vi "IonicsServiceTool.vi"() -> ()   [LabVIEW 2015]
uses:
  Type/_Source Type.ctl
  Type/_Syringe Pump Command.ctl
  Type/_Instrument Model.ctl
  Type/_RT Instrument State.ctl
  Type/_Run State.ctl
  Type/_Log Command.ctl
  Type/_RT Command.ctl
  Type/_RT Configuration 2.ctl
  Type/_PIC Channel.ctl
  Type/_RT Startup Options.ctl
  Type/_RT Instrument 2.ctl
  Type/_Data Operation.ctl
  Type/_Model Family.ctl
  Type/_SaveOption.ctl
  Type/_Board ID.ctl
  Type/_Run Module.ctl
  Type/_Voltage Type.ctl
  Print.ctl
  Type/_Pump Parameter.ctl
  Configuration/_Global Configuration.vi
  <vilib>/Utility/config.llb/Read Key (Path).vi
  <vilib>/Utility/config.llb/Write Key (Path).vi
  <vilib>/Utility/config.llb/Read Key (String).vi
  <vilib>/Utility/config.llb/Write Key (String).vi
  LCDriver/_Global LC Driver.vi
  <vilib>/Utility/config.llb/Read Key (I32).vi
  <vilib>/Utility/NIReport.llb/Append Image to Report (path wrap).vi
  <vilib>/Platform/browser.llb/Open URL in Default Browser (string).vi
  <vilib>/Utility/config.llb/Write Key (I32).vi
  <vilib>/Utility/NIReport.llb/NI_report.lvclass
  <vilib>/Utility/config.llb/NI_LVConfig.lvlib
panel:
  in  "Force Update Oscillators":bool
  out "Version":string
  out "Date/Time":string
  out "SN":string
  in  "Force Update Poles":bool
  out "MS State":T1
  in  "Print":bool
  in  "Options":bool
  in  "Unit":bool
  out "Firmware OK":bool
  out "Intlk/Per OK":bool
  out "Quad/Tune OK":bool=TRUE
  out "SVG OK":bool
  out "Voltage OK":bool
  out "Turbo OK":bool
  in  "Tab Control":T2(tab)
  out "*.ipf Path:":path=path "C:/GIT/EH-Simplicity/firmware-server/Sniffer.900/Ionica Server.ipf"
  in  "Header Info":bool
  out "IP Address":string="172.16.0.2"
  out "Corona":u16
  out "Source 2":u16
  out "Source 1":u16
  out "HSID":u16
  out "Model Name":T3=enum."Simulation (Single Source)"
  out "Serial Number":string="Ion Sniffer 03"
  in  "Refresh":bool
  out "Messages":string
  out "Description":string
  in  "Load Firmware":bool
  out "Current Information:":string[][](table)=[["FW Package Version", "0"], ["RT Firmware Version", "0"], ["FPGA Firmware Version", "0"], ["", ""], ["Instrument Serial #", "-1"], ["Instrument Model", "-1"]]
  out "Number of Power Failures:":u32
  out "Number of Pressure Overload Errors:":u32
  out "Total Number of Errors:":u32
  out "Errors:":string[][](table)=[["0", ""], ["", ""], ["", ""], ["", ""], ["", ""], ["", ""], ["", ""], ["", ""]]
  out "PumpStatus":u16(ring)
  out "Turning":bool
  out "Normal \nOperation":bool
  out "Accel":bool
  out "Decel":bool
  out "Frequency (Hz):":u16(slide) scale=0.0..1000.0
  out "Controller Temperature:":u16(slide) scale=0.0..90.0
  out "Moter Temperature:":u32(slide) scale=0.0..120.0
  out "Bearing Temperature:":u32(slide) scale=0.0..75.0
  out "Pressures:":string[][](table)=[["Foreline Pressure (torr)", "-0.11"], ["Analyzer Pressure (torr)", "1.00E+0"]]
  out "Run Time:":string[][](table)=[["Pump (hours)", ""], ["Days", ""], ["Number of Starts", ""], ["", ""], ["", ""], ["", ""], ["", ""], ["", ""]]
  out "Power:":string[][](table)=[["Voltage (V)", ""], ["Power (W)", ""], ["Current (A)", ""], ["Mean Current (A)", ""], ["Max Current (A)", ""], ["", ""], ["", ""], ["", ""]]
  out "Configuration:":string[][](table)=[["Pump Model", ""], ["Pump Serial Number", ""], ["Controller Model", ""], ["Controller Serial Number", ""], ["Electronics Model", ""], ["Electronic Serial Number", ""], ["Software Version", ""], ["Pump Parameter Set", ""]]
  in  "LBPower":bool
  in  "LBRunTime":bool
  in  "LBError":bool
  in  "LBConfiguration":bool
  in  "LBFreqTemp":bool
  in  "LBUpdateAll":bool
  in  "LBPump":bool
  in  "Update Power":bool
  in  "Update Temp":bool
  in  "Update Pumping":bool
  in  "Update Info":bool
  out "Error History":string[][](table)
  out "Temperatures:":string[][](table)=[["Electronic Drive Temperature", "Pass"], ["Pump Temperature", "Pass"], ["Power Stage Temperature (°C)", "0"], ["Electronics Temperature (°C)", "0"], ["Upper Pump Temperature (°C)", "0"], ["Bearing Temperature (°C)", "0"], ["Motor Temperature (°C)", "0"]]
  out "Power / Current:":string[][](table)=[["Drive Power (W)", "0"], ["Drive Current (A)", "0"]]
  out "Pumping:":string[][](table)=[["Rotational Frequency (Hz)", "0"], ["Rotational Speed (rpm)", "0"]]
  out "Pump Info:":string[][](table)=[["Hardware Version", "0"], ["Firmware Version", "0"], ["Operating Hours (Pump)", "0"], ["Operating Hours (Electronic Drive)", "0"]]
  in  "Turbo Update":bool
  out "Vacuum Readings by Region":string[][](table)=[["Foreline Pressure (torr)", "-0.11"], ["Analyzer Pressure (torr)", "1.00E+0"]]
  in  "Update Error":bool
  out "Main System Current (A)":dbl
  out "Lens Board 2 PS":i32(listbox)=-1
  in  "Set 0 Values":bool
  in  "Load Default Method":bool
  in  "Load Tune File":bool
  in  "Min Voltages":bool
  in  "Max Voltages":bool
  in  "Test Voltages":bool
  in  "Switch Polarity":bool
  out "Main System PS":i32(listbox)=-1
  out "Quad DC PS":i32(listbox)=-1
  out "Lens Board 1 PS":i32(listbox)=-1
  in  "Detector":string[][](table)=[["HED", "", "0.0", "3.014"], ["Horn", "", "0.0", "0.019"], ["DV", "", "0.0", "0.023"], ["Disc", "", "0.0", "2.014"], ["5", "L2 (11)", "0.0", "0.019"], ["6", "PF (12)", "-16.0", "0.019"], ["7", "CCL1 (13)", "0.0", "0.019"], ["8", "CCL2 (14)", "-100.0", "0.019"], ["9", "CC (23)", "-50.0", "0.014"], ["10", "CCAF (10)", "50.0", "0.019"], ["11", "CCL3 (15)", "-52.5", "0.014"], ["12", "CCL4 (16)", "-72.5", "0.014"], ["13", "ID (17)", "-100.0", "0.014"], ["14", "Horn (200)", "5500.0", "-82.090"], ["15", "DV (34)", "1000.0", "-82.773"], ["16", "M1RF (3)", "400.0", "2.161"], ["17", "Disc (32)", "10", "10"]]
  in  "Lens 1":string[][](table)=[["Element", "L1", "M1", "EV", "Spare", "M2", "CC", "Spare", "Spare"], ["Input", "0", "0", "0", "0", "0", "0", "0", "0"], ["Readback", "0", "0", "0", "0", "0", "0", "0", "0"]]
  in  "Lens 2":string[][](table)=[["Element", "CCAF", "L2", "PF", "CCL1", "CCL2", "CCL3", "CCL4", "ID"], ["Input", "", "", "", "", "", "", "", ""], ["Readback", "", "", "", "", "", "", "", ""]]
  out "Source Map":T4={"Ring 2"=0, "Ring 3"=0, "OK 2"=TRUE, "OK 3"=TRUE, "OK 4"=TRUE, "OK 5"=TRUE, "OK 6"=TRUE, "OK 7"=TRUE, "OK 8"=TRUE, "OK 9"=TRUE, "OK 10"=TRUE, "OK 11"=TRUE}
  out "Pressure Readings":string[][](table)=[["Foreline Pressure (torr)", "-0.11"], ["Analyzer Pressure (torr)", "1.00E+0"], ["Plenum Delta P (torr)", "-0.09"], ["Drying Gas Pressure (psi)", "-12.56"], ["Source Gas Pressure (psi)", "-12.56"]]
  in  "Corona/Curtain High Voltage":string[][](table)=[["Corona High Voltage", "0.0", "65535.000", "0"], ["Curtain Cap Voltage", "0.0", "910936.500", "0"]]
  in  "Source Probes":string[][](table)=[["Pillar 1", "None", "0.0", "2791790.869", "0"], ["Pillar 2", "None", "0.0", "2794412.334", "0"]]
  in  "Heaters":string[][](table)=[["1", "HSID", "200.0", "65535.000"], ["2", "P1T", "0.0", "93715.050"], ["3", "P2T", "0.0", "93715.050"]]
  in  "Typical Gas Settings":bool
  in  "Max Gas Settings":bool
  in  "Min Gas Settings":bool
  in  "Gas Flows":string[][](table)=[["1", "DG", "150.0", "316.460"], ["2", "NG1", "200.0", "312.782"], ["3", "HG1", "280.0", "354.817"], ["4", "NG2", "200.0", "0.000"], ["5", "HG2", "280.0", "0.000"], ["6", "CCP", "490", "-477.539"]]
  in  "GotoUPS":bool
  in  "IP Address":string
  in  "Input Value":sgl
  in  "Pump Command":T5=enum."status"
  out "Return Data":string
  in  "SendSyringeCommand":bool
  out "SourceOK":bool
  out "HG2OK":bool
  out "HG1OK":bool
  out "ExhaustOK":bool
  out "DryingGasOK":bool
  out "VacRdy":bool
  out "DoorOK":bool=TRUE
  out "Interlocks":string[][](table)=[["Card Cage Door", ""], ["Vacuum Ready", ""], ["Heating Gas 1", ""], ["Heating Gas 2", ""], ["Drying Gas", ""], ["Exhaust Gas", ""], ["Source Interlock", ""]]
  out "Source 2 Type:":T6=127 items=["None", "ESI", "APCI", "APPI", "MicroSpray"]
  out "Source 1 Type:":T6=127 items=["None", "ESI", "APCI", "APPI", "MicroSpray"]
  in  "FrequencyTuneSetup":bool
  out "Q2 RF Heat Sink Temperatures":string[][](table)=[["Q2 HS1", "-0.481"], ["Q2 HS2", "-0.481"], ["Q2 DC Pole A (18)", "-0.481"], ["Q2 DC Pole B (19)", "-0.481"]]
  out "Q1 RF Heat Sink Temperatures":string[][](table)=[["Q1 HS1", "-0.481"], ["Q1 HS2", "-0.481"], ["Q2 DC Pole A (18)", "-0.481"], ["Q2 DC Pole B (19)", "-0.481"]]
  out "M1 RF Heat Sink Temperatures":string[][](table)=[["M1 HS1", "-0.481"], ["M1 HS2", "-0.481"], ["Q2 DC Pole A (18)", "-0.481"], ["Q2 DC Pole B (19)", "-0.481"]]
  out "New Frequence":dbl=1.1064999969676137 format="%.4f"
  out "Old Frequency":dbl=1.1064999969676137 format="%.4f"
  in  "Adjust Cal Tables":bool
  out "M1RF Readback":dbl
  in  "M1RF":dbl=400.0 format="%#.3f"
  in  "Update PM":bool
  in  "Q2 Park Mass":dbl=400.0 format="%#.3f"
  in  "Q1 Park Mass":dbl=400.0 format="%#.3f"
  out "Q2 Total":dbl=157.94015025000002
  out "Q1 Total":dbl=157.94015025000002
  out "Q2 (VDC)":dbl=157.94015025000002
  out "Q1 (VDC)":dbl=157.94015025000002
  in  "Q2 DC Inputs":string[][](table)=[["600.00"], ["0.00"], ["0.00"]]
  in  "Q1 DC Inputs":string[][](table)=[["600.00"], ["0.00"], ["0.00"]]
  out "DC Pole Read Back":string[][](table)=[["Q1 DC Pole A", "-0.481"], ["Q1 DC Pole B", "-0.481"], ["Q2 DC Pole A", "-0.481"], ["Q2 DC Pole B", "-0.481"]]
  in  "Oscillator Settings":string[][](table)=[["M1RF", "66529043", "10", "10", "0.4", "1.5490", "2.256", "1.5490"], ["Q1RF", "47523813", "10", "10", "0.6", "1.1065", "-0.645", "1.1065"], ["Q2RF", "47523813", "10", "10", "0.6", "1.1065", "7.339", "1.1065"]]
  in  "Pos/Neg":enum32{"Positive", "Negative"}(radio)
  in  "Pole Swap Options Negative":T7
  in  "Pole Swap Options Positive":T7
  in  "Table Choice":T8(radio)
  out "Table 4":T9 caption="Q2 -ve Mass Calibration Table"
  out "Table 2":T9 caption="Q2 +ve Mass Calibration Table"
  out "Table 3":T9 caption="Q1 -ve Mass Calibration Table"
  out "Table 1":T9 caption="Q1 +ve Mass Calibration Table"
  in  "Edit Config":bool
  in  "Edit ADC":bool
  in  "View Config":bool
  in  "Export ADC":bool
  out "ADC List":i32(listbox)=130
  in  "Run":bool
  in  "Cancel":bool
  out "Progress Bar":u8(slide)=1 scale=0.0..100.0
  out "LoadedTable":bool
  in  "Tune File":path=path "C:/GIT/EH-Simplicity/firmware-server/Sniffer.900/InternalTools/DEFAULT_SETTINGS.d2m"
  in  "SG Input":dbl[](array[numeric])=[40.0, 0.0, 0.0, 0.0, 0.0, 0.0, 0.0, 200.0, 0.0, 0.0, 0.0, 0.0, 0.0, 0.0]
  in  "VoltageInput":dbl[](array[numeric])=[0.0, 0.0, 0.0, 0.0, 0.0, -16.0, 0.0, -100.0, -50.0, 50.0, -52.5, -72.5, -100.0, 5500.0, 1000.0, 400.0, 10.0, 0.0, 0.0]
  out "Quit":bool=TRUE
  out "Running":bool
  out "Ion Path":T10={"OK 1"=TRUE, "OK 2"=TRUE, "OK 3"=TRUE, "OK 4"=TRUE, "OK 5"=TRUE, "OK 6"=TRUE, "OK 7"=TRUE, "OK 8"=TRUE, "OK 9"=TRUE, "OK 10"=TRUE, "OK 15"=TRUE, "OK 20"=TRUE, "OK 16"=TRUE, "OK 11"=TRUE, "OK 17"=TRUE, "OK 18"=TRUE, "OK 19"=TRUE, "OK 12"=TRUE, "OK 13"=TRUE, "Selected 1"="Selected", "Selected 2"="Selected", "Selected 3"="Selected", "Selected 4"="Selected", "Selected 5"="Selected", "Selected 6"="Selected", "Selected 7"="Selected", "Selected 8"="Selected", "Selected 9"="Selected", "Selected 10"="Selected", "Selected 15"="Selected", "Selected 20"="Selected", "Selected 16"="Selected", "Selected 11"="Selected", "Selected 17"="Selected", "Selected 18"="Selected", "Selected 19"="Selected", "Selected 12"="Selected", "Selected 13"="Selected", "Ring 2"=0, "Ring 3"=0, "OK 14"=TRUE, "Selected 14"="Selected"}
  out "IonPathMap":enum32{"0", "200", "100"}(tab)
  # "PIC Firmware Version"
  # "It will take about 70s\nto complete Update All."
  # "Syringe Pump Control"
  # "UPS"
  # "V"
  # "Polarity"
  # "Pole Orientation"
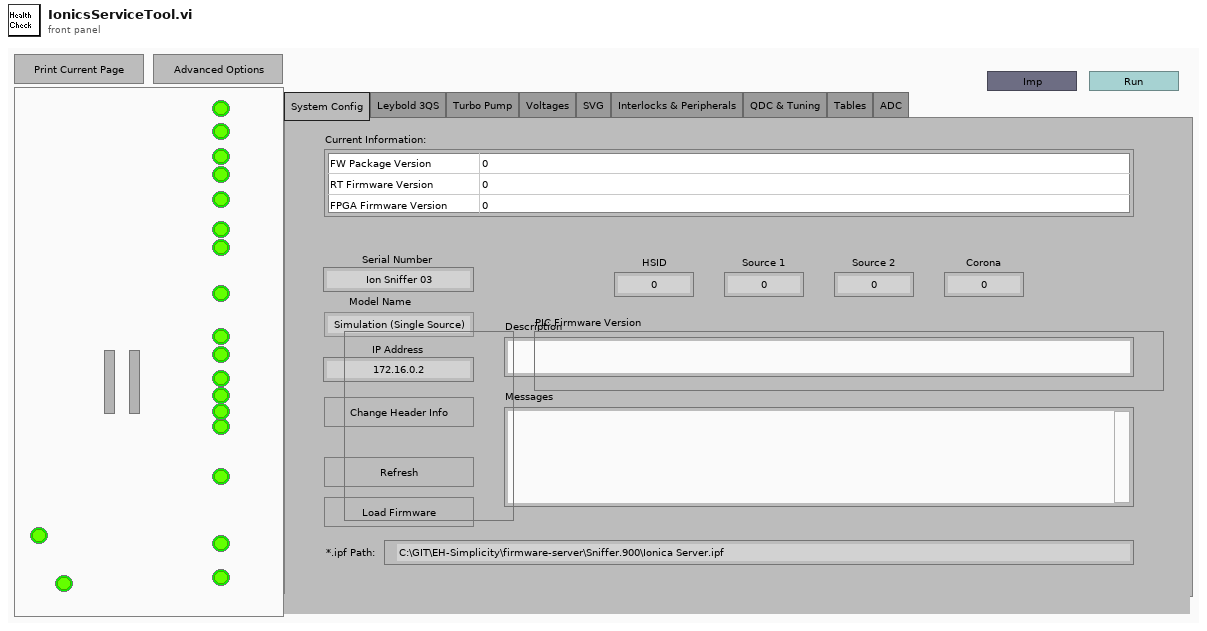
[diagram p1: front panel]
types:
  T1 = typedef "_RT Instrument State.ctl" = enum16{"Initializing", "Mass Spectrometer is Off", "Starting Up", "Turning Power Off", "Going to Standby", "Roughing Pump Ready", "Turning Turbo Off", "Turbo Startup", "Turbopump Ready", "Checking Vacuum", "Going to Ready", "Ready", "Running", "Source Standby", "Lost Communication", "Shutting Down", "Fault", "24V Standby", "Go to 24V Standby", "Turbopump Ready-Waiting"}
  T2 = enum32{"System Config", "Leybold 3QS", "Turbo Pump", "Voltages", "SVG", "Interlocks & Peripherals", "QDC & Tuning", "Tables", "ADC"}
  T3 = typedef "_Instrument Model.ctl" = enum16{"QSight 110", "QSight 120", "QSight 210", "QSight 220", "IONICS 3Q 110", "IONICS 3Q 120", "IONICS 3Q 210", "IONICS 3Q 220", "IONICS 3Q 310", "IONICS 3Q 320", "Simulation (Single Source)", "Simulation (Dual Source)"}
  T4 = cluster{"Ring 2":u16, "Ring 3":u16, "OK 2":bool, "OK 3":bool, "OK 4":bool, "OK 5":bool, "OK 6":bool, "OK 7":bool, "OK 8":bool, "OK 9":bool, "OK 10":bool, "OK 11":bool}
  T5 = typedef "_Syringe Pump Command.ctl" = enum16{"start", "stop", "pause", "restart", "help", "set units", "set diameter", "set rate", "set time", "set volume", "set delay", "save setting", "read limit parameter", "view parameter", "status"}
  T6 = typedef "_Source Type.ctl" = i8
  T7 = cluster{"Q1 A":bool, "Q1 B":bool, "Q2 A":bool, "Q2 B":bool}
  T8 = enum32{"Calibration", "Low Resolution", "Unit Resolution", "High Resolution"}
  T9 = cluster{"Graph":cluster{"all rows":dbl[], "all rows":dbl[]}, "Table":string[][]}
  T10 = cluster{"OK 1":bool, "OK 2":bool, "OK 3":bool, "OK 4":bool, "OK 5":bool, "OK 6":bool, "OK 7":bool, "OK 8":bool, "OK 9":bool, "OK 10":bool, "OK 15":bool, "OK 20":bool, "OK 16":bool, "OK 11":bool, "OK 17":bool, "OK 18":bool, "OK 19":bool, "OK 12":bool, "OK 13":bool, "Selected 1":string, "Selected 2":string, "Selected 3":string, "Selected 4":string, "Selected 5":string, "Selected 6":string, "Selected 7":string, "Selected 8":string, "Selected 9":string, "Selected 10":string, "Selected 15":string, "Selected 20":string, "Selected 16":string, "Selected 11":string, "Selected 17":string, "Selected 18":string, "Selected 19":string, "Selected 12":string, "Selected 13":string, "Ring 2":u16, "Ring 3":u16, "OK 14":bool, "Selected 14":string}
  T11 = enum32{"invalid app kind", "Development System", "Run Time System", "Student Edition", "Embedded LabVIEW", "Evaluation", "Custom"}
  T12 = enum8{"Enabled", "Disabled", "Disabled and Grayed Out"}
  T13 = typedef "_Run State.ctl" = enum16{"Init", "Update", "Start", "End", "Error"}
  T14 = typedef "_Log Command.ctl" = enum16{"No Command", "Open", "Read", "Write", "Close", "Check Size"}
  T15 = typedef "_RT Command.ctl" = enum16{"xml Start Run", "xml Start Actual Run", "xml Stop Run", "xml Runtime Update", "xml Get Status", "xml Get Table", "xml Set Table", "xml Get Configuration", "xml System Status", "xml Set LC Input Logic", "xml Get Data", "xml Get Info", "Start", "StartActualRun", "Stop", "Runtime Update", "Get Data", "Get Info", "Get Status", "Get Param", "Get Config", "Get Table", "Read ADC", "Set Oscillator", "Update Config", "Update Table", "Set All Pol", "Set Pol and DC", "Set Max Mass", "Toggle RP", "Toggle EL", "Set PIC", "Initialize Turbo", "Send Turbo Comm", "Close Turbo", "P1", "P2", "P3", "Send Serial", "Set LC Out", "Get LC In", "Read VAC", "Test Table", "Toggle Power", "Get Startup", "Set Startup", "Get ADC Table", "Set ADC Table", "Get Brief Status", "Get Detail Status", "Auxiliary Update", "Set CC Logics", "Set CC Input Logics", "Ignore Error", "invalid"}
  T16 = enum16{"Use Dialog", "Temporary File", "My Tables"}
  T17 = typedef "_PIC Channel.ctl" = enum16{"Corona +HV", "Corona -HV", "HSID Temp", "Time Const 1", "Curtain Cap +HV", "Curtain Cap -HV", "Time Const 2", "Source 1 +HV", "Source 1 -HV", "Source 1 Temp", "Time Const 3", "Source 2 +HV", "Source 2 -HV", "Source 2 Temp", "Time Const 4"}
  T18 = typedef "_RT Instrument 2.ctl" = cluster{"Table":T19[], "Instrument":string[]}
  T19 = typedef "_RT Configuration 2.ctl" = cluster{"Name":string, "Ch#":u8, "Min":dbl, "Max":dbl, "Def+":dbl, "Def-":dbl, "Offset":dbl, "Slope":dbl, "Type":u8, "Description":string, "SettleT":dbl}
  T20 = cluster{"top":dbl, "left":dbl, "right":dbl, "bottom":dbl}
  T21 = typedef "Print.ctl" = cluster{"Picture Name":string, "VI Reference":refnum<vi>}
  T22 = enum16{"Standard Report", "HTML", "Word", "Excel"}
  T23 = typedef "_Data Operation.ctl" = enum8{"Initialize", "Get Data", "Set Data", "Close"}
  T24 = typedef "_SaveOption.ctl" = enum16{"Use Dialog", "Temporary File", "My Tables", "Full Path"}
  T25 = typedef "_Pump Parameter.ctl" = enum16{"Turn Pump Motor On", "Turn Pump Motor Off", "Read Pump Oil Deficiency", "Read Rotation Switch Point Attained", "Read Ele. Drive Over Temperature", "Read Pump Over Temperature", "Read Set Rotation Speed Attained", "Read Turbopump Accelerates", "Read Actual Rotation Speed in Hz", "Read Motor Current in A", "Read Operating Hours in h", "Read Motor Voltage in V", "Read Motor Power in W", "Set Rotation Speed Switchpoint in %", "Clear Error", "Read Error Code", "Read Bearing Temperature", "Read Hardware Version", "Read Firmware Version", "Read Operating Hours (Drive)", "Read Rotational Speed (rpm)", "Read Power Stage Temperature", "Read Electronics Temperature", "Read Upper Pump Temperature", "Read Motor Temperature", "Read Error Code History, 1", "Read Error Code History, 2", "Read Error Code History, 3", "Read Error Code History, 4", "Read Error Code History, 5", "Read Error Code History, 6", "Read Error Code History, 7", "Read Error Code History, 8", "Read Error Code History, 9", "Read Error Code History, 10"}
  T26 = enum32{"existing file", "new file", "new or existing file", "existing dir", "new dir", "new or existing dir", "existing file (use LLBs)", "new file (use LLBs)", "new or existing file (use LLBs)", "new or existing file or directory (use LLBs)"}
  T27 = enum32{"Leybold 3QS", "Pfeiffer Pump", "Voltages", "SVG", "Interlocks & Peripherals", "FW Manager", "QDC & Tuning", "Tables", "ADC"}
  T28 = cluster{"Source Map":refnum<vi>, "Ion Path":refnum<vi>, "Lens 1":refnum<vi>, "Lens 2":refnum<vi>, "Detector":refnum<vi>, "Main System PS":refnum<vi>, "Lens Board 1 PS":refnum<vi>, "Quad DC PS":refnum<vi>, "Gas Flows":refnum<vi>, "Heaters":refnum<vi>, "Source Probes":refnum<vi>, "Corona/Curtain High Voltage":refnum<vi>, "Pressure Readings":refnum<vi>, "DC Pole Read Back":refnum<vi>, "Lens Board 2 PS":refnum<vi>, "M1 RF Heat Sink Temperatures":refnum<vi>, "Q1 RF Heat Sink Temperatures":refnum<vi>, "Q2 RF Heat Sink Temperatures":refnum<vi>}
  T29 = typedef "NI_LVConfig.lvlib/Config Data RefNum.ctl" = refnum<k1>
  T30 = typedef "_LC Type.ctl" = enum16{"No LC", "Spark"}
  T31 = typedef "_RT Startup Options.ctl" = cluster{"Door":bool, "Curtain":bool, "Pressure":bool, "Turbo":bool, "SysPoll":bool, "GasFlag":bool, "SourceExhaust":bool}
  T32 = cluster{"Configuration 2":T18, "FrequencyTune":bool, "CalAjusted":bool, "Update":bool, "Running":bool, "ADC Table":T19[]}
  T33 = typedef "_Model Family.ctl" = u16
  T34 = typedef "_Board ID.ctl" = u16
  T35 = typedef "_Run Module.ctl" = u16
  T36 = cluster{"trimmed string":string, string, "selected path":path, "Source":enum32{"RT Target", "Folder"}}
  T37 = typedef "_Voltage Type.ctl" = u16
  T38 = cluster{"Frequency":u16, "Decel":bool, "Accel":bool, "Normal \nOperation":bool, "Turning":bool, "BearingTemp":u32, "MotorTemp":u32, "ControllerTemp":u16, "PumpStatus":u16, "NumErrors":u32, "NumOverload":u32, "NumFailure":u32}
  T39 = typedef "imagedata.ctl" = cluster{"image type":i32, "image depth":i32, "image":u8[], "mask":u8[], "colors":u32[], "Rectangle":cluster{"left":i16, "top":i16, "right":i16, "bottom":i16}}
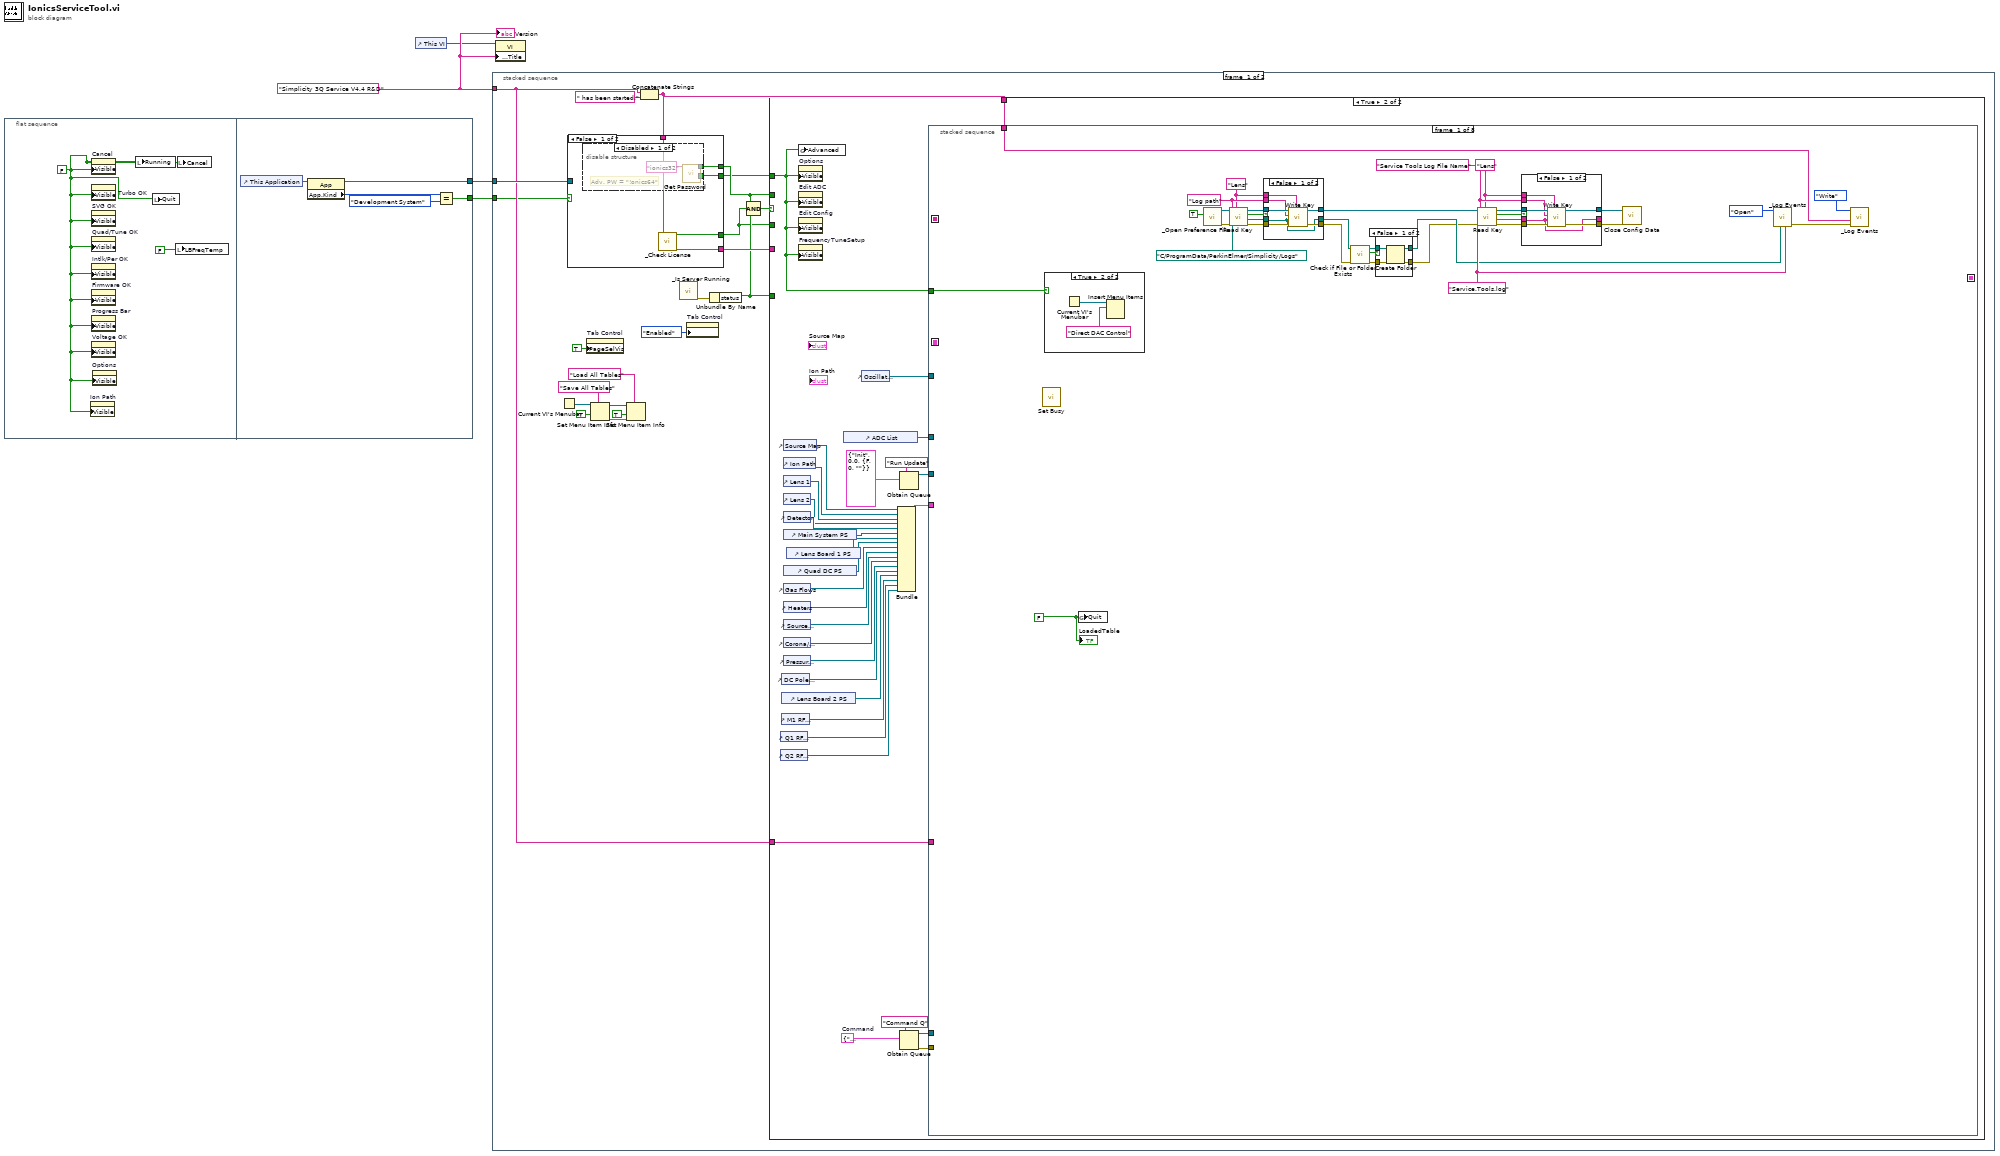
[diagram p0: block diagram]
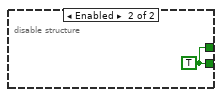
[diagram p2: hidden frame]
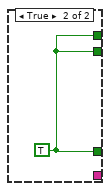
[diagram p3: hidden frame]
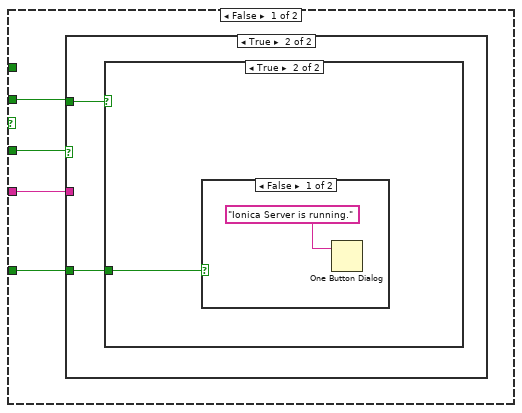
[diagram p4: hidden frame]
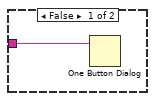
[diagram p5: hidden frame]
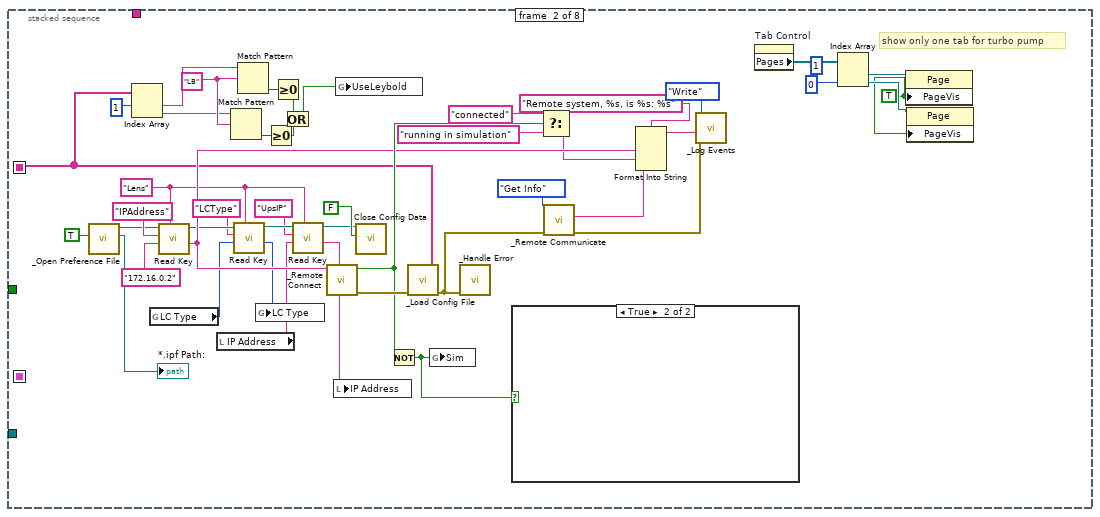
[diagram p12: hidden frame]
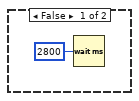
[diagram p13: hidden frame]
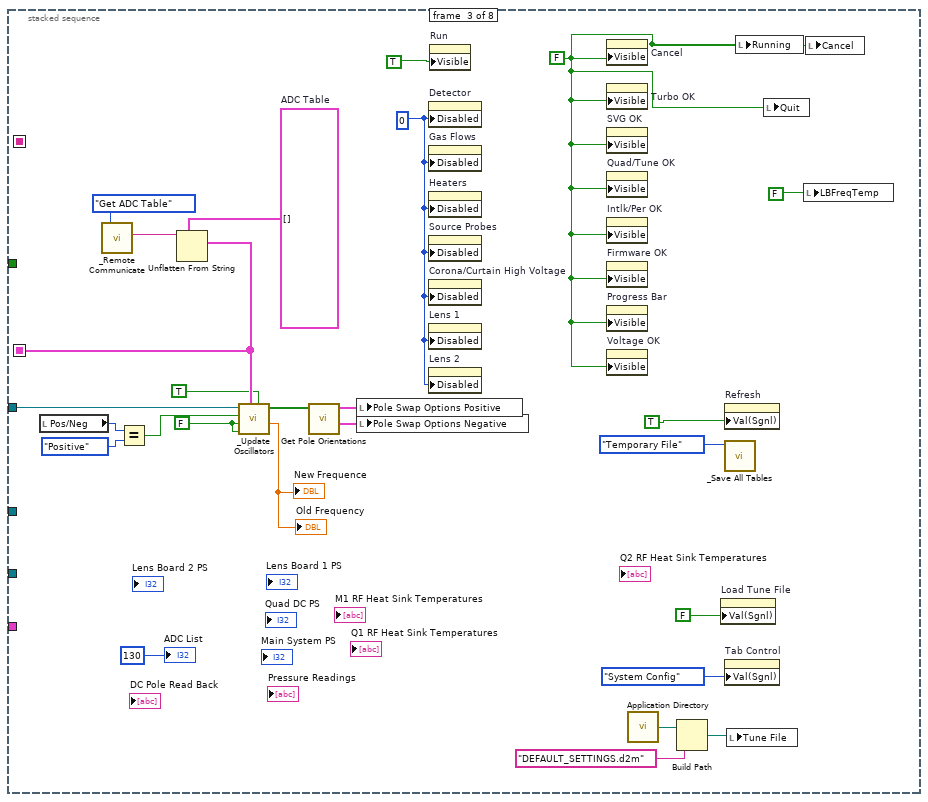
[diagram p14: hidden frame]
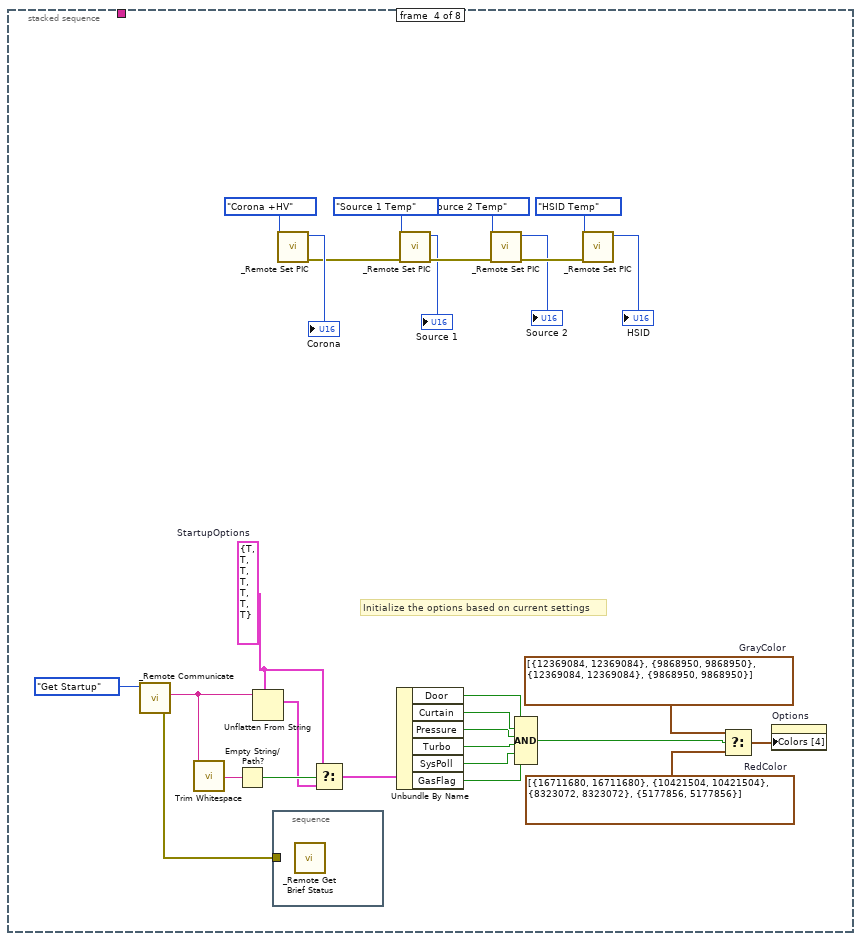
[diagram p15: hidden frame]
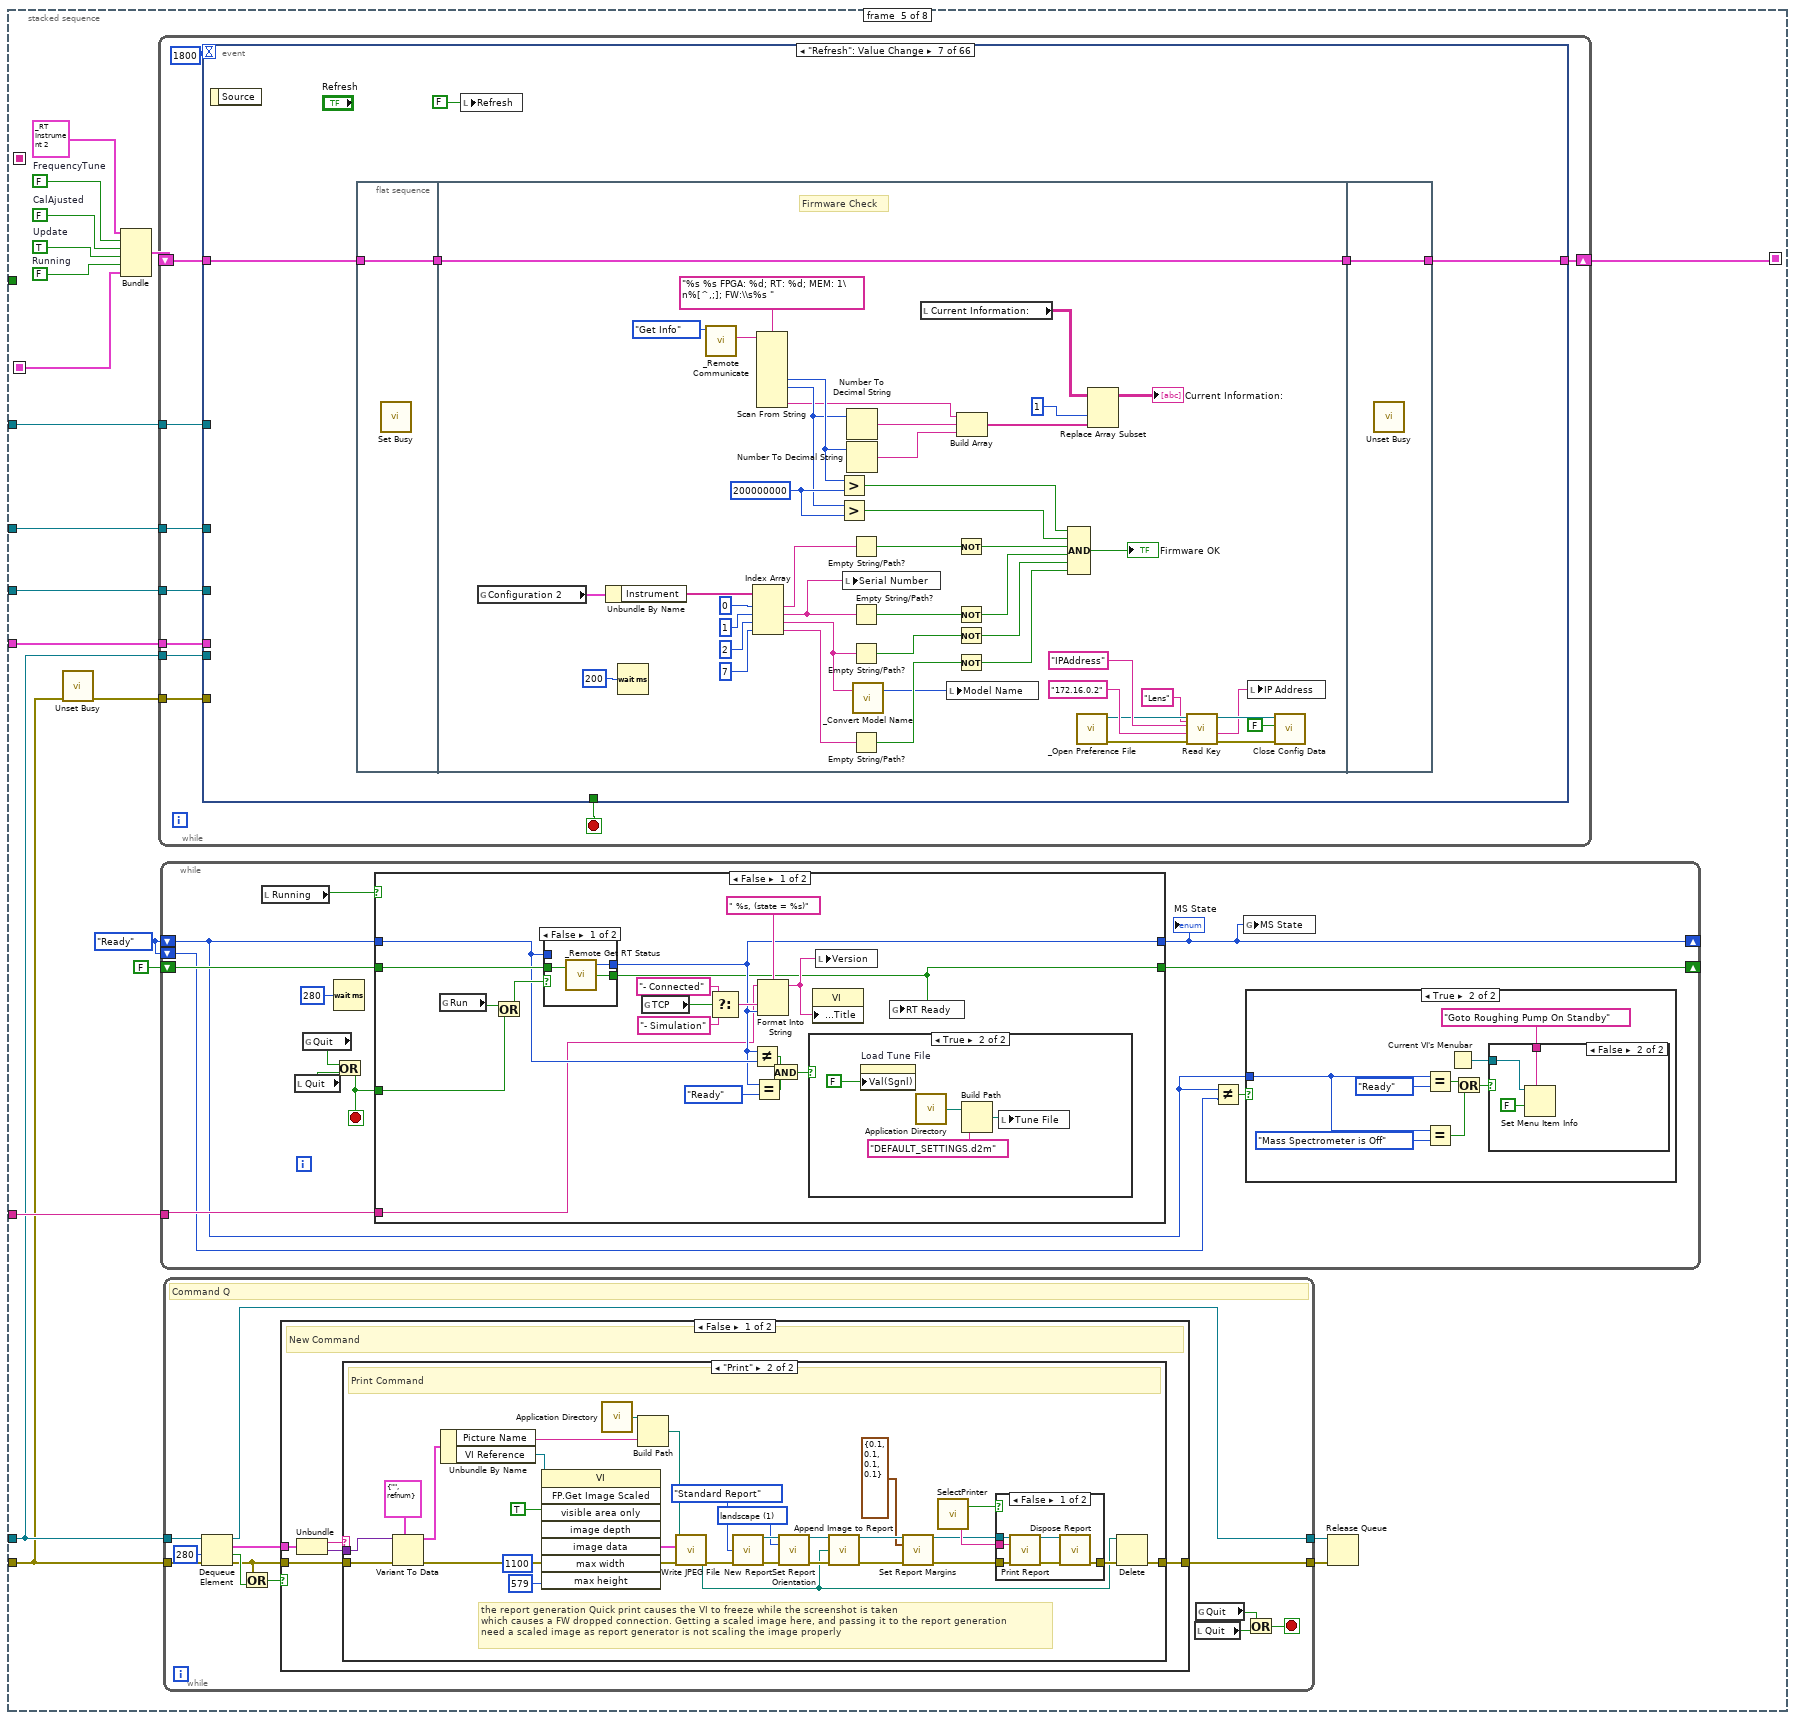
[diagram p16: hidden frame]
diagram:
  w2 = "Simplicity 3Q Service V4.4 R&D" ("string")
  n1 = flat-sequence {
    tunnel: [w9] -> w4
    tunnel: [w8] -> w3
    frame #0 {
      w5 = FALSE ("Unit")
      n2 = property on="Ion Path" class="Clust (strict)"("Visible"=w5) -> ()  [unwired: 2 in, 2 out]
      n3 = property on="Cancel" class="Bool (strict)"("Visible"=w5) -> ()  [unwired: 2 in, 2 out]
      n4 = property on="Turbo OK" class="Bool (strict)"("Visible"=w5) -> ()  [unwired: 2 in, 2 out]
      n5 = property on="SVG OK" class="Bool (strict)"("Visible"=w5) -> ()  [unwired: 2 in, 2 out]
      n6 = property on="Quad/Tune OK" class="Bool (strict)"("Visible"=w5) -> ()  [unwired: 2 in, 2 out]
      n7 = property on="Intlk/Per OK" class="Bool (strict)"("Visible"=w5) -> ()  [unwired: 2 in, 2 out]
      n8 = property on="Firmware OK" class="Bool (strict)"("Visible"=w5) -> ()  [unwired: 2 in, 2 out]
      n9 = property on="Progress Bar" class="Slide (strict)"("Visible"=w5) -> ()  [unwired: 2 in, 2 out]
      n10 = property on="Voltage OK" class="Bool (strict)"("Visible"=w5) -> ()  [unwired: 2 in, 2 out]
      n11 = property on="Options" class="Bool"("Visible"=w5) -> ()  [unwired: 2 in, 2 out]
      n12 = local write "Running"(w5) -> ()
      n13 = local write "Quit"(w5) -> ()
      n14 = local write "LBFreqTemp"(FALSE ("LBFreqTemp")) -> ()
      n15 = local write "Cancel"(w5) -> ()
    }
    frame #1 {
      n16 = control-ref of="This Application"() -> (w7:refnum<vi>)
      n17 = property class="App"(reference=w7) -> (reference out=w8:refnum<vi>, "App.Kind"=w10:T11)  [unwired: 1 in, 1 out]
      n18 = Equal?(x=w10, y=T11."Development System") -> (x = y?=w9:bool)
    }
  }
  n19 = control-ref of="This VI"() -> (w1:refnum<vi>)
  n20 = stacked-sequence {
    tunnel: w4 -> [w12 w1712]
    tunnel: w3 -> [w25 _]
    tunnel: w2 -> [w22 _]
    frame #0 {
      n21 = Current VI's Menubar() -> (w19:refnum<k9>)
      n22 = property on="Tab Control" class="TabCtl (strict)"("PageSelVis"=TRUE ("Page Selector Visible")) -> ()  [unwired: 2 in, 2 out]
      n23 = Set Menu Item Info(7:"Save All Tables" ("item tag"), 9:TRUE ("enabled"), 11:w19) -> (0:w15:errorcluster, 3:w16:refnum<k9>)  [unwired: 4 in]
      n24 = Set Menu Item Info(7:"Load All Tables" ("item tag"), 8:w15, 9:TRUE ("enabled"), 11:w16) -> ()  [unwired: 3 in, 2 out]
      n25 = Concatenate Strings(w22, " has been started." ("string")) -> (w24:string)
      n26 = case shown="False" w12 {
        tunnel: w24 -> [w37 _]
        tunnel: [w36 _] -> w31
        tunnel: [w35 w42] -> w30
        tunnel: [w34 w42] -> w29
        tunnel: [w33 w42] -> w26
        tunnel: w25 -> [_ _]
        frame False {
          n27 = disable-structure shown="Disabled" {
            disable-tunnel: [w39 w41] -> w35
            disable-tunnel: [w38 w41] -> w34
            frame Disabled {
              # "Adv. PW = \"!onics64\""
              n28 = call "Get Password.vi"("IonSniffer777"="ionics32") -> ("Advanced"=w38:bool, "Valid"=w39:bool)  [unwired: 5 out]
            }
            frame Enabled {
              w41 = TRUE ("Advanced")
            }
          }
          n29 = call "_Check License.vi"("ApplicationName"=w37) -> ("Reason"=w36:string, "Valid"=w33:bool)  [unwired: 5 out]
        }
        frame True {
          w42 = TRUE ("Valid")
        }
      }
      n30 = call "_Is Server Running.vi"() -> ("error out"=w28:errorcluster)  [unwired: 6 in, 1 out]
      n31 = property on="Tab Control" class="TabCtl (strict)"("DisabledEnum"=T12."Enabled" ("Disabled")) -> ()  [unwired: 2 in, 2 out]
      n32 = Unbundle By Name(w28) -> ("status"=w27:bool)
      n33 = Compound Arithmetic op=AND(w30, w26, w27) -> (w32:bool)
      n34 = case shown="True" w32 {
        tunnel: w24 -> [_ w66]
        tunnel: w26 -> [w46 _]
        tunnel: w31 -> [w45 _]
        tunnel: w30 -> [w44 _]
        tunnel: w29 -> [_ w57]
        tunnel: w27 -> [w43 _]
        tunnel: w22 -> [_ w56]
        frame False {
          n35 = case shown="True" w46 {
            tunnel: w45 -> [w47 _]
            tunnel: w44 -> [_ w49]
            tunnel: w43 -> [_ w48]
            frame False {
              n36 = One Button Dialog(message=w47) -> ()  [unwired: 2 out]
            }
            frame True {
              n37 = case shown="True" w49 {
                tunnel: w48 -> [_ w50]
                frame False {
                }
                frame True {
                  n38 = case shown="False" w50 {
                    frame False {
                      n39 = One Button Dialog(message="Ionica Server is running.") -> ()  [unwired: 2 out]
                    }
                    frame True {
                    }
                  }
                }
              }
            }
          }
        }
        frame True {
          w54 = cluster{"Command":string, "Data":variant} {"Command"="", "Data"=variant}  # Command
          n40 = control-ref of="Q1 RF Heat Sink Temperatures"() -> (w59:refnum<vi>)
          n41 = control-ref of="Q2 RF Heat Sink Temperatures"() -> (w58:refnum<vi>)
          n42 = control-ref of="Lens Board 2 PS"() -> (w61:refnum<vi>)
          n43 = control-ref of="DC Pole Read Back"() -> (w67:refnum<vi>)
          n44 = control-ref of="M1 RF Heat Sink Temperatures"() -> (w60:refnum<vi>)
          n45 = control-ref of="Ion Path"() -> (w63:refnum<vi>)
          n46 = control-ref of="Lens 1"() -> (w64:refnum<vi>)
          n47 = control-ref of="Lens 2"() -> (w65:refnum<vi>)
          n48 = control-ref of="Detector"() -> (w79:refnum<vi>)
          n49 = control-ref of="Main System PS"() -> (w78:refnum<vi>)
          n50 = control-ref of="Quad DC PS"() -> (w77:refnum<vi>)
          n51 = control-ref of="Gas Flows"() -> (w73:refnum<vi>)
          n52 = control-ref of="Heaters"() -> (w72:refnum<vi>)
          n53 = control-ref of="Source Probes"() -> (w71:refnum<vi>)
          n54 = control-ref of="Corona/Curtain High Voltage"() -> (w70:refnum<vi>)
          n55 = control-ref of="Pressure Readings"() -> (w69:refnum<vi>)
          n56 = control-ref of="Source Map"() -> (w62:refnum<vi>)
          n57 = control-ref of="Lens Board 1 PS"() -> (w76:refnum<vi>)
          n58 = global write "_Global Configuration.vi" "Advanced"(w57) -> ()
          n59 = property on="Options" class="Bool"("Visible"=w57) -> ()  [unwired: 2 in, 2 out]
          n60 = property on="Edit ADC" class="Bool"("Visible"=w57) -> ()  [unwired: 2 in, 2 out]
          n61 = property on="Edit Config" class="Bool"("Visible"=w57) -> ()  [unwired: 2 in, 2 out]
          n62 = property on="FrequencyTuneSetup" class="Bool (strict)"("Visible"=w57) -> ()  [unwired: 2 in, 2 out]
          n63 = control-ref of="ADC List"() -> (w74:refnum<vi>)
          n64 = control-ref of="Oscillator Settings"() -> (w68:refnum<vi>)
          n65 = Bundle("Source Map"=w62, "Ion Path"=w63, "Lens 1"=w64, "Lens 2"=w65, "Detector"=w79, "Main System PS"=w78, "Lens Board 1 PS"=w76, "Quad DC PS"=w77, "Gas Flows"=w73, "Heaters"=w72, "Source Probes"=w71, "Corona/Curtain High Voltage"=w70, "Pressure Readings"=w69, "DC Pole Read Back"=w67, "Lens Board 2 PS"=w61, "M1 RF Heat Sink Temperatures"=w60, "Q1 RF Heat Sink Temperatures"=w59, "Q2 RF Heat Sink Temperatures"=w58) -> (w75:T28)  [unwired: 1 out]
          n66 = Obtain Queue(name (unnamed)="Run Update", element data type=cluster{T13, dbl, "error out":errorcluster} {enum."Init", 0.0, "error out"={"status"=FALSE, "code"=0, "source"=""}}) -> (queue out=w80:refnum<queue>)  [unwired: 3 in, 2 out]
          n67 = Obtain Queue(name (unnamed)="Command Q", element data type=w54) -> (queue out=w53:refnum<queue>, error out=w52:errorcluster)  [unwired: 3 in, 1 out]
          n68 = stacked-sequence {
            seq-local: [_ _ w209 _ _ _ _ _] -> [_ _ _ _ w257 _ _ _]
            seq-local: [_ w160 _ _ _ _ _ _] -> [_ _ _ _ _ w1652 _ _]
            seq-local: [_ _ _ _ w255 _ _ _] -> [_ _ _ _ _ w1596 _ _]
            tunnel: w80 -> [_ _ _ _ w265 w1658 _ _]
            tunnel: w75 -> [_ _ _ _ w261 _ _ _]
            tunnel: w74 -> [_ _ _ _ w260 _ _ _]
            tunnel: w68 -> [_ _ w214 _ w259 _ _ _]
            tunnel: w66 -> [w83 _ _ _ _ _ _ _]
            tunnel: w57 -> [w114 _ _ _ _ _ _ _]
            tunnel: w56 -> [_ _ _ _ w252 _ _ _]
            tunnel: w53 -> [_ _ _ _ w251 _ _ _]
            tunnel: w52 -> [_ _ _ _ w248 _ _ _]
            frame #0 {
              w113 = "Service.Tools.log" ("default value")
              w103 = "Service Tools Log File Name" ("key")
              w102 = "Lens" ("section")
              w97 = "Log path" ("key")
              w96 = "Lens" ("section")
              w115 = FALSE ("Quit")
              n69 = call <vilib>:"Set Busy.vi"() -> ()  [unwired: 4 in, 8 out]
              n70 = case shown="True" w114 {
                frame False {
                }
                frame True {
                  n71 = Current VI's Menubar() -> (w143:refnum<k9>)
                  n72 = Insert Menu Items(8:"Direct DAC Control", 9:w143) -> ()  [unwired: 4 in, 3 out]
                }
              }
              n73 = global write "_Global Configuration.vi" "Quit"(w115) -> ()
              n74 = call "_Open Preference File.vi"("Initialize"=TRUE) -> ("error"=w89:errorcluster, "refnum"=w90:T29)  [unwired: 2 in, 3 out]
              n75 = call-poly <vilib>:"Read Key.vi"("section"=w96, "error in (no error)"=w89, "default value"=path "C:/ProgramData/PerkinElmer/Simplicity/Logs", "key"=w97, "refnum"=w90) -> ("error out"=w91:errorcluster, "value"=w93:path, "found?"=w92:bool, "refnum out"=w94:T29)  [unwired: 3 in]
              n76 = case shown="False" w92 {
                tunnel: w91 -> [w138 w141]
                tunnel: w93 -> [w132 w139]
                tunnel: w94 -> [w136 w140]
                tunnel: [w137 w141] -> w110
                tunnel: [w135 w140] -> w95
                tunnel: [w132 w139] -> w111
                tunnel: w96 -> [w134 _]
                tunnel: w97 -> [w133 _]
                frame False {
                  n77 = call-poly <vilib>:"Write Key.vi"("section"=w134, "error in (no error)"=w138, "value"=w132, "key"=w133, "refnum"=w136) -> ("error out"=w137:errorcluster, "refnum out"=w135:T29)  [unwired: 4 in, 1 out]
                }
                frame True {
                }
              }
              n78 = call <vilib>:"Check if File or Folder Exists.vi"("error in (no error)"=w110, "path"=w111) -> ("error out"=w106:errorcluster, "file or folder exists?"=w108:bool, "dup path"=w107:path)  [unwired: 7 in]
              n79 = case shown="False" w108 {
                tunnel: w106 -> [w119 w120]
                tunnel: w107 -> [w118 w121]
                tunnel: [w117 w121] -> w112
                tunnel: [w116 w120] -> w109
                frame False {
                  n80 = Create Folder(path (use dialog)=w118, error in=w119) -> (created path=w117:path, error out=w116:errorcluster)  [unwired: 1 in, 1 out]
                }
                frame True {
                }
              }
              n81 = call-poly <vilib>:"Read Key.vi"("section"=w102, "error in (no error)"=w109, "default value"=w113, "key"=w103, "refnum"=w95) -> ("error out"=w101:errorcluster, "value"=w100:string, "found?"=w99:bool, "refnum out"=w98:T29)  [unwired: 3 in]
              n82 = case shown="False" w99 {
                tunnel: w101 -> [w128 w131]
                tunnel: w100 -> [w122 w129]
                tunnel: w98 -> [w126 w130]
                tunnel: [w127 w131] -> w105
                tunnel: [w125 w130] -> w104
                tunnel: [w122 w129] -> _
                tunnel: w102 -> [w124 _]
                tunnel: w103 -> [w123 _]
                frame False {
                  n83 = call-poly <vilib>:"Write Key.vi"("section"=w124, "error in (no error)"=w128, "value"=w122, "key"=w123, "refnum"=w126) -> ("error out"=w127:errorcluster, "refnum out"=w125:T29)  [unwired: 4 in, 1 out]
                }
                frame True {
                }
              }
              n84 = call <vilib>:"Close Config Data.vi"("error in (no error)"=w105, "refnum"=w104) -> ()  [unwired: 1 in, 9 out]
              n85 = call "_Log Events.vi"("File Name"=w113, "Log Path"=w112, "Log Command"=_Log_Command."Open" ("File Command")) -> ("error out"=w86:errorcluster)  [unwired: 5 in, 1 out]
              n86 = call "_Log Events.vi"("error in (no error)"=w86, "Event"=w83, "Log Command"=_Log_Command."Write" ("File Command")) -> ()  [unwired: 5 in, 2 out]
              "LoadedTable" <- w115
            }
            frame #1 {
              w144 = TRUE ("Page Visible")
              w156 = "LB" ("regular expression")
              w163 = "Lens" ("section")
              # "show only one tab for turbo pump"
              n87 = call "_Open Preference File.vi"("Initialize"=TRUE) -> ("ipf path"=→"*.ipf Path:":path, "refnum"=w173:T29)  [unwired: 2 in, 3 out]
              n88 = global read "_Global LC Driver.vi" "LC Type"() -> (w169:T30)
              n89 = call-poly <vilib>:"Read Key.vi"("section"=w163, "default value"="172.16.0.2", "key"="IPAddress" ("section"), "refnum"=w173) -> ("value"=w183:string, "refnum out"=w170:T29)  [unwired: 2 in, 4 out]
              n90 = local read "IP Address"() -> (w162:string)
              n91 = call-poly <vilib>:"Read Key.vi"("section"=w163, "default value"=w169, "key"="LCType" ("section"), "refnum"=w170) -> ("value"=w167:i32, "refnum out"=w166:T29)  [unwired: 1 in, 5 out]
              n92 = global write "_Global LC Driver.vi" "LC Type"(w167) -> ()
              n93 = call-poly <vilib>:"Read Key.vi"("section"=w163, "default value"=w162, "key"="UpsIP" ("section"), "refnum"=w166) -> ("value"=w161:string, "refnum out"=w165:T29)  [unwired: 2 in, 4 out]
              n94 = call "_Remote Connect.vi"("IP Address"=w183) -> ("error out"=w187:errorcluster, "TCP"=w186:bool)  [unwired: 1 in, 4 out]
              n95 = local write "IP Address"(w161) -> ()
              n96 = call <vilib>:"Close Config Data.vi"("write file if changed (T)"=FALSE ("write configuration file? (T)"), "refnum"=w165) -> ()  [unwired: 1 in, 9 out]
              n97 = Not(x=w186) -> (.not. x?=w172:bool)
              n98 = call "_Load Config File.vi"("error in (no error)"=w187) -> ("error out"=w189:errorcluster, "Instrument"=w160:string[])  [unwired: 5 out]
              n99 = Index Array(array=w160, index #1=1 ("index")) -> (element #1=w153:string, element #2=w152:string)  [unwired: 1 in]
              n100 = Match Pattern(string=w152, regular expression=w156) -> (offset past match=w157:i32)  [unwired: 4 out]
              n101 = Match Pattern(string=w153, regular expression=w156) -> (offset past match=w158:i32)  [unwired: 4 out]
              n102 = Greater Or Equal To 0?(x=w157) -> (x >= 0?=w154:bool)
              n103 = Greater Or Equal To 0?(x=w158) -> (x >= 0?=w155:bool)
              n104 = Or(x=w155, y=w154) -> (x .or. y?=w151:bool)
              n105 = global write "_Global Configuration.vi" "UseLeybold"(w151) -> ()
              n106 = global write "_Global Configuration.vi" "Sim"(w172) -> ()
              n107 = call "_Handle Error.vi"("error in (no error)"=w189) -> ()  [unwired: 2 in, 5 out]
              n108 = case shown="True" w172 {
                frame False {
                  n109 = Wait (ms)(milliseconds to wait=u32 2800) -> ()  [unwired: 1 out]
                }
                frame True {
                }
              }
              n110 = Select(t="connected", s=w186, f="running in simulation") -> (s? t:f=w178:string)
              n111 = call "_Remote Communicate.vi"("error in (no error)"=w189, "Command"=_RT_Command."Get Info") -> ("error out"=w188:errorcluster, "Info"=w185:string)  [unwired: 4 in, 2 out]
              n112 = Format Into String(format string="Remote system, %s, is %s: %s", w183, w178, w185) -> (resulting string=w179:string)  [unwired: 2 in, 1 out]
              n113 = call "_Log Events.vi"("error in (no error)"=w188, "Event"=w179, "Log Command"=_Log_Command."Write" ("File Command")) -> ()  [unwired: 5 in, 2 out]
              n114 = property on="Tab Control" class="TabCtl (strict)"() -> ("Pages"=w149:refnum<vi>[])  [unwired: 2 in, 2 out]
              n115 = Index Array(array=w149, index #1=1 ("index"), index #2=0 ("index")) -> (element #1=w148:refnum<vi>, element #2=w147:refnum<vi>)
              n116 = property class="Page"(reference=w148, "PageVis"=w144) -> ()  [unwired: 1 in, 2 out]
              n117 = property class="Page"(reference=w147, "PageVis"=w144) -> ()  [unwired: 1 in, 2 out]
            }
            frame #2 {
              w210 = T19[] []  # ADC Table
              w213 = FALSE ("Update (T)")
              w201 = u8 0 ("Disabled")
              w207 = FALSE ("Unit")
              n118 = local read "Pos/Neg"() -> (w193:enum32{"Positive", "Negative"})
              n119 = call "_Remote Communicate.vi"("Command"=_RT_Command."Get ADC Table") -> ("Info"=w211:string)  [unwired: 5 in, 3 out]
              n120 = Equal?(x=w193, y=enum32{"Positive", "Negative"}."Positive" ("Pos/Neg")) -> (x = y?=w191:bool)
              n121 = Unflatten From String(type=w210, binary string=w211) -> (value=w209:T19[])  [unwired: 1 in, 4 out]
              n122 = call "_Update Oscillators.vi"("UpdateInput (F)"=TRUE, "ADC Table"=w209, "Pole Swap (T)"=w213, "Update (T)"=w213, "Mode(pos)"=w191, "Oscillator Settings"=w214) -> ("Q1RF Frequency"=→"New Frequence" →"Old Frequency":dbl, "Pole"=w194:bool[])  [unwired: 2 in, 2 out]
              n123 = call "Get Pole Orientations.vi"("Pole"=w194) -> ("Pole Swap Options Negative"=w195:T7, "Pole Swap Options Positive"=w196:T7)  [unwired: 9 in]
              n124 = local write "Pole Swap Options Positive"(w196) -> ()
              n125 = local write "Pole Swap Options Negative"(w195) -> ()
              n126 = property on="Detector" class="Tbl (strict)"("Disabled"=w201) -> ()  [unwired: 2 in, 2 out]
              n127 = property on="Gas Flows" class="Tbl (strict)"("Disabled"=w201) -> ()  [unwired: 2 in, 2 out]
              n128 = property on="Heaters" class="Tbl (strict)"("Disabled"=w201) -> ()  [unwired: 2 in, 2 out]
              n129 = property on="Source Probes" class="Tbl (strict)"("Disabled"=w201) -> ()  [unwired: 2 in, 2 out]
              n130 = property on="Corona/Curtain High Voltage" class="Tbl (strict)"("Disabled"=w201) -> ()  [unwired: 2 in, 2 out]
              n131 = property on="Lens 1" class="Tbl (strict)"("Disabled"=w201) -> ()  [unwired: 2 in, 2 out]
              n132 = property on="Lens 2" class="Tbl (strict)"("Disabled"=w201) -> ()  [unwired: 2 in, 2 out]
              n133 = property on="Run" class="Bool"("Visible"=TRUE) -> ()  [unwired: 2 in, 2 out]
              n134 = property on="Cancel" class="Bool (strict)"("Visible"=w207) -> ()  [unwired: 2 in, 2 out]
              n135 = property on="Turbo OK" class="Bool (strict)"("Visible"=w207) -> ()  [unwired: 2 in, 2 out]
              n136 = property on="SVG OK" class="Bool (strict)"("Visible"=w207) -> ()  [unwired: 2 in, 2 out]
              n137 = property on="Quad/Tune OK" class="Bool (strict)"("Visible"=w207) -> ()  [unwired: 2 in, 2 out]
              n138 = property on="Intlk/Per OK" class="Bool (strict)"("Visible"=w207) -> ()  [unwired: 2 in, 2 out]
              n139 = property on="Firmware OK" class="Bool (strict)"("Visible"=w207) -> ()  [unwired: 2 in, 2 out]
              n140 = property on="Progress Bar" class="Slide (strict)"("Visible"=w207) -> ()  [unwired: 2 in, 2 out]
              n141 = property on="Voltage OK" class="Bool (strict)"("Visible"=w207) -> ()  [unwired: 2 in, 2 out]
              n142 = call <vilib>:"Application Directory.vi"() -> ("Application Directory"=w197:path)
              n143 = Build Path(base path=w197, name or relative path="DEFAULT_SETTINGS.d2m") -> (appended path=w205:path)
              n144 = property on="Load Tune File" class="Bool (strict)"("Val(Sgnl)"=FALSE ("Value (Signaling)")) -> ()  [unwired: 2 in, 2 out]
              n145 = property on="Refresh" class="Bool (strict)"("Val(Sgnl)"=TRUE ("Use temporary file (F)")) -> ()  [unwired: 2 in, 2 out]
              n146 = call "_Save All Tables.vi"("SaveOption (Temporary File)"=T16."Temporary File" ("Use temporary file (F)")) -> ()  [unwired: 2 in, 5 out]
              n147 = property on="Tab Control" class="TabCtl (strict)"("Val(Sgnl)"=T2."System Config" ("Value (Signaling)")) -> ()  [unwired: 2 in, 2 out]
              n148 = local write "Tune File"(w205) -> ()
              n149 = local write "Running"(w207) -> ()
              n150 = local write "Quit"(w207) -> ()
              n151 = local write "LBFreqTemp"(FALSE ("LBFreqTemp")) -> ()
              n152 = local write "Cancel"(w207) -> ()
              "ADC List" <- 130 ("ADC List")
            }
            frame #3 {
              w220 = cluster{u32, u32}[] [{16711680, 16711680}, {10421504, 10421504}, {8323072, 8323072}, {5177856, 5177856}]  # RedColor
              w221 = cluster{u32, u32}[] [{12369084, 12369084}, {9868950, 9868950}, {12369084, 12369084}, {9868950, 9868950}]  # GrayColor
              w230 = T31 {"Door"=TRUE, "Curtain"=TRUE, "Pressure"=TRUE, "Turbo"=TRUE, "SysPoll"=TRUE, "GasFlag"=TRUE, "SourceExhaust"=TRUE}  # StartupOptions
              # "Initialize the options based on current settings"
              n153 = call "_Remote Communicate.vi"("Command"=_RT_Command."Get Startup") -> ("error out"=w217:errorcluster, "Info"=w233:string)  [unwired: 5 in, 2 out]
              n154 = call <vilib>:"Trim Whitespace.vi"("string"=w233) -> ("trimmed string"=w232:string)  [unwired: 1 in]
              n155 = Empty String/Path?(string/path=w232) -> (empty?=w231:bool)
              n156 = Unflatten From String(type=w230, binary string=w233) -> (value=w229:T31)  [unwired: 1 in, 4 out]
              n157 = stacked-sequence {
                tunnel: w217 -> [_]
                frame #0 {
                  n158 = call "_Remote Get Brief Status.vi"() -> ()  [unwired: 2 in, 3 out]
                }
              }
              n159 = call "_Remote Set PIC.vi"("PIC Channel"=_PIC_Channel."Corona +HV") -> ("error out"=w240:errorcluster, "Received Header"=→"Corona":u16)  [unwired: 2 in, 3 out]
              n160 = Select(t=w230, s=w231, f=w229) -> (s? t:f=w228:T31)
              n161 = Unbundle By Name(w228) -> ("Door"=w227:bool, "Curtain"=w226:bool, "Pressure"=w225:bool, "Turbo"=w224:bool, "SysPoll"=w223:bool, "GasFlag"=w222:bool)
              n162 = call "_Remote Set PIC.vi"("error in (no error)"=w240, "PIC Channel"=_PIC_Channel."Source 1 Temp") -> ("error out"=w239:errorcluster, "Received Header"=→"Source 1":u16)  [unwired: 1 in, 3 out]
              n163 = call "_Remote Set PIC.vi"("error in (no error)"=w239, "PIC Channel"=_PIC_Channel."Source 2 Temp") -> ("error out"=w238:errorcluster, "Received Header"=→"Source 2":u16)  [unwired: 1 in, 3 out]
              n164 = Compound Arithmetic op=AND(w227, w226, w225, w224, w223, w222) -> (w218:bool)
              n165 = call "_Remote Set PIC.vi"("error in (no error)"=w238, "PIC Channel"=_PIC_Channel."HSID Temp") -> ("Received Header"=→"HSID":u16)  [unwired: 1 in, 4 out]
              n166 = Select(t=w221, s=w218, f=w220) -> (s? t:f=w219:cluster{u32, u32}[])
              n167 = property on="Options" class="Bool"("Colors [4]"=w219) -> ()  [unwired: 2 in, 2 out]
            }
            frame #4 {
              w254 = FALSE  # FrequencyTune
              w256 = FALSE  # CalAjusted
              w246 = _RT_Instrument_State."Ready" ("y")
              w263 = FALSE  # Running
              w264 = TRUE  # Update
              n168 = call <vilib>:"Unset Busy.vi"("error in (no error)"=w248) -> ("error out"=w247:errorcluster)  [unwired: 1 in, 9 out]
              n169 = Bundle("Configuration 2"=T18 {"Table"=[{"Name"="Q1 RF", "Ch#"=1, "Min"=0.0, "Max"=1500.0, "Def+"=400.0, "Def-"=400.0, "Offset"=0.0, "Slope"=218.45, "Type"=64, "Description"="Quadrupole 1 RF", "SettleT"=5.0}, {"Name"="Q1 DC", "Ch#"=4, "Min"=0.0, "Max"=1500.0, "Def+"=600.0, "Def-"=600.0, "Offset"=0.0, "Slope"=218.45, "Type"=64, "Description"="Quadrupole 1 DC", "SettleT"=5.0}, {"Name"="Q1 RR", "Ch#"=7, "Min"=0.0, "Max"=64000.0, "Def+"=32000.0, "Def-"=32000.0, "Offset"=32768.0, "Slope"=-1.0, "Type"=64, "Description"="Quadrupole 1 PW", "SettleT"=5.0}, {"Name"="Q2 RF", "Ch#"=2, "Min"=0.0, "Max"=1500.0, "Def+"=400.0, "Def-"=400.0, "Offset"=0.0, "Slope"=218.45, "Type"=64, "Description"="Quadrupole 2 RF", "SettleT"=5.0}, {"Name"="Q2 DC", "Ch#"=5, "Min"=0.0, "Max"=1500.0, "Def+"=600.0, "Def-"=600.0, "Offset"=0.0, "Slope"=218.45, "Type"=64, "Description"="Quadrupole 2 DC", "SettleT"=5.0}, {"Name"="Q2 RR", "Ch#"=9, "Min"=0.0, "Max"=64000.0, "Def+"=32000.0, "Def-"=32000.0, "Offset"=32768.0, "Slope"=-1.0, "Type"=64, "Description"="Quadrupole 2 PW", "SettleT"=5.0}, {"Name"="M1 RF", "Ch#"=3, "Min"=0.0, "Max"=500.0, "Def+"=400.0, "Def-"=400.0, "Offset"=0.0, "Slope"=14.7, "Type"=6, "Description"="Multipole 1 RF", "SettleT"=5.0}, {"Name"="EV", "Ch#"=20, "Min"=-400.0, "Max"=400.0, "Def+"=0.0, "Def-"=0.0, "Offset"=32768.0, "Slope"=-65.7, "Type"=7, "Description"="Entrance voltage", "SettleT"=5.0}, {"Name"="ED", "Ch#"=21, "Min"=-400.0, "Max"=400.0, "Def+"=0.0, "Def-"=0.0, "Offset"=32768.0, "Slope"=-131.0, "Type"=7, "Description"="Not Used 1", "SettleT"=5.0}, {"Name"="M1", "Ch#"=19, "Min"=-400.0, "Max"=400.0, "Def+"=0.0, "Def-"=0.0, "Offset"=32768.0, "Slope"=-65.6, "Type"=7, "Description"="Multipole 1", "SettleT"=5.0}, {"Name"="L1", "Ch#"=18, "Min"=-400.0, "Max"=400.0, "Def+"=0.0, "Def-"=0.0, "Offset"=32760.0, "Slope"=-65.9, "Type"=7, "Description"="Multipole Len 1", "SettleT"=5.0}, {"Name"="M2", "Ch#"=22, "Min"=-400.0, "Max"=400.0, "Def+"=0.0, "Def-"=0.0, "Offset"=32768.0, "Slope"=-66.0, "Type"=7, "Description"="Multipole 2", "SettleT"=5.0}, {"Name"="L2", "Ch#"=11, "Min"=-400.0, "Max"=400.0, "Def+"=0.0, "Def-"=0.0, "Offset"=32768.0, "Slope"=-65.9, "Type"=7, "Description"="Multipole Len 2", "SettleT"=5.0}, {"Name"="PF", "Ch#"=12, "Min"=-400.0, "Max"=400.0, "Def+"=-16.0, "Def-"=16.0, "Offset"=32768.0, "Slope"=-65.8, "Type"=7, "Description"="Prefilter 1", "SettleT"=5.0}, {"Name"="Q1", "Ch#"=6, "Min"=-150.0, "Max"=150.0, "Def+"=-1.0, "Def-"=1.0, "Offset"=32755.0, "Slope"=-131.3, "Type"=11, "Description"="Quadrupole 1", "SettleT"=5.0}, {"Name"="CC L1", "Ch#"=13, "Min"=-400.0, "Max"=400.0, "Def+"=0.0, "Def-"=0.0, "Offset"=32768.0, "Slope"=-65.8, "Type"=7, "Description"="Collision Cell Lens 1", "SettleT"=5.0}, {"Name"="CC L2", "Ch#"=14, "Min"=-400.0, "Max"=400.0, "Def+"=-100.0, "Def-"=100.0, "Offset"=32768.0, "Slope"=-65.8, "Type"=7, "Description"="Collision Cell Lens 2", "SettleT"=5.0}, {"Name"="CC", "Ch#"=23, "Min"=-400.0, "Max"=400.0, "Def+"=-50.0, "Def-"=50.0, "Offset"=32768.0, "Slope"=-65.8, "Type"=7, "Description"="Collision Energy", "SettleT"=5.0}, {"Name"="CC AF", "Ch#"=10, "Min"=-400.0, "Max"=400.0, "Def+"=50.0, "Def-"=-50.0, "Offset"=32768.0, "Slope"=-65.8, "Type"=7, "Description"="Axial Field", "SettleT"=5.0}, {"Name"="CC L3", "Ch#"=15, "Min"=-400.0, "Max"=400.0, "Def+"=-52.5, "Def-"=52.5, "Offset"=32768.0, "Slope"=-65.7, "Type"=7, "Description"="Collision Cell Lens 3", "SettleT"=5.0}, {"Name"="CC L4", "Ch#"=16, "Min"=-400.0, "Max"=400.0, "Def+"=-72.5, "Def-"=72.5, "Offset"=32768.0, "Slope"=-65.7, "Type"=7, "Description"="Collision Cell Lens 4", "SettleT"=5.0}, {"Name"="Q2", "Ch#"=8, "Min"=-150.0, "Max"=150.0, "Def+"=-54.0, "Def-"=54.0, "Offset"=32756.0, "Slope"=-131.3, "Type"=11, "Description"="Quadrupole 2", "SettleT"=5.0}, {"Name"="ID", "Ch#"=17, "Min"=-400.0, "Max"=400.0, "Def+"=-100.0, "Def-"=100.0, "Offset"=32768.0, "Slope"=-65.8, "Type"=18, "Description"="Detector Deflector", "SettleT"=5.0}, {"Name"="DISC", "Ch#"=32, "Min"=10.0, "Max"=2000.0, "Def+"=20.0, "Def-"=20.0, "Offset"=-10.0, "Slope"=1.23, "Type"=18, "Description"="Discriminator", "SettleT"=5.0}, {"Name"="DV", "Ch#"=34, "Min"=0.0, "Max"=3500.0, "Def+"=1000.0, "Def-"=1000.0, "Offset"=0.0, "Slope"=0.615, "Type"=18, "Description"="Detector Voltage", "SettleT"=5.0}, {"Name"="DET horn", "Ch#"=200, "Min"=0.0, "Max"=5500.0, "Def+"=5500.0, "Def-"=5500.0, "Offset"=0.0, "Slope"=0.615, "Type"=16, "Description"="Detector Horn", "SettleT"=200.0}, {"Name"="LS400A", "Ch#"=36, "Min"=0.0, "Max"=420.0, "Def+"=420.0, "Def-"=420.0, "Offset"=0.0, "Slope"=8.4, "Type"=64, "Description"="Len Power Supply A +400", "SettleT"=5.0}, {"Name"="LS-400A", "Ch#"=37, "Min"=-420.0, "Max"=-55.0, "Def+"=-420.0, "Def-"=-420.0, "Offset"=-433.0, "Slope"=-8.4, "Type"=64, "Description"="Len Power Supply A -400", "SettleT"=5.0}, {"Name"="LS400B", "Ch#"=38, "Min"=0.0, "Max"=420.0, "Def+"=420.0, "Def-"=420.0, "Offset"=0.0, "Slope"=8.4, "Type"=64, "Description"="Len Power Supply B +400", "SettleT"=5.0}, {"Name"="LS-400B", "Ch#"=39, "Min"=-420.0, "Max"=-55.0, "Def+"=-420.0, "Def-"=-420.0, "Offset"=-433.0, "Slope"=-8.4, "Type"=64, "Description"="Len Power Supply B  -400", "SettleT"=5.0}, {"Name"="QPS800", "Ch#"=40, "Min"=0.0, "Max"=600.0, "Def+"=600.0, "Def-"=600.0, "Offset"=0.0, "Slope"=4.25, "Type"=64, "Description"="Quad Power Supply +800", "SettleT"=5.0}, {"Name"="QPS-800", "Ch#"=41, "Min"=-600.0, "Max"=-110.0, "Def+"=-600.0, "Def-"=-600.0, "Offset"=-433.0, "Slope"=-4.2, "Type"=64, "Description"="Quad Power Supply -800", "SettleT"=5.0}, {"Name"="DG", "Ch#"=26, "Min"=30.0, "Max"=300.0, "Def+"=40.0, "Def-"=40.0, "Offset"=0.0, "Slope"=32.765, "Type"=32, "Description"="Drying Gas", "SettleT"=1000.0}, {"Name"="NG1", "Ch#"=27, "Min"=0.0, "Max"=500.0, "Def+"=0.0, "Def-"=0.0, "Offset"=0.0, "Slope"=32.765, "Type"=32, "Description"="Nebulizer Gas 1", "SettleT"=1000.0}, {"Name"="HG1", "Ch#"=29, "Min"=0.0, "Max"=350.0, "Def+"=0.0, "Def-"=0.0, "Offset"=0.0, "Slope"=32.765, "Type"=32, "Description"="Heating Gas 1", "SettleT"=1000.0}, {"Name"="NG2", "Ch#"=28, "Min"=0.0, "Max"=500.0, "Def+"=0.0, "Def-"=0.0, "Offset"=0.0, "Slope"=32.765, "Type"=32, "Description"="Nebulizer Gas 2", "SettleT"=1000.0}, {"Name"="HG2", "Ch#"=30, "Min"=0.0, "Max"=350.0, "Def+"=0.0, "Def-"=0.0, "Offset"=0.0, "Slope"=32.765, "Type"=32, "Description"="Heating Gas 2", "SettleT"=1000.0}, {"Name"="CC P", "Ch#"=43, "Min"=0.0, "Max"=500.0, "Def+"=0.0, "Def-"=0.0, "Offset"=0.0, "Slope"=32.765, "Type"=6, "Description"="Collision Pressure", "SettleT"=3000.0}, {"Name"="SX", "Ch#"=42, "Min"=0.0, "Max"=500.0, "Def+"=0.0, "Def-"=0.0, "Offset"=0.0, "Slope"=32.765, "Type"=32, "Description"="Source Exhaust", "SettleT"=1000.0}, {"Name"="ISV2", "Ch#"=204, "Min"=-6000.0, "Max"=6000.0, "Def+"=0.0, "Def-"=0.0, "Offset"=0.0, "Slope"=0.04, "Type"=34, "Description"="Ion Spray HV2", "SettleT"=200.0}, {"Name"="ISV1", "Ch#"=203, "Min"=-6000.0, "Max"=6000.0, "Def+"=0.0, "Def-"=0.0, "Offset"=0.0, "Slope"=0.04, "Type"=34, "Description"="Ion Spray HV1", "SettleT"=200.0}, {"Name"="CD", "Ch#"=202, "Min"=-255.0, "Max"=255.0, "Def+"=0.0, "Def-"=0.0, "Offset"=0.0, "Slope"=1.0, "Type"=34, "Description"="Corona Discharge", "SettleT"=2000.0}, {"Name"="CAP", "Ch#"=201, "Min"=-1100.0, "Max"=1100.0, "Def+"=0.0, "Def-"=0.0, "Offset"=0.0, "Slope"=0.22, "Type"=32, "Description"="Curtain Cap", "SettleT"=200.0}, {"Name"="HSID T", "Ch#"=81, "Min"=0.0, "Max"=300.0, "Def+"=200.0, "Def-"=200.0, "Offset"=0.0, "Slope"=1.0, "Type"=32, "Description"="HSID Temperature", "SettleT"=3000.0}, {"Name"="P1 T", "Ch#"=86, "Min"=0.0, "Max"=500.0, "Def+"=0.0, "Def-"=0.0, "Offset"=0.0, "Slope"=0.7, "Type"=32, "Description"="Probe 1 Temp", "SettleT"=3000.0}, {"Name"="P2 T", "Ch#"=84, "Min"=0.0, "Max"=500.0, "Def+"=0.0, "Def-"=0.0, "Offset"=0.0, "Slope"=0.7, "Type"=32, "Description"="Probe 2 Temp", "SettleT"=3000.0}], "Instrument"=["C:\\USERS\\PUBLIC\\Ion Sniffer\\GOLD\\Config\\Config-Default-Molana-110209.c3n", "Ion Sniffer 03", "Ionics 3Q Simulation", "0", "0", "0", "0", "172.16.0.2", "T", "0", "2864776525 47523813", "2864776525 47523813", "2864776499 66529043", "0", "0"]}, "FrequencyTune"=w254, "CalAjusted"=w256, "Update"=w264, "Running"=w263, "ADC Table"=w257) -> (w262:T32)  [unwired: 1 out]
              n170 = while {
                shift-right: [w457] -> w255
                shift-left: w262 -> [w459]
                tunnel: w265 -> [w456]
                tunnel: w261 -> [w455]
                tunnel: w260 -> [w454]
                tunnel: w259 -> [w453]
                tunnel: w251 -> [w452]
                tunnel: w247 -> [w451]
                stop <- w460 stop-if-true
                n171 = event shown="[6] \"Refresh\": Value Change" {
                  selector: _ -> [_ _ _ _ _ _ _ _ _ _ _ _ _ _ _ _ _ _ _ _ _ _ _ _ _ _ _ _ _ _ _ _ _ _ _ _ _ _ _ _ _ _ _ _ _ _ _ _ _ _ _ _ _ _ _ _ _ _ _ _ _ _ _ _ _ _]
                  dyn-events: _ -> [_ _ _ _ _ _ _ _ _ _ _ _ _ _ _ _ _ _ _ _ _ _ _ _ _ _ _ _ _ _ _ _ _ _ _ _ _ _ _ _ _ _ _ _ _ _ _ _ _ _ _ _ _ _ _ _ _ _ _ _ _ _ _ _ _ _]
                  timeout: 1800 -> [_ _ _ _ _ _ _ _ _ _ _ _ _ _ _ _ _ _ _ _ _ _ _ _ _ _ _ _ _ _ _ _ _ _ _ _ _ _ _ _ _ _ _ _ _ _ _ _ _ _ _ _ _ _ _ _ _ _ _ _ _ _ _ _ _ _]
                  tunnel: [w464 _ w557 _ _ _ _ _ _ _ _ _ _ _ _ _ _ _ _ _ _ _ _ _ _ _ _ _ _ _ _ _ _ _ _ _ _ _ _ _ _ _ _ _ _ _ _ _ _ _ _ _ _ _ _ _ _ _ _ _ _ _ _ _ _ _] -> w460
                  tunnel: w459 -> [w465 w482 w554 w705 w716 w726 w800 w854 w864 w867 w914 w942 w946 w963 w980 w997 w1015 w1027 w1039 w1050 w1068 w1097 w1113 w1120 w1127 w1134 w1146 w1153 w1155 w1180 w1185 w1191 w1197 w1203 w1211 w1217 w1223 w1229 w1242 w1244 w1285 w1294 w1301 w1303 w1314 w1331 w1336 w1341 w1346 w1351 w1356 w1378 w1391 w1397 w1402 w1407 w1419 w1423 w1424 w1426 w1428 w1438 w1504 w1554 w1556 w1582]
                  tunnel: [w465 w484 w553 w709 w713 w725 w803 w853 w864 w867 w914 w942 w946 w963 w980 w997 w1015 w1027 w1039 w1050 w1068 w1097 w1113 w1120 w1127 w1134 w1146 w1153 w1155 w1180 w1185 w1191 w1197 w1203 w1211 w1217 w1223 w1229 w1242 w1243 w1284 w1294 w1301 w1303 w1314 w1331 w1336 w1341 w1346 w1351 w1356 w1378 w1391 w1397 w1402 w1407 w1419 w1423 w1424 w1426 w1428 w1437 w1503 w1554 w1555 w1582] -> w457
                  tunnel: w456 -> [_ w483 _ w711 _ _ _ _ _ _ _ _ _ _ _ _ _ _ _ _ _ _ _ _ _ _ _ _ _ _ _ _ _ _ _ _ _ _ _ _ _ _ _ _ _ _ _ _ _ _ _ _ _ _ _ _ _ _ _ _ _ _ _ _ _ _]
                  tunnel: w455 -> [_ w479 _ _ _ _ _ _ _ _ _ _ _ _ _ _ _ _ _ _ _ _ _ _ _ _ _ _ _ _ _ _ _ _ _ _ _ _ _ _ _ _ _ _ _ _ _ _ _ _ _ _ _ _ _ _ _ _ _ _ _ _ _ _ _ _]
                  tunnel: w454 -> [_ w478 _ _ _ _ _ _ _ _ _ _ _ _ _ _ _ _ _ _ _ _ _ _ _ _ _ _ _ _ _ _ _ _ _ _ _ _ _ _ _ _ _ _ _ _ _ _ _ _ _ _ _ _ _ _ _ _ _ _ _ _ _ _ _ _]
                  tunnel: w453 -> [_ w477 w552 _ _ _ _ _ _ _ _ _ _ _ _ _ _ _ _ _ _ _ _ _ _ _ _ _ _ w1184 _ _ _ _ _ _ _ _ _ w1246 _ w1290 w1297 _ _ _ _ _ _ _ _ _ _ _ _ _ _ _ _ _ _ _ _ _ _ _]
                  tunnel: w452 -> [_ _ w551 _ _ _ _ _ _ _ _ _ _ _ _ _ _ _ _ _ _ _ _ _ _ _ _ _ _ _ _ _ _ _ _ _ _ _ w1240 _ _ _ _ _ _ _ _ _ _ _ _ _ _ _ _ _ _ _ _ _ _ _ _ _ _ _]
                  tunnel: w451 -> [_ _ _ _ _ _ _ _ _ _ _ _ _ _ _ _ _ _ _ _ _ _ _ _ _ _ _ _ _ _ _ _ _ _ _ _ _ _ w1241 _ _ _ _ _ _ _ _ _ _ _ _ _ _ _ _ _ _ _ _ _ _ _ _ _ _ _]
                  event Panel Close? {
                    w461 = FALSE ("Update")
                    w464 = TRUE ("Discard?")
                    n172 = event-data() -> ()  [unwired: 2 out]
                    n173 = call "_Remote Communicate.vi"("Command"=_RT_Command."Stop") -> ("error out"=w462:errorcluster)  [unwired: 5 in, 3 out]
                    n174 = call "_Remote Park Lens.vi"("error in"=w462, "All Ch (F)"=TRUE) -> ()  [unwired: 6 out]
                    n175 = global write "_Global Configuration.vi" "Quit"(w464) -> ()
                    n176 = global write "_Global Configuration.vi" "Run"(w461) -> ()
                    n177 = local write "Running"(w461) -> ()
                    n178 = event-data("Discard?"=w464) -> ()  [unwired: 1 in, 1 out]
                    "Quit" <- w464
                  }
                  event Timeout {
                    n179 = event-data() -> ()  [unwired: 2 out]
                    n180 = Unbundle By Name(w482) -> ("Update"=w481:bool, "Running"=w480:bool, "ADC Table"=w476:T19[])
                    n181 = case shown="False" w481 {
                      tunnel: w482 -> [w490 w548]
                      tunnel: [w489 w546] -> w484
                      tunnel: w480 -> [w492 _]
                      tunnel: w483 -> [w491 _]
                      tunnel: w476 -> [w488 _]
                      tunnel: w479 -> [w487 _]
                      tunnel: w478 -> [w486 _]
                      tunnel: w477 -> [w485 _]
                      frame False {
                        n182 = case shown="False" w492 {
                          tunnel: w491 -> [_ w534]
                          tunnel: w490 -> [w528 w529]
                          tunnel: [w528 w529] -> w489
                          tunnel: w488 -> [w495 _]
                          tunnel: w487 -> [w526 _]
                          tunnel: w486 -> [w523 _]
                          tunnel: w485 -> [w519 _]
                          frame False {
                            w501 = T6 4 items=["None", "ESI", "APCI", "APPI", "MicroSpray"] ("y")
                            w508 = FALSE ("Pole Swap (T)")
                            n183 = call "_Remote Communicate.vi"("Command"=_RT_Command."Read ADC") -> ("Data Array"=w496:i32[])  [unwired: 5 in, 3 out]
                            n184 = call "_Update Oscillators.vi"("UpdateInput (F)"=w508, "ADC Array"=w496, "ADC Table"=w495, "Pole Swap (T)"=w508, "Update (T)"=w508, "Oscillator Settings"=w519) -> ()  [unwired: 2 in, 4 out]
                            n185 = call "_Check ADCs.vi"("ADC Table"=w495, "ADC Values"=w496, "ADC List Ref"=w523) -> ("Interlocks"=w518:bool[])  [unwired: 4 out]
                            n186 = call "_Remote Calculate ADC.vi"("ADC Table"=w495, "ADC Channel (64)"=u8 56, "ADC Values"=w496) -> ("User Value"=→"M1RF Readback":dbl)  [unwired: 1 in, 3 out]
                            n187 = local read "VoltageInput"() -> (w524:dbl[])
                            n188 = call "_Remote Calculate ADC.vi"("ADC Table"=w495, "ADC Channel (64)"=u8 8, "ADC Values"=w496) -> ("User Value"=→"Main System Current (A)":dbl)  [unwired: 1 in, 3 out]
                            n189 = local read "SG Input"() -> (w517:dbl[])
                            n190 = call "_Check Voltages.vi"("Unit"="Unit", "SGInput"=w517, "ADC Table"=w495, "ADC Values"=w496, "VoltageInput"=w524, "Reference"=w526) -> ("Source 2 Type:"=w503:T6, "Source 1 Type:"=w502:T6, "SVG OK"=→"SVG OK":bool, "Voltage OK"=→"Voltage OK":bool, "Pressure"=→"Vacuum Readings by Region" →"Pressures:":string[][], "DC OK"=→"Quad/Tune OK":bool)
                            "Source 1 Type:" <- w502
                            "Source 2 Type:" <- w503
                            n191 = global read "_Global Configuration.vi" "Single Source"() -> (w516:bool)
                            n192 = Equal?(x=w503, y=w501) -> (x = y?=w504:bool)
                            n193 = Equal?(x=w502, y=w501) -> (x = y?=w500:bool)
                            n194 = Index Array(array=w518) -> (element #1=w510:bool, element #2=w511:bool, element #3=w499:bool, element #4=w505:bool, element #5=w513:bool, element #6=w514:bool, element #7=w515:bool)  [unwired: 7 in]
                            "DoorOK" <- w510
                            "VacRdy" <- w511
                            "DryingGasOK" <- w513
                            "ExhaustOK" <- w514
                            "SourceOK" <- w515
                            n195 = Compound Arithmetic op=OR(w505, w504, w516) -> (w512:bool)
                            "HG2OK" <- w512
                            n196 = Or(x=w500, y=w499) -> (x .or. y?=→"HG1OK":bool)
                            n197 = Compound Arithmetic op=AND(w510, w511, w499, w512, w513, w514, w515) -> (→"Intlk/Per OK":bool)
                          }
                          frame True {
                            n198 = Dequeue Element(queue=w534, timeout in ms (-1)=1) -> (element=w532:cluster{T13, dbl, "error out":errorcluster}, timed out?=w531:bool)  [unwired: 1 in, 2 out]
                            n199 = call "_Current Data Global.vi"("Operation"=_Data_Operation."Get Data") -> ()  [unwired: 3 in, 4 out]
                            n200 = case shown="False" w531 {
                              tunnel: w532 -> [w538 _]
                              frame False {
                                n201 = Unbundle(w538) -> (w537:T13, w535:dbl, "error out"=w536:errorcluster)
                                n202 = case shown="\"End\"" w537 {
                                tunnel: w536 -> [_ w539 w540]
                                tunnel: w535 -> [_ _ _]
                                frame "Init", Default {
                                }
                                frame "End" {
                                n203 = call "_Handle Error.vi"("error in (no error)"=w539) -> ()  [unwired: 2 in, 5 out]
                                }
                                frame "Error" {
                                n204 = call "_Handle Error.vi"("error in (no error)"=w540) -> ()  [unwired: 2 in, 5 out]
                                }
                                }
                              }
                              frame True {
                              }
                            }
                          }
                        }
                      }
                      frame True {
                        w545 = T33 1 items=["8080 Series", "100 Series", "200 Series", "300 Series", "Other Series"] ("Model Family (100)")
                        n205 = call "_Check Model Family.vi"("Model Family (100)"=w545) -> ("Yes"=w544:bool)
                        n206 = Select(t=enum32{"0", "200", "100"}."100" ("IonPathMap"), s=w544, f=enum32{"0", "200", "100"}."200" ("IonPathMap")) -> (s? t:f=w543:enum32{"0", "200", "100"})
                        n207 = stacked-sequence {
                          tunnel: w543 -> [w549 _]
                          frame #0 {
                            "IonPathMap" <- w549
                          }
                          frame #1 {
                            n208 = property on="Ion Path" class="Clust (strict)"("Visible"=TRUE) -> ()  [unwired: 2 in, 2 out]
                          }
                        }
                        n209 = Bundle By Name(cluster=w548, "Update"=FALSE) -> (w546:T32)
                      }
                    }
                    n210 = local read "Serial Number"() -> (w467:string)
                    n211 = Format Into String(format string="Serial Number: %s", w467) -> (resulting string=→"SN":string)  [unwired: 2 in, 1 out]
                    n212 = Get Date/Time In Seconds() -> (seconds since 1Jan1904=w475:timestamp)
                    n213 = Get Date/Time String(seconds (now)=w475, want seconds? (F)=TRUE) -> (date string=w472:string, time string=w471:string)  [unwired: 1 in]
                    n214 = Format Into String(format string="%s %s", w472, w471) -> (resulting string=→"Date/Time":string)  [unwired: 2 in, 1 out]
                  }
                  event Menu Selection (User) {
                    n215 = event-data() -> ("ItemTag"=w558:string)  [unwired: 1 out]
                    n216 = Unbundle By Name(w554) -> ("Running"=w559:bool, "ADC Table"=w556:T19[])
                    n217 = case shown="False" w559 {
                      tunnel: w558 -> [w565 _]
                      tunnel: [w564 _] -> w557
                      tunnel: w556 -> [w563 w699]
                      tunnel: [w562 w699] -> w555
                      tunnel: w552 -> [w561 _]
                      tunnel: w551 -> [w560 _]
                      frame False {
                        n218 = case shown="\"Load All Tables\"" w565 {
                          tunnel: [_ _ _ w589 _ _ _ _ _ _ _ _ _ _ _ _ _ _ _ _ w683 _] -> w564
                          tunnel: w563 -> [w567 w568 w581 w587 w591 w595 w600 w605 w610 w615 w620 w625 w629 w650 w652 w656 w660 w664 w665 w668 w685 w698]
                          tunnel: [w567 w568 w582 w587 w591 w594 w599 w604 w609 w614 w619 w624 w633 w650 w652 w656 w660 w664 w665 w668 w685 w698] -> w562
                          tunnel: w561 -> [_ _ w576 _ _ _ _ _ _ _ _ _ _ _ _ _ _ _ _ _ _ _]
                          tunnel: w560 -> [_ _ _ _ _ _ _ _ _ _ _ _ w628 _ _ _ _ _ _ _ _ _]
                          frame "Save All Tables" {
                            n219 = call "_Save All Tables.vi"("SaveOption (Temporary File)"=_SaveOption."Use Dialog") -> ()  [unwired: 2 in, 5 out]
                          }
                          frame Default {
                          }
                          frame "Load All Tables" {
                            w580 = FALSE ("Update (T)")
                            n220 = local read "Pos/Neg"() -> (w571:enum32{"Positive", "Negative"})
                            n221 = Equal?(x=w571, y=enum32{"Positive", "Negative"}."Positive" ("Pos/Neg")) -> (x = y?=w569:bool)
                            n222 = local write "LoadedTable"(TRUE ("LoadedTable")) -> ()
                            n223 = call "_Load All Tables.vi"() -> ("ADC Table"=w578:T19[], "Loaded ADC"=w583:bool)  [unwired: 1 in, 5 out]
                            n224 = call "_Update Oscillators.vi"("UpdateInput (F)"=TRUE, "ADC Table"=w578, "Pole Swap (T)"=w580, "Update (T)"=w580, "Mode(pos)"=w569, "Oscillator Settings"=w576) -> ("Q1RF Frequency"=w575:dbl, "Pole"=w572:bool[])  [unwired: 2 in, 2 out]
                            n225 = local write "New Frequence"(w575) -> ()
                            n226 = local write "Old Frequency"(w575) -> ()
                            n227 = call "Get Pole Orientations.vi"("Pole"=w572) -> ("Pole Swap Options Negative"=w573:T7, "Pole Swap Options Positive"=w574:T7)  [unwired: 9 in]
                            n228 = local write "Pole Swap Options Positive"(w574) -> ()
                            n229 = local write "Pole Swap Options Negative"(w573) -> ()
                            n230 = property on="Refresh" class="Bool (strict)"("Val(Sgnl)"=TRUE ("Use temporary file (F)")) -> ()  [unwired: 2 in, 2 out]
                            n231 = Select(t=w578, s=w583, f=w581) -> (s? t:f=w582:T19[])
                          }
                          frame "Quit" {
                            w589 = TRUE
                            n232 = call "_Remote Communicate.vi"("Command"=_RT_Command."Stop") -> ("error out"=w585:errorcluster)  [unwired: 5 in, 3 out]
                            n233 = call "_Remote Park Lens.vi"("error in"=w585, "All Ch (F)"=TRUE) -> ()  [unwired: 6 out]
                            n234 = global write "_Global Configuration.vi" "Run"(FALSE ("Run")) -> ()
                            n235 = global write "_Global Configuration.vi" "Quit"(w589) -> ()
                            n236 = local write "Quit"(w589) -> ()
                          }
                          frame "ADC Plot" {
                            n237 = call "_Launch Dynamic VI.vi"("VI Name"=path "ADC Plot.vi" ("name or relative path")) -> ()  [unwired: 4 out]
                          }
                          frame "Quad DC without PS Test Points" {
                            w593 = T34 0 items=["Quad DC Board", "Lens 1 (Slot 8) Module", "Lens 2 (Slot 6) Module", "Detector Board", "Quad DC Board with Test Points", "Lens 1 Module with Test Points", "Len 2 Module with Test Points", "", "", "", "", ""] ("Board")
                            n238 = call "Board Calibrator.vi"("Board"=w593) -> ("ADC Table"=w596:T19[], "Suceeded"=w597:bool)  [unwired: 5 out]
                            n239 = Select(t=w596, s=w597, f=w595) -> (s? t:f=w594:T19[])
                          }
                          frame "Quad DC with PS Test Points" {
                            w598 = T34 4 items=["Quad DC Board", "Lens 1 (Slot 8) Module", "Lens 2 (Slot 6) Module", "Detector Board", "Quad DC Board with Test Points", "Lens 1 Module with Test Points", "Len 2 Module with Test Points", "", "", "", "", ""] ("Board")
                            n240 = call "Board Calibrator.vi"("Board"=w598) -> ("ADC Table"=w601:T19[], "Suceeded"=w602:bool)  [unwired: 5 out]
                            n241 = Select(t=w601, s=w602, f=w600) -> (s? t:f=w599:T19[])
                          }
                          frame "Lens 1 without PS Test Points" {
                            w603 = T34 1 items=["Quad DC Board", "Lens 1 (Slot 8) Module", "Lens 2 (Slot 6) Module", "Detector Board", "Quad DC Board with Test Points", "Lens 1 Module with Test Points", "Len 2 Module with Test Points", "", "", "", "", ""] ("Board")
                            n242 = call "Board Calibrator.vi"("Board"=w603) -> ("ADC Table"=w606:T19[], "Suceeded"=w607:bool)  [unwired: 5 out]
                            n243 = Select(t=w606, s=w607, f=w605) -> (s? t:f=w604:T19[])
                          }
                          frame "Lens 1 with PS Test Points" {
                            w608 = T34 5 items=["Quad DC Board", "Lens 1 (Slot 8) Module", "Lens 2 (Slot 6) Module", "Detector Board", "Quad DC Board with Test Points", "Lens 1 Module with Test Points", "Len 2 Module with Test Points", "", "", "", "", ""] ("Board")
                            n244 = call "Board Calibrator.vi"("Board"=w608) -> ("ADC Table"=w611:T19[], "Suceeded"=w612:bool)  [unwired: 5 out]
                            n245 = Select(t=w611, s=w612, f=w610) -> (s? t:f=w609:T19[])
                          }
                          frame "Lens 2 without PS Test Points" {
                            w613 = T34 2 items=["Quad DC Board", "Lens 1 (Slot 8) Module", "Lens 2 (Slot 6) Module", "Detector Board", "Quad DC Board with Test Points", "Lens 1 Module with Test Points", "Len 2 Module with Test Points", "", "", "", "", ""] ("Board")
                            n246 = call "Board Calibrator.vi"("Board"=w613) -> ("ADC Table"=w616:T19[], "Suceeded"=w617:bool)  [unwired: 5 out]
                            n247 = Select(t=w616, s=w617, f=w615) -> (s? t:f=w614:T19[])
                          }
                          frame "Lens 2 with PS Test Points" {
                            w618 = T34 6 items=["Quad DC Board", "Lens 1 (Slot 8) Module", "Lens 2 (Slot 6) Module", "Detector Board", "Quad DC Board with Test Points", "Lens 1 Module with Test Points", "Len 2 Module with Test Points", "", "", "", "", ""] ("Board")
                            n248 = call "Board Calibrator.vi"("Board"=w618) -> ("ADC Table"=w621:T19[], "Suceeded"=w622:bool)  [unwired: 5 out]
                            n249 = Select(t=w621, s=w622, f=w620) -> (s? t:f=w619:T19[])
                          }
                          frame "Detector Board" {
                            w623 = T34 3 items=["Quad DC Board", "Lens 1 (Slot 8) Module", "Lens 2 (Slot 6) Module", "Detector Board", "Quad DC Board with Test Points", "Lens 1 Module with Test Points", "Len 2 Module with Test Points", "", "", "", "", ""] ("Board")
                            n250 = call "Board Calibrator.vi"("Board"=w623) -> ("ADC Table"=w626:T19[], "Suceeded"=w627:bool)  [unwired: 5 out]
                            n251 = Select(t=w626, s=w627, f=w625) -> (s? t:f=w624:T19[])
                          }
                          frame "Ion Spray Voltages" {
                            n252 = call "ISV Calibration.vi"("queue out"=w628) -> ("Channel Values"=w631:dbl[], "Suceeded"=w630:bool, "ADC Table"=w632:T19[])  [unwired: 4 in]
                            n253 = case shown="True" w630 {
                              tunnel: w629 -> [w634 _]
                              tunnel: [w634 w649] -> w633
                              tunnel: w632 -> [_ w649]
                              tunnel: w631 -> [_ w645]
                              frame False {
                              }
                              frame True {
                                w648 = 1 ("index (row)")
                                n254 = Index Array(array=w645) -> (element #1=w644:dbl, element #2=w638:dbl)  [unwired: 2 in]
                                n255 = local read "Corona/Curtain High Voltage"() -> (w643:string[][])
                                n256 = Format Into String(format string="%0.1f", w644) -> (resulting string=w646:string)  [unwired: 2 in, 1 out]
                                n257 = Format Into String(format string="%0.1f", w638) -> (resulting string=w637:string)  [unwired: 2 in, 1 out]
                                n258 = local read "Source Probes"() -> (w640:string[][])
                                n259 = Replace Array Subset(array=w643, new element=w646, index (row)=w648, index (col)=w648) -> (w642:string[][])
                                n260 = Replace Array Subset(array=w640, new element=w637, index (row)=0, index (col)=2 ("disabled index (col)")) -> (w636:string[][])
                                n261 = property on="Corona/Curtain High Voltage" class="Tbl (strict)"("Val(Sgnl)"=w642) -> ()  [unwired: 2 in, 2 out]
                                n262 = property on="Source Probes" class="Tbl (strict)"("Val(Sgnl)"=w636) -> ()  [unwired: 2 in, 2 out]
                              }
                            }
                          }
                          frame "Show Brief Status" {
                            n263 = call "_Launch Dynamic VI.vi"("VI Name"=path "Show Brief Status.vi" ("name or relative path")) -> ()  [unwired: 4 out]
                          }
                          frame "Start System" {
                            n264 = call "_Remote Communicate.vi"("DC Param"=u16 0, "Command"=_RT_Command."Toggle Power") -> ("error out"=w653:errorcluster)  [unwired: 4 in, 3 out]
                            n265 = call <vilib>:"Simple Error Handler.vi"("error in (no error)"=w653) -> ()  [unwired: 1 in, 8 out]
                          }
                          frame "Goto Roughing Pump On Standby" {
                            n266 = call "_Remote Communicate.vi"("DC Param"=u16 1, "Command"=_RT_Command."Toggle Power") -> ("error out"=w657:errorcluster)  [unwired: 4 in, 3 out]
                            n267 = call <vilib>:"Simple Error Handler.vi"("error in (no error)"=w657) -> ()  [unwired: 1 in, 8 out]
                          }
                          frame "Shut Down System" {
                            n268 = call "_Remote Communicate.vi"("DC Param"=u16 2, "Command"=_RT_Command."Toggle Power") -> ("error out"=w661:errorcluster)  [unwired: 4 in, 3 out]
                            n269 = call <vilib>:"Simple Error Handler.vi"("error in (no error)"=w661) -> ()  [unwired: 1 in, 8 out]
                          }
                          frame "Update Methods" {
                            n270 = call "Update Methods.vi"() -> ()  [unwired: 12 in]
                          }
                          frame "Diagnostics Run" {
                            n271 = call "Auto Diagnotics Run.vi"() -> ()  [unwired: 8 in]
                          }
                          frame "Firmware Reboot" {
                            n272 = local read "MS State"() -> (w667:T1)
                            n273 = case shown="Default" w667 {
                              tunnel: [w678 TRUE ("T button?")] -> w666
                              frame Default {
                                n274 = Two Button Dialog(message="MS will have to be shutdown before performing a firmware reboot.", 2:"Continue" ("T button name (\"OK\")")) -> (T button?=w678:bool)  [unwired: 1 out]
                              }
                              frame "Mass Spectrometer is Off" {
                              }
                            }
                            n275 = case shown="True" w666 {
                              frame False {
                              }
                              frame True {
                                n276 = call "_Open Preference File.vi"() -> ("error"=w670:errorcluster, "refnum"=w671:T29)  [unwired: 3 in, 3 out]
                                n277 = call-poly <vilib>:"Read Key.vi"("section"="Lens", "error in (no error)"=w670, "default value"="172.16.0.2", "key"="IPAddress", "refnum"=w671) -> ("error out"=w672:errorcluster, "value"=w669:string, "refnum out"=w673:T29)  [unwired: 1 in, 3 out]
                                n278 = call "_Remote Reboot.vi"("IP Address"=w669) -> ()  [unwired: 1 in, 1 out]
                                n279 = call <vilib>:"Close Config Data.vi"("error in (no error)"=w672, "write file if changed (T)"=FALSE ("write configuration file? (F)"), "refnum"=w673) -> ()  [unwired: 9 out]
                              }
                            }
                          }
                          frame "Switch User" {
                            n280 = disable-structure shown="Disabled" {
                              disable-tunnel: [w687 w689] -> w684
                              disable-tunnel: [w686 w689] -> w682
                              frame Disabled {
                                n281 = call "Get Password.vi"("IonSniffer777"="ionics32") -> ("Advanced"=w686:bool, "Valid"=w687:bool)  [unwired: 5 out]
                              }
                              frame Enabled {
                                w689 = TRUE ("Advanced")
                              }
                            }
                            n282 = global write "_Global Configuration.vi" "Advanced"(w682) -> ()
                            n283 = property on="Options" class="Bool"("Visible"=w682) -> ()  [unwired: 2 in, 2 out]
                            n284 = property on="Edit ADC" class="Bool"("Visible"=w682) -> ()  [unwired: 2 in, 2 out]
                            n285 = property on="Edit Config" class="Bool"("Visible"=w682) -> ()  [unwired: 2 in, 2 out]
                            n286 = property on="FrequencyTuneSetup" class="Bool (strict)"("Visible"=w682) -> ()  [unwired: 2 in, 2 out]
                            n287 = case shown="True" w682 {
                              frame False {
                                n288 = Current VI's Menubar() -> (w691:refnum<k9>)
                                n289 = Delete Menu Items(7:"Direct DAC Control", 9:w691) -> ()  [unwired: 2 in, 2 out]
                              }
                              frame True {
                                w695 = "Direct DAC Control"
                                n290 = Current VI's Menubar() -> (w694:refnum<k9>)
                                n291 = Get Menu Item Info(7:w695, 11:w694) -> (1:w692:bool, 3:w693:refnum<k9>)  [unwired: 1 in, 5 out]
                                n292 = case shown="False" w692 {
                                tunnel: w695 -> [w697 _]
                                tunnel: w693 -> [w696 _]
                                frame False {
                                n293 = Insert Menu Items(8:w697, 9:w696) -> ()  [unwired: 4 in, 3 out]
                                }
                                frame True {
                                }
                                }
                              }
                            }
                            n294 = Not(x=w684) -> (.not. x?=w683:bool)
                            n295 = global write "_Global Configuration.vi" "Quit"(w683) -> ()
                          }
                          frame "Direct DAC Control" {
                            n296 = call "Direct DAC Control.vi"() -> ()  [unwired: 8 in]
                          }
                        }
                      }
                      frame True {
                      }
                    }
                    n297 = Bundle By Name(cluster=w554, "ADC Table"=w555) -> (w553:T32)
                  }
                  event "Run": Value Change {
                    w700 = u8 1 ("Disabled")
                    w706 = T35 2 items=["Diagnostics", "Tune", "Acquisition"] ("RunModule")
                    w701 = FALSE
                    n298 = event-data() -> ()  [unwired: 2 out]
                    n299 = Flush Queue(queue=w711) -> ()  [unwired: 1 in, 3 out]
                    n300 = local write "Running"("Run") -> ()
                    n301 = global write "_Global Configuration.vi" "RunModule"(w706) -> ()
                    n302 = property on="Run" class="Bool"("Visible"=FALSE) -> ()  [unwired: 2 in, 2 out]
                    n303 = property on="Cancel" class="Bool (strict)"("Visible"=TRUE) -> ()  [unwired: 2 in, 2 out]
                    n304 = property on="Detector" class="Tbl (strict)"("Disabled"=w700) -> ()  [unwired: 2 in, 2 out]
                    n305 = property on="Gas Flows" class="Tbl (strict)"("Disabled"=w700) -> ()  [unwired: 2 in, 2 out]
                    n306 = property on="Heaters" class="Tbl (strict)"("Disabled"=w700) -> ()  [unwired: 2 in, 2 out]
                    n307 = property on="Source Probes" class="Tbl (strict)"("Disabled"=w700) -> ()  [unwired: 2 in, 2 out]
                    n308 = property on="Corona/Curtain High Voltage" class="Tbl (strict)"("Disabled"=w700) -> ()  [unwired: 2 in, 2 out]
                    n309 = property on="Lens 1" class="Tbl (strict)"("Disabled"=w700) -> ()  [unwired: 2 in, 2 out]
                    n310 = property on="Lens 2" class="Tbl (strict)"("Disabled"=w700) -> ()  [unwired: 2 in, 2 out]
                    n311 = property on="Turbo OK" class="Bool (strict)"("Visible"=w701) -> ()  [unwired: 2 in, 2 out]
                    n312 = property on="SVG OK" class="Bool (strict)"("Visible"=w701) -> ()  [unwired: 2 in, 2 out]
                    n313 = property on="Intlk/Per OK" class="Bool (strict)"("Visible"=w701) -> ()  [unwired: 2 in, 2 out]
                    n314 = property on="Firmware OK" class="Bool (strict)"("Visible"=w701) -> ()  [unwired: 2 in, 2 out]
                    n315 = property on="Quad/Tune OK" class="Bool (strict)"("Visible"=w701) -> ()  [unwired: 2 in, 2 out]
                    n316 = property on="Voltage OK" class="Bool (strict)"("Visible"=w701) -> ()  [unwired: 2 in, 2 out]
                    n317 = property on="Progress Bar" class="Slide (strict)"("Visible"=TRUE) -> ()  [unwired: 2 in, 2 out]
                    n318 = Bundle By Name(cluster=w705, "Running"=TRUE) -> (w709:T32)
                    "Progress Bar" <- u8 0 ("ProgressBar")
                  }
                  event "Cancel": Value Change {
                    n319 = event-data() -> ()  [unwired: 7 out]
                    n320 = local write "Cancel"(FALSE ("Cancel")) -> ()
                    n321 = stacked-sequence {
                      tunnel: w716 -> [_ w721 _]
                      tunnel: [_ w721 _] -> w714
                      frame #0 {
                        w717 = u8 0 ("Disabled")
                        w718 = TRUE
                        w719 = FALSE ("Update")
                        n322 = property on="Detector" class="Tbl (strict)"("Disabled"=w717) -> ()  [unwired: 2 in, 2 out]
                        n323 = property on="Gas Flows" class="Tbl (strict)"("Disabled"=w717) -> ()  [unwired: 2 in, 2 out]
                        n324 = property on="Heaters" class="Tbl (strict)"("Disabled"=w717) -> ()  [unwired: 2 in, 2 out]
                        n325 = property on="Source Probes" class="Tbl (strict)"("Disabled"=w717) -> ()  [unwired: 2 in, 2 out]
                        n326 = property on="Corona/Curtain High Voltage" class="Tbl (strict)"("Disabled"=w717) -> ()  [unwired: 2 in, 2 out]
                        n327 = property on="Lens 1" class="Tbl (strict)"("Disabled"=w717) -> ()  [unwired: 2 in, 2 out]
                        n328 = property on="Lens 2" class="Tbl (strict)"("Disabled"=w717) -> ()  [unwired: 2 in, 2 out]
                        n329 = call <vilib>:"Set Busy.vi"() -> ()  [unwired: 4 in, 8 out]
                        n330 = global write "_Global Configuration.vi" "Run"(w719) -> ()
                        n331 = property on="Turbo OK" class="Bool (strict)"("Visible"=w718) -> ()  [unwired: 2 in, 2 out]
                        n332 = property on="SVG OK" class="Bool (strict)"("Visible"=w718) -> ()  [unwired: 2 in, 2 out]
                        n333 = property on="Intlk/Per OK" class="Bool (strict)"("Visible"=w718) -> ()  [unwired: 2 in, 2 out]
                        n334 = property on="Firmware OK" class="Bool (strict)"("Visible"=w718) -> ()  [unwired: 2 in, 2 out]
                        n335 = property on="Quad/Tune OK" class="Bool (strict)"("Visible"=w718) -> ()  [unwired: 2 in, 2 out]
                        n336 = property on="Voltage OK" class="Bool (strict)"("Visible"=w718) -> ()  [unwired: 2 in, 2 out]
                        n337 = property on="Progress Bar" class="Slide (strict)"("Visible"=FALSE) -> ()  [unwired: 2 in, 2 out]
                        "Running" <- w719
                      }
                      frame #1 {
                      }
                      frame #2 {
                        n338 = call "_Remote Park Lens.vi"() -> ()  [unwired: 2 in, 6 out]
                        n339 = call <vilib>:"Unset Busy.vi"() -> ()  [unwired: 2 in, 10 out]
                        n340 = property on="Run" class="Bool"("Visible"=TRUE) -> ()  [unwired: 2 in, 2 out]
                        n341 = property on="Cancel" class="Bool (strict)"("Visible"=FALSE) -> ()  [unwired: 2 in, 2 out]
                      }
                    }
                    n342 = Bundle By Name(cluster=w714, "Running"=FALSE) -> (w713:T32)
                  }
                  event "Load Firmware": Value Change {
                    n343 = event-data() -> ()  [unwired: 2 out]
                    n344 = Unbundle By Name(w726) -> ("Running"=w727:bool)
                    n345 = case shown="False" w727 {
                      frame False {
                        n346 = stacked-sequence {
                          seq-local: [_ w774 _] -> [_ _ w783]
                          seq-local: [_ w771 _] -> [_ _ w784]
                          seq-local: [w729 _ _] -> [_ w772 _]
                          seq-local: [w728 _ _] -> [_ _ w782]
                          frame #0 {
                            w742 = ""
                            w732 = "RT Controller Image Info" ("section")
                            # "Update Firmware from Files"
                            n347 = Current VI's Path() -> (path=w770:path)
                            n348 = Strip Path(path=w770) -> (stripped path=w769:path)  [unwired: 1 out]
                            n349 = Strip Path(path=w769) -> (stripped path=w768:path)  [unwired: 1 out]
                            n350 = call "File Dialog"("start path"=w768, "prompt"="Please choose a firmware image folder") -> ("selected path"=w728:path)  [unwired: 5 in, 8 out]
                            n351 = Build Path(base path=w728, name or relative path="RTCtrlr.ini") -> (appended path=w733:path)
                            n352 = call <vilib>:"Open Config Data.vi"("create file if necessary (T)"=FALSE ("create file if necessary? (T)"), "configuration file path"=w733) -> ("error out"=w765:errorcluster, "refnum"=w766:T29)  [unwired: 7 in, 1 out]
                            n353 = call-poly <vilib>:"Read Key.vi"("section"=w732, "error in (no error)"=w765, "default value"=w742, "key"="Model", "refnum"=w766) -> ("error out"=w762:errorcluster, "value"=w740:string, "refnum out"=w763:T29)  [unwired: 1 in, 3 out]
                            n354 = call-poly <vilib>:"Read Key.vi"("section"=w732, "error in (no error)"=w762, "default value"=w742, "key"="Image_Type", "refnum"=w763) -> ("error out"=w759:errorcluster, "value"=w739:string, "refnum out"=w760:T29)  [unwired: 1 in, 3 out]
                            n355 = call-poly <vilib>:"Read Key.vi"("section"=w732, "error in (no error)"=w759, "default value"=w742, "key"="MAC_Address", "refnum"=w760) -> ("error out"=w754:errorcluster, "value"=w736:string, "refnum out"=w755:T29)  [unwired: 1 in, 3 out]
                            n356 = call-poly <vilib>:"Read Key.vi"("section"=w732, "error in (no error)"=w754, "default value"=w742, "key"="Time", "refnum"=w755) -> ("error out"=w745:errorcluster, "value"=w738:string, "refnum out"=w746:T29)  [unwired: 1 in, 3 out]
                            n357 = call-poly <vilib>:"Read Key.vi"("section"=w732, "error in (no error)"=w745, "default value"=w742, "key"="IP_Address", "refnum"=w746) -> ("error out"=w743:errorcluster, "value"=w737:string, "refnum out"=w744:T29)  [unwired: 1 in, 3 out]
                            n358 = call-poly <vilib>:"Read Key.vi"("section"=w732, "error in (no error)"=w743, "default value"=w742, "key"="Host_Name", "refnum"=w744) -> ("error out"=w752:errorcluster, "value"=w735:string, "refnum out"=w753:T29)  [unwired: 1 in, 3 out]
                            n359 = call <vilib>:"Close Config Data.vi"("error in (no error)"=w752, "refnum"=w753) -> ("error out"=w756:errorcluster)  [unwired: 1 in, 8 out]
                            n360 = Format Into String(format string="Model: %s    Image: %s    Created: %s\nIP: %s     MAC: %s     Name: %s", error in=w756, w740, w739, w738, w737, w736, w735) -> (resulting string=w748:string, error out=w749:errorcluster)  [unwired: 1 in]
                            n361 = Unbundle By Name(w749) -> ("status"=w729:bool)
                            n362 = Select(t="Failed to load the backup files.\nPlease find a folder containing the firmware back-up files.", s=w729, f=w748) -> (s? t:f=→"Description":string)
                          }
                          frame #1 {
                            n363 = case shown="False" w772 {
                              selector: w772 -> [_ w781]
                              tunnel: [w778 w780] -> w771
                              frame False {
                                n364 = Two Button Dialog(message="The vacuum pumps will be shut off during firmware update.  Please press OK to continue.") -> (T button?=w778:bool)  [unwired: 2 out]
                              }
                              frame True {
                                n365 = Not(x=w781) -> (.not. x?=w780:bool)
                              }
                            }
                            n366 = global read "_Global Configuration.vi" "Configuration 2"() -> (w777:T18)
                            n367 = Unbundle By Name(w777) -> ("Instrument"=w776:string[])
                            n368 = Index Array(array=w776, index=7) -> (element=w775:string)
                            n369 = call <vilib>:"Trim Whitespace.vi"("string"=w775) -> ("trimmed string"=w774:string)  [unwired: 1 in]
                          }
                          frame #2 {
                            n370 = case shown="True" w784 {
                              tunnel: w783 -> [_ w786]
                              tunnel: w782 -> [_ w785]
                              frame False {
                              }
                              frame True {
                                # "Start firmware update"
                                n371 = stacked-sequence {
                                tunnel: w786 -> [_ w788 _]
                                tunnel: w785 -> [_ w790 _]
                                frame #0 {
                                n372 = call <vilib>:"Set Busy.vi"() -> ()  [unwired: 4 in, 8 out]
                                }
                                frame #1 {
                                w797 = ""
                                n373 = Bundle("trimmed string"=w788, w797, "selected path"=w790, "Source"=enum32{"RT Target", "Folder"}."Folder") -> (w793:T36)  [unwired: 1 out]
                                n374 = Bundle("trimmed string"=w788, w797, "selected path"=w790, "Source"=enum32{"RT Target", "Folder"}."RT Target") -> (w792:T36)  [unwired: 1 out]
                                n375 = call "_Remote RT Copy.vi"("Copy software only"=FALSE, "Image Destination"=w792, "Image Source"=w793) -> ("Error Out"=w789:errorcluster, "Messages"=→"Messages":string)  [unwired: 1 in, 4 out]
                                n376 = case shown="No Error" w789 {
                                selector: w789 -> [_ w799]
                                tunnel: [w798 w799] -> w787
                                frame No Error {
                                n377 = call "_Load Config File.vi"() -> ("error out"=w798:errorcluster)  [unwired: 1 in, 6 out]
                                }
                                frame Error {
                                }
                                }
                                n378 = call "_Handle Error.vi"("error in (no error)"=w787) -> ()  [unwired: 2 in, 5 out]
                                }
                                frame #2 {
                                n379 = call <vilib>:"Unset Busy.vi"() -> ()  [unwired: 2 in, 10 out]
                                }
                                }
                              }
                            }
                          }
                        }
                      }
                      frame True {
                      }
                    }
                    n380 = Bundle By Name(cluster=w726, "Update"=TRUE) -> (w725:T32)
                  }
                  event "Refresh": Value Change {
                    n381 = event-data() -> ()  [unwired: 2 out]
                    n382 = flat-sequence {
                      tunnel: [w805] -> w801
                      tunnel: w800 -> [w805]
                      tunnel: [w812] -> w802
                      tunnel: w801 -> [w812]
                      tunnel: [w852] -> w803
                      tunnel: w802 -> [w852]
                      frame #0 {
                        n383 = call <vilib>:"Set Busy.vi"() -> ()  [unwired: 4 in, 8 out]
                      }
                      frame #1 {
                        w849 = u32 200000000 ("y")
                        # "Firmware Check"
                        n384 = global read "_Global Configuration.vi" "Configuration 2"() -> (w848:T18)
                        n385 = Unbundle By Name(w848) -> ("Instrument"=w847:string[])
                        n386 = Wait (ms)(milliseconds to wait=u32 200) -> ()  [unwired: 1 out]
                        n387 = call "_Remote Communicate.vi"("Command"=_RT_Command."Get Info") -> ("Info"=w850:string)  [unwired: 5 in, 3 out]
                        n388 = Index Array(array=w847, index #1=0 ("index"), index #2=1 ("index"), index #3=2 ("index"), index #4=7 ("index")) -> (element #1=w836:string, element #2=w826:string, element #3=w822:string, element #4=w825:string)
                        n389 = Scan From String(format string="%s %s FPGA: %d; RT: %d; MEM: 1\n%[^,;]; FW:\\s%s ", input string=w850) -> (output 3=w808:i32, output 4=w807:i32, output 6=w806:string)  [unwired: 2 in, 12 out]
                        n390 = Greater?(x=w808, y=w849) -> (0:w832:bool)
                        n391 = Greater?(x=w807, y=w849) -> (0:w840:bool)
                        n392 = local write "Serial Number"(w826) -> ()
                        n393 = Number To Decimal String(number=w807) -> (decimal integer string=w810:string)  [unwired: 1 out]
                        n394 = Number To Decimal String(number=w808) -> (decimal integer string=w811:string)  [unwired: 1 out]
                        n395 = Empty String/Path?(string/path=w836) -> (empty?=w842:bool)
                        n396 = Empty String/Path?(string/path=w826) -> (empty?=w843:bool)
                        n397 = Empty String/Path?(string/path=w822) -> (empty?=w841:bool)
                        n398 = Empty String/Path?(string/path=w825) -> (empty?=w831:bool)
                        n399 = call "_Convert Model Name.vi"("Model"=w822) -> ("Model Name"=w823:T3)  [unwired: 1 in, 1 out]
                        n400 = local read "Current Information:"() -> (w835:string[][])
                        n401 = local write "Model Name"(w823) -> ()
                        n402 = Not(x=w842) -> (.not. x?=w839:bool)
                        n403 = Not(x=w843) -> (.not. x?=w838:bool)
                        n404 = Not(x=w841) -> (.not. x?=w837:bool)
                        n405 = Not(x=w831) -> (.not. x?=w830:bool)
                        n406 = Build Array(w806, w810, w811) -> (w833:string[])
                        n407 = Compound Arithmetic op=AND(w832, w840, w839, w838, w837, w830) -> (→"Firmware OK":bool)
                        n408 = call "_Open Preference File.vi"() -> ("error"=w815:errorcluster, "refnum"=w819:T29)  [unwired: 3 in, 3 out]
                        n409 = Replace Array Subset(array=w835, new element=w833, index (col)=1 ("disabled index (col)")) -> (→"Current Information:":string[][])  [unwired: 1 in]
                        n410 = call-poly <vilib>:"Read Key.vi"("section"="Lens", "error in (no error)"=w815, "default value"="172.16.0.2", "key"="IPAddress" ("section"), "refnum"=w819) -> ("error out"=w814:errorcluster, "value"=w813:string, "refnum out"=w816:T29)  [unwired: 1 in, 3 out]
                        n411 = local write "IP Address"(w813) -> ()
                        n412 = call <vilib>:"Close Config Data.vi"("error in (no error)"=w814, "write file if changed (T)"=FALSE ("write configuration file? (T)"), "refnum"=w816) -> ()  [unwired: 9 out]
                      }
                      frame #2 {
                        n413 = call <vilib>:"Unset Busy.vi"() -> ()  [unwired: 2 in, 10 out]
                      }
                    }
                    n414 = local write "Refresh"(FALSE ("Refresh")) -> ()
                  }
                  event "Header Info": Value Change {
                    n415 = event-data() -> ()  [unwired: 7 out]
                    n416 = local read "Serial Number"() -> (w856:string)
                    n417 = local read "Model Name"() -> (w857:T3)
                    n418 = call "Get Header Info.vi"("Model Name"=w857, "Serial Number"=w856) -> ("Model Name out"=→"Model Name":T3, "IP Address"=→"IP Address":string, "Serial Number out"=→"Serial Number":string)  [unwired: 3 out]
                    n419 = Bundle By Name(cluster=w854, "Update"=TRUE) -> (w853:T32)
                  }
                  event "GotoUPS": Value Change {
                    n420 = event-data() -> ()  [unwired: 2 out]
                    n421 = call-poly <vilib>:"Open URL in Default Browser.vi"("URL"="IP Address") -> ("error out"=w861:errorcluster, "URL out"=w862:string)  [unwired: 5 in]
                    n422 = local write "IP Address"(w862) -> ()
                    n423 = case shown="Error" w861 {
                      frame No Error {
                      }
                      frame Error {
                        n424 = One Button Dialog(message="Invalid address format.  \nTo fully ensure accuracy, please take the following steps:\n1. Open the web page in your default browser.\n2. Copy the command line from the address bar.\n3. Paste the path in Ionica Service Tool, and press \"Go to UPS\".") -> ()  [unwired: 1 in, 1 out]
                      }
                    }
                  }
                  event "SendSyringeCommand": Value Change {
                    n425 = event-data() -> ()  [unwired: 2 out]
                    n426 = Unbundle By Name(w867) -> ("Running"=w866:bool)
                    n427 = case shown="False" w866 {
                      frame False {
                        n428 = case shown="\"status\", Default" "Pump Command" {
                          tunnel: [u8 2 u8 3 u8 12 u8 13 u8 14 u8 17 u8 4 u8 5 u8 18 u8 6 u8 19 u8 11 u8 16 u8 15 u8 7] -> w871
                          frame "start" {
                          }
                          frame "stop" {
                          }
                          frame "pause" {
                          }
                          frame "restart" {
                          }
                          frame "help" {
                          }
                          frame "set units" {
                          }
                          frame "set diameter" {
                          }
                          frame "set rate" {
                          }
                          frame "set time" {
                          }
                          frame "set volume" {
                          }
                          frame "set delay" {
                          }
                          frame "save setting" {
                          }
                          frame "read limit parameter" {
                          }
                          frame "view parameter" {
                          }
                          frame "status", Default {
                          }
                        }
                        n429 = Format Into String(format string="%d,%f", w871, "Input Value") -> (resulting string=w868:string)  [unwired: 2 in, 1 out]
                        n430 = call "_Remote Communicate.vi"("String"=w868, "Command"=_RT_Command."Auxiliary Update") -> ("Info"=→"Return Data":string)  [unwired: 4 in, 3 out]
                      }
                      frame True {
                      }
                    }
                  }
                  event "VoltageInput": Value Change {
                    w900 = "Input"
                    w904 = 8 ("length")
                    n431 = event-data() -> ("NewVal"=w913:dbl[])  [unwired: 1 out]
                    n432 = Number To Fractional String(number=w913, precision (6)=i16 1) -> (F-format string=w905:string[])  [unwired: 2 out]
                    n433 = Array Subset(array=w905, index=0, length=w904) -> (w903:string[])
                    n434 = Array Subset(array=w905, index=w904, length=w904) -> (w902:string[])
                    n435 = Array Subset(array=w905, index=16, length=3) -> (w901:string[])
                    n436 = Build Array (concatenate)(w900, w903) -> (w891:string[])
                    n437 = Build Array (concatenate)(w900, w902) -> (w897:string[])
                    n438 = Build Array (concatenate)("", w901) -> (w899:string[])
                    n439 = Replace Array Subset(array="Lens 1", new element=w891, index (row)=1 ("disabled index (col)")) -> (w893:string[][])  [unwired: 1 in]
                    n440 = Replace Array Subset(array="Lens 2", new element=w897, index (row)=1 ("disabled index (col)")) -> (w898:string[][])  [unwired: 1 in]
                    n441 = Replace Array Subset(array="Detector", new element=w899, index (col)=1 ("disabled index (col)")) -> (w909:string[][])  [unwired: 1 in]
                    n442 = local write "Lens 1"(w893) -> ()
                    n443 = local write "Lens 2"(w898) -> ()
                    n444 = local write "Detector"(w909) -> ()
                  }
                  event "SG Input": Value Change {
                    # "EHSM-1864 - SX row should be removed"
                    # "EHSM-351 - Set SX to 0 - delete the SX entry"
                    n445 = event-data() -> ("NewVal"=w940:dbl[])  [unwired: 1 out]
                    n446 = Number To Fractional String(number=w940, precision (6)=i16 1) -> (F-format string=w929:string[])  [unwired: 2 out]
                    n447 = Split 1D Array(array=w929, index=7) -> (first subarray=w918:string[], second subarray=w927:string[])
                    n448 = Delete From Array(array=w918, length=1, index=5) -> (array with subset deleted=w917:string[])  [unwired: 1 out]
                    n449 = Replace Array Subset(array="Gas Flows", new element=w917, index (col)=2 ("disabled index (col)")) -> (w919:string[][])  [unwired: 1 in]
                    n450 = local write "Gas Flows"(w919) -> ()
                    n451 = Split 1D Array(array=w927, index=3) -> (first subarray=w921:string[], second subarray=w925:string[])
                    n452 = Replace Array Subset(array="Heaters", new element=w921, index (col)=2 ("disabled index (col)")) -> (w935:string[][])  [unwired: 1 in]
                    n453 = local write "Heaters"(w935) -> ()
                    n454 = Split 1D Array(array=w925, index=2) -> (first subarray=w922:string[], second subarray=w923:string[])
                    n455 = Replace Array Subset(array="Source Probes", new element=w922, index (col)=2 ("disabled index (col)")) -> (w920:string[][])  [unwired: 1 in]
                    n456 = local write "Source Probes"(w920) -> ()
                    n457 = Replace Array Subset(array="Corona/Curtain High Voltage", new element=w923, index (col)=1 ("disabled index (col)")) -> (w932:string[][])  [unwired: 1 in]
                    n458 = local write "Corona/Curtain High Voltage"(w932) -> ()
                  }
                  event "Detector": Value Change {
                    n459 = event-data() -> ("OldVal"=w943:string[][], "NewVal"=w944:string[][])  [unwired: 1 out]
                    n460 = Unbundle By Name(w946) -> ("Running"=w945:bool)
                    n461 = case shown="False" w945 {
                      tunnel: w944 -> [w957 _]
                      tunnel: w943 -> [_ w959]
                      frame False {
                        w951 = 1 ("disabled index (col)")
                        n462 = Index Array(array=w957, index (col)=w951) -> (element=w954:string[])  [unwired: 1 in]
                        n463 = Array Subset(array=w954, index=w951, length=3) -> (w953:string[])
                        n464 = local read "VoltageInput"() -> (w950:dbl[])
                        n465 = Fract/Exp String To Number(string=w953) -> (number=w948:dbl[])  [unwired: 4 out]
                        n466 = Replace Array Subset(array=w950, new element=w948, index=16) -> (w947:dbl[])
                        n467 = local read "SG Input"() -> (w955:dbl[])
                        n468 = call "_Remote Set Voltages.vi"("Source/Gas"=w955, "UserValues"=w947) -> ("error out"=w956:errorcluster, "Voltages"=w958:dbl[])  [unwired: 2 in, 2 out]
                        n469 = property on="VoltageInput" class="Arr (strict)"("Val(Sgnl)"=w958) -> ()  [unwired: 2 in, 2 out]
                        n470 = call "_Handle Error.vi"("error in (no error)"=w956) -> ()  [unwired: 2 in, 5 out]
                      }
                      frame True {
                        n471 = local write "Detector"(w959) -> ()
                      }
                    }
                  }
                  event "Lens 1": Value Change {
                    n472 = event-data() -> ("OldVal"=w960:string[][], "NewVal"=w961:string[][])  [unwired: 1 out]
                    n473 = Unbundle By Name(w963) -> ("Running"=w962:bool)
                    n474 = case shown="False" w962 {
                      tunnel: w961 -> [w974 _]
                      tunnel: w960 -> [_ w976]
                      frame False {
                        w964 = 1 ("disabled index (col)")
                        n475 = Index Array(array=w974, index (row)=w964) -> (element=w971:string[])  [unwired: 1 in]
                        n476 = Array Subset(array=w971, index=w964, length=8) -> (w970:string[])
                        n477 = local read "VoltageInput"() -> (w968:dbl[])
                        n478 = Fract/Exp String To Number(string=w970) -> (number=w966:dbl[])  [unwired: 4 out]
                        n479 = Replace Array Subset(array=w968, new element=w966, index=0) -> (w965:dbl[])
                        n480 = local read "SG Input"() -> (w972:dbl[])
                        n481 = call "_Remote Set Voltages.vi"("Source/Gas"=w972, "UserValues"=w965) -> ("error out"=w973:errorcluster, "Voltages"=w975:dbl[])  [unwired: 2 in, 2 out]
                        n482 = property on="VoltageInput" class="Arr (strict)"("Val(Sgnl)"=w975) -> ()  [unwired: 2 in, 2 out]
                        n483 = call "_Handle Error.vi"("error in (no error)"=w973) -> ()  [unwired: 2 in, 5 out]
                      }
                      frame True {
                        n484 = local write "Lens 1"(w976) -> ()
                      }
                    }
                  }
                  event "Lens 2": Value Change {
                    n485 = event-data() -> ("OldVal"=w977:string[][], "NewVal"=w978:string[][])  [unwired: 1 out]
                    n486 = Unbundle By Name(w980) -> ("Running"=w979:bool)
                    n487 = case shown="False" w979 {
                      tunnel: w978 -> [w991 _]
                      tunnel: w977 -> [_ w993]
                      frame False {
                        w981 = 1 ("disabled index (col)")
                        n488 = Index Array(array=w991, index (row)=w981) -> (element=w988:string[])  [unwired: 1 in]
                        n489 = Array Subset(array=w988, index=w981, length=8) -> (w987:string[])
                        n490 = local read "VoltageInput"() -> (w985:dbl[])
                        n491 = Fract/Exp String To Number(string=w987) -> (number=w983:dbl[])  [unwired: 4 out]
                        n492 = Replace Array Subset(array=w985, new element=w983, index=8) -> (w982:dbl[])
                        n493 = local read "SG Input"() -> (w989:dbl[])
                        n494 = call "_Remote Set Voltages.vi"("Source/Gas"=w989, "UserValues"=w982) -> ("error out"=w990:errorcluster, "Voltages"=w992:dbl[])  [unwired: 2 in, 2 out]
                        n495 = property on="VoltageInput" class="Arr (strict)"("Val(Sgnl)"=w992) -> ()  [unwired: 2 in, 2 out]
                        n496 = call "_Handle Error.vi"("error in (no error)"=w990) -> ()  [unwired: 2 in, 5 out]
                      }
                      frame True {
                        n497 = local write "Lens 2"(w993) -> ()
                      }
                    }
                  }
                  event "Gas Flows": Value Change {
                    n498 = event-data() -> ("OldVal"=w994:string[][], "NewVal"=w995:string[][])  [unwired: 1 out]
                    n499 = Unbundle By Name(w997) -> ("Running"=w996:bool)
                    n500 = case shown="False" w996 {
                      tunnel: w995 -> [w1012 _]
                      tunnel: w994 -> [_ w1013]
                      frame False {
                        # "EHSM-351 - Set SX to 0 - add an entry for SX as 0"
                        n501 = Index Array(array=w1012, index (col)=2 ("disabled index (col)")) -> (element=w1010:string[])  [unwired: 1 in]
                        n502 = Fract/Exp String To Number(string=w1010) -> (number=w999:dbl[])  [unwired: 4 out]
                        n503 = Insert Into Array(array=w999, index=5, new element=0.0 ("new element/subarray")) -> (w998:dbl[])
                        n504 = Reshape Array(w998, 7 ("dimension size")) -> (w1001:dbl[])
                        n505 = local read "SG Input"() -> (w1006:dbl[])
                        n506 = local read "VoltageInput"() -> (w1007:dbl[])
                        n507 = Replace Array Subset(array=w1006, new element=w1001, index=0) -> (w1000:dbl[])
                        n508 = call "_Remote Set Voltages.vi"("Source/Gas"=w1000, "UserValues"=w1007) -> ("error out"=w1009:errorcluster, "Source/Gas Out"=w1008:dbl[])  [unwired: 2 in, 2 out]
                        n509 = property on="SG Input" class="Arr (strict)"("Val(Sgnl)"=w1008) -> ()  [unwired: 2 in, 2 out]
                        n510 = call "_Handle Error.vi"("error in (no error)"=w1009) -> ()  [unwired: 2 in, 5 out]
                      }
                      frame True {
                        n511 = local write "Gas Flows"(w1013) -> ()
                      }
                    }
                  }
                  event "Typical Gas Settings": Value Change {
                    n512 = event-data() -> ()  [unwired: 2 out]
                    n513 = Unbundle By Name(w1015) -> ("Running"=w1014:bool)
                    n514 = case shown="False" w1014 {
                      frame False {
                        n515 = global read "_Global Configuration.vi" "Single Source"() -> (w1019:bool)
                        n516 = local read "VoltageInput"() -> (w1023:dbl[])
                        n517 = local read "SG Input"() -> (w1022:dbl[])
                        n518 = Select(t=dbl[] [150.0, 200.0, 350.0, 0.0, 0.0, 0.0, 450.0] ("output array"), s=w1019, f=dbl[] [150.0, 200.0, 350.0, 200.0, 350.0, 0.0, 450.0] ("output array")) -> (s? t:f=w1017:dbl[])
                        n519 = Replace Array Subset(array=w1022, new element=w1017, index=0) -> (w1020:dbl[])
                        n520 = call "_Remote Set Voltages.vi"("Source/Gas"=w1020, "UserValues"=w1023) -> ("error out"=w1025:errorcluster, "Source/Gas Out"=w1024:dbl[])  [unwired: 2 in, 2 out]
                        n521 = property on="SG Input" class="Arr (strict)"("Val(Sgnl)"=w1024) -> ()  [unwired: 2 in, 2 out]
                        n522 = call "_Handle Error.vi"("error in (no error)"=w1025) -> ()  [unwired: 2 in, 5 out]
                      }
                      frame True {
                      }
                    }
                  }
                  event "Max Gas Settings": Value Change {
                    n523 = event-data() -> ()  [unwired: 2 out]
                    n524 = Unbundle By Name(w1027) -> ("Running"=w1026:bool)
                    n525 = case shown="False" w1026 {
                      frame False {
                        n526 = global read "_Global Configuration.vi" "Single Source"() -> (w1031:bool)
                        n527 = Select(t=dbl[] [300.0, 450.0, 350.0, 0.0, 0.0, 0.0, 500.0] ("output array"), s=w1031, f=dbl[] [300.0, 450.0, 350.0, 450.0, 350.0, 0.0, 500.0] ("output array")) -> (s? t:f=w1028:dbl[])
                        n528 = local read "VoltageInput"() -> (w1035:dbl[])
                        n529 = local read "SG Input"() -> (w1034:dbl[])
                        n530 = Replace Array Subset(array=w1034, new element=w1028, index=0) -> (w1032:dbl[])
                        n531 = call "_Remote Set Voltages.vi"("Source/Gas"=w1032, "UserValues"=w1035) -> ("error out"=w1037:errorcluster, "Source/Gas Out"=w1036:dbl[])  [unwired: 2 in, 2 out]
                        n532 = property on="SG Input" class="Arr (strict)"("Val(Sgnl)"=w1036) -> ()  [unwired: 2 in, 2 out]
                        n533 = call "_Handle Error.vi"("error in (no error)"=w1037) -> ()  [unwired: 2 in, 5 out]
                      }
                      frame True {
                      }
                    }
                  }
                  event "Min Gas Settings": Value Change {
                    n534 = event-data() -> ()  [unwired: 2 out]
                    n535 = Unbundle By Name(w1039) -> ("Running"=w1038:bool)
                    n536 = case shown="False" w1038 {
                      frame False {
                        n537 = local read "VoltageInput"() -> (w1044:dbl[])
                        n538 = local read "SG Input"() -> (w1043:dbl[])
                        n539 = Replace Array Subset(array=w1043, new element=dbl[] [30.0, 0.0, 0.0, 0.0, 0.0, 0.0, 0.0] ("output array"), index=0) -> (w1041:dbl[])
                        n540 = call "_Remote Set Voltages.vi"("Source/Gas"=w1041, "UserValues"=w1044) -> ("error out"=w1046:errorcluster, "Source/Gas Out"=w1045:dbl[])  [unwired: 2 in, 2 out]
                        n541 = property on="SG Input" class="Arr (strict)"("Val(Sgnl)"=w1045) -> ()  [unwired: 2 in, 2 out]
                        n542 = call "_Handle Error.vi"("error in (no error)"=w1046) -> ()  [unwired: 2 in, 5 out]
                      }
                      frame True {
                      }
                    }
                  }
                  event "Heaters": Value Change {
                    n543 = event-data() -> ("OldVal"=w1047:string[][], "NewVal"=w1048:string[][])  [unwired: 1 out]
                    n544 = Unbundle By Name(w1050) -> ("Running"=w1049:bool)
                    n545 = case shown="False" w1049 {
                      tunnel: w1048 -> [w1062 _]
                      tunnel: w1047 -> [_ w1064]
                      frame False {
                        n546 = Index Array(array=w1062, index (col)=2 ("disabled index (col)")) -> (element=w1060:string[])  [unwired: 1 in]
                        n547 = Fract/Exp String To Number(string=w1060) -> (number=w1055:dbl[])  [unwired: 4 out]
                        n548 = local read "VoltageInput"() -> (w1057:dbl[])
                        n549 = local read "SG Input"() -> (w1056:dbl[])
                        n550 = Reshape Array(w1055, 3 ("dimension size")) -> (w1053:dbl[])
                        n551 = Replace Array Subset(array=w1056, new element=w1053, index=7) -> (w1051:dbl[])
                        n552 = call "_Remote Set Voltages.vi"("Source/Gas"=w1051, "UserValues"=w1057) -> ("error out"=w1059:errorcluster, "Source/Gas Out"=w1058:dbl[], "Voltages"=w1063:dbl[])  [unwired: 2 in, 1 out]
                        n553 = property on="VoltageInput" class="Arr (strict)"("Val(Sgnl)"=w1063) -> ()  [unwired: 2 in, 2 out]
                        n554 = call "_Handle Error.vi"("error in (no error)"=w1059) -> ()  [unwired: 2 in, 5 out]
                        n555 = property on="SG Input" class="Arr (strict)"("Val(Sgnl)"=w1058) -> ()  [unwired: 2 in, 2 out]
                      }
                      frame True {
                        n556 = local write "Heaters"(w1064) -> ()
                      }
                    }
                  }
                  event "Source Probes": Value Change {
                    n557 = event-data() -> ("OldVal"=w1065:string[][], "NewVal"=w1066:string[][])  [unwired: 1 out]
                    n558 = Unbundle By Name(w1068) -> ("Running"=w1067:bool)
                    n559 = case shown="False" w1067 {
                      tunnel: w1066 -> [w1091 _]
                      tunnel: w1065 -> [_ w1093]
                      frame False {
                        w1073 = 0.0 ("t")
                        w1078 = T6 2 items=["None", "ESI", "APCI"] ("Source 1 Type:")
                        n560 = local read "Source 1 Type:"() -> (w1080:T6)
                        n561 = local read "Source 2 Type:"() -> (w1079:T6)
                        n562 = Index Array(array=w1091, index (col)=2 ("disabled index (col)")) -> (element=w1089:string[])  [unwired: 1 in]
                        n563 = Fract/Exp String To Number(string=w1089) -> (number=w1084:dbl[])  [unwired: 4 out]
                        n564 = Equal?(x=w1080, y=w1078) -> (x = y?=w1077:bool)
                        n565 = Equal?(x=w1078, y=w1079) -> (x = y?=w1075:bool)
                        n566 = local read "VoltageInput"() -> (w1086:dbl[])
                        n567 = local read "SG Input"() -> (w1085:dbl[])
                        n568 = Reshape Array(w1084, 2 ("dimension size")) -> (w1070:dbl[])
                        n569 = Index Array(array=w1070) -> (element #1=w1076:dbl, element #2=w1074:dbl)  [unwired: 2 in]
                        n570 = Select(t=w1073, s=w1075, f=w1074) -> (s? t:f=w1071:dbl)
                        n571 = Select(t=w1073, s=w1077, f=w1076) -> (s? t:f=w1072:dbl)
                        n572 = Build Array(w1072, w1071) -> (w1069:dbl[])
                        n573 = Replace Array Subset(array=w1085, new element=w1069, index=10) -> (w1081:dbl[])
                        n574 = call "_Remote Set Voltages.vi"("Source/Gas"=w1081, "UserValues"=w1086) -> ("error out"=w1088:errorcluster, "Source/Gas Out"=w1087:dbl[], "Voltages"=w1092:dbl[])  [unwired: 2 in, 1 out]
                        n575 = property on="VoltageInput" class="Arr (strict)"("Val(Sgnl)"=w1092) -> ()  [unwired: 2 in, 2 out]
                        n576 = call "_Handle Error.vi"("error in (no error)"=w1088) -> ()  [unwired: 2 in, 5 out]
                        n577 = property on="SG Input" class="Arr (strict)"("Val(Sgnl)"=w1087) -> ()  [unwired: 2 in, 2 out]
                      }
                      frame True {
                        n578 = local write "Source Probes"(w1093) -> ()
                      }
                    }
                  }
                  event "Corona/Curtain High Voltage": Value Change {
                    n579 = event-data() -> ("OldVal"=w1094:string[][], "NewVal"=w1095:string[][])  [unwired: 1 out]
                    n580 = Unbundle By Name(w1097) -> ("Running"=w1096:bool)
                    n581 = case shown="False" w1096 {
                      tunnel: w1095 -> [w1109 _]
                      tunnel: w1094 -> [_ w1111]
                      frame False {
                        n582 = Index Array(array=w1109, index (col)=1 ("disabled index (col)")) -> (element=w1107:string[])  [unwired: 1 in]
                        n583 = Fract/Exp String To Number(string=w1107) -> (number=w1102:dbl[])  [unwired: 4 out]
                        n584 = local read "VoltageInput"() -> (w1104:dbl[])
                        n585 = local read "SG Input"() -> (w1103:dbl[])
                        n586 = Reshape Array(w1102, 2 ("dimension size")) -> (w1100:dbl[])
                        n587 = Replace Array Subset(array=w1103, new element=w1100, index=12) -> (w1098:dbl[])
                        n588 = call "_Remote Set Voltages.vi"("Source/Gas"=w1098, "UserValues"=w1104) -> ("error out"=w1106:errorcluster, "Source/Gas Out"=w1105:dbl[], "Voltages"=w1110:dbl[])  [unwired: 2 in, 1 out]
                        n589 = property on="VoltageInput" class="Arr (strict)"("Val(Sgnl)"=w1110) -> ()  [unwired: 2 in, 2 out]
                        n590 = call "_Handle Error.vi"("error in (no error)"=w1106) -> ()  [unwired: 2 in, 5 out]
                        n591 = property on="SG Input" class="Arr (strict)"("Val(Sgnl)"=w1105) -> ()  [unwired: 2 in, 2 out]
                      }
                      frame True {
                        n592 = local write "Source Probes"(w1111) -> ()
                      }
                    }
                  }
                  event "Test Voltages": Value Change {
                    n593 = event-data() -> ()  [unwired: 2 out]
                    n594 = Unbundle By Name(w1113) -> ("Running"=w1112:bool)
                    n595 = case shown="False" w1112 {
                      frame False {
                        w1118 = T37 0 items=["Default", "Minimum", "Maximum", "Zero", "User"] ("VoltageType")
                        n596 = local read "SG Input"() -> (w1115:dbl[])
                        n597 = call "_Remote Set Voltages.vi"("Source/Gas"=w1115, "VoltageType"=w1118) -> ("error out"=w1117:errorcluster, "Source/Gas Out"=w1114:dbl[], "Voltages"=w1116:dbl[])  [unwired: 2 in, 1 out]
                        n598 = property on="VoltageInput" class="Arr (strict)"("Val(Sgnl)"=w1116) -> ()  [unwired: 2 in, 2 out]
                        n599 = property on="SG Input" class="Arr (strict)"("Val(Sgnl)"=w1114) -> ()  [unwired: 2 in, 2 out]
                        n600 = call "_Handle Error.vi"("error in (no error)"=w1117) -> ()  [unwired: 2 in, 5 out]
                      }
                      frame True {
                      }
                    }
                  }
                  event "Max Voltages": Value Change {
                    n601 = event-data() -> ()  [unwired: 2 out]
                    n602 = Unbundle By Name(w1120) -> ("Running"=w1119:bool)
                    n603 = case shown="False" w1119 {
                      frame False {
                        w1125 = T37 2 items=["Default", "Minimum", "Maximum", "Zero", "User"] ("VoltageType")
                        n604 = local read "SG Input"() -> (w1122:dbl[])
                        n605 = call "_Remote Set Voltages.vi"("Source/Gas"=w1122, "VoltageType"=w1125) -> ("error out"=w1124:errorcluster, "Source/Gas Out"=w1121:dbl[], "Voltages"=w1123:dbl[])  [unwired: 2 in, 1 out]
                        n606 = call "_Handle Error.vi"("error in (no error)"=w1124) -> ()  [unwired: 2 in, 5 out]
                        n607 = property on="SG Input" class="Arr (strict)"("Val(Sgnl)"=w1121) -> ()  [unwired: 2 in, 2 out]
                        n608 = property on="VoltageInput" class="Arr (strict)"("Val(Sgnl)"=w1123) -> ()  [unwired: 2 in, 2 out]
                      }
                      frame True {
                      }
                    }
                  }
                  event "Min Voltages": Value Change {
                    n609 = event-data() -> ()  [unwired: 2 out]
                    n610 = Unbundle By Name(w1127) -> ("Running"=w1126:bool)
                    n611 = case shown="False" w1126 {
                      frame False {
                        w1132 = T37 1 items=["Default", "Minimum", "Maximum", "Zero", "User"] ("VoltageType")
                        n612 = local read "SG Input"() -> (w1129:dbl[])
                        n613 = call "_Remote Set Voltages.vi"("Source/Gas"=w1129, "VoltageType"=w1132) -> ("error out"=w1131:errorcluster, "Source/Gas Out"=w1128:dbl[], "Voltages"=w1130:dbl[])  [unwired: 2 in, 1 out]
                        n614 = call "_Handle Error.vi"("error in (no error)"=w1131) -> ()  [unwired: 2 in, 5 out]
                        n615 = property on="SG Input" class="Arr (strict)"("Val(Sgnl)"=w1128) -> ()  [unwired: 2 in, 2 out]
                        n616 = property on="VoltageInput" class="Arr (strict)"("Val(Sgnl)"=w1130) -> ()  [unwired: 2 in, 2 out]
                      }
                      frame True {
                      }
                    }
                  }
                  event "Set 0 Values": Value Change {
                    n617 = event-data() -> ()  [unwired: 2 out]
                    n618 = Unbundle By Name(w1134) -> ("Running"=w1133:bool)
                    n619 = case shown="False" w1133 {
                      frame False {
                        w1139 = T37 3 items=["Default", "Minimum", "Maximum", "Zero", "User"] ("VoltageType")
                        n620 = local read "SG Input"() -> (w1136:dbl[])
                        n621 = call "_Remote Set Voltages.vi"("Source/Gas"=w1136, "VoltageType"=w1139) -> ("error out"=w1138:errorcluster, "Source/Gas Out"=w1135:dbl[], "Voltages"=w1137:dbl[])  [unwired: 2 in, 1 out]
                        n622 = call "_Handle Error.vi"("error in (no error)"=w1138) -> ()  [unwired: 2 in, 5 out]
                        n623 = property on="SG Input" class="Arr (strict)"("Val(Sgnl)"=w1135) -> ()  [unwired: 2 in, 2 out]
                        n624 = property on="VoltageInput" class="Arr (strict)"("Val(Sgnl)"=w1137) -> ()  [unwired: 2 in, 2 out]
                      }
                      frame True {
                      }
                    }
                  }
                  event "Load Tune File": Value Change {
                    n625 = event-data() -> ("NewVal"=w1144:bool)  [unwired: 1 out]
                    n626 = local write "Load Tune File"(FALSE ("Load Tune File")) -> ()
                    n627 = call "_Remote Set Method Voltages.vi"("use dialog? (F)"=w1144, "start path"="Tune File") -> ("error out"=w1143:errorcluster, "Source/Gas Out"=w1141:dbl[], "Voltages"=w1142:dbl[])  [unwired: 3 out]
                    n628 = case shown="No Error" w1143 {
                      tunnel: w1142 -> [w1148 _]
                      tunnel: w1141 -> [w1147 _]
                      frame No Error {
                        n629 = property on="VoltageInput" class="Arr (strict)"("Val(Sgnl)"=w1148) -> ()  [unwired: 2 in, 2 out]
                        n630 = property on="SG Input" class="Arr (strict)"("Val(Sgnl)"=w1147) -> ()  [unwired: 2 in, 2 out]
                      }
                      frame Error {
                      }
                    }
                  }
                  event "Load Default Method": Value Change {
                    n631 = event-data() -> ()  [unwired: 2 out]
                    n632 = property on="Load Tune File" class="Bool (strict)"("Val(Sgnl)"=FALSE ("Value (Signaling)")) -> ()  [unwired: 2 in, 2 out]
                    n633 = call <vilib>:"Application Directory.vi"() -> ("Application Directory"=w1149:path)
                    n634 = Build Path(base path=w1149, name or relative path="DEFAULT_SETTINGS.d2m") -> (appended path=w1152:path)
                    n635 = local write "Tune File"(w1152) -> ()
                  }
                  event "Switch Polarity": Value Change {
                    n636 = event-data() -> ()  [unwired: 2 out]
                    n637 = Unbundle By Name(w1155) -> ("Running"=w1154:bool)
                    n638 = case shown="False" w1154 {
                      frame False {
                        n639 = Split 1D Array(array="VoltageInput", index=16) -> (first subarray=w1159:dbl[], second subarray=w1158:dbl[])
                        n640 = Negate(x=w1159) -> (-x=w1157:dbl[])
                        n641 = Build Array (concatenate)(w1157, w1158) -> (w1156:dbl[])
                        n642 = call "_Remote Set Voltages.vi"("Source/Gas"="SG Input", "UserValues"=w1156) -> ("error out"=w1165:errorcluster, "Source/Gas Out"=w1162:dbl[], "Voltages"=w1164:dbl[])  [unwired: 2 in, 1 out]
                        n643 = property on="SG Input" class="Arr (strict)"("Val(Sgnl)"=w1162) -> ()  [unwired: 2 in, 2 out]
                        n644 = call "_Handle Error.vi"("error in (no error)"=w1165) -> ()  [unwired: 2 in, 5 out]
                        n645 = property on="VoltageInput" class="Arr (strict)"("Val(Sgnl)"=w1164) -> ()  [unwired: 2 in, 2 out]
                      }
                      frame True {
                      }
                    }
                  }
                  event "Pos/Neg", "Force Update Poles": Value Change {
                    n646 = event-data() -> ()  [unwired: 2 out]
                    n647 = Unbundle By Name(w1180) -> ("ADC Table"=w1179:T19[])
                    n648 = Unbundle By Name("Pole Swap Options Positive") -> ("Q1 B"=w1169:bool, "Q2 B"=w1168:bool)
                    n649 = Unbundle By Name("Pole Swap Options Negative") -> ("Q1 A"=w1167:bool, "Q2 A"=w1166:bool)
                    n650 = local write "Force Update Poles"(FALSE ("Force Update Poles")) -> ()
                    n651 = Equal?(x="Pos/Neg", y=enum32{"Positive", "Negative"}."Positive" ("Pos/Neg")) -> (x = y?=w1172:bool)
                    n652 = Build Array(w1169, w1168, w1167, w1166) -> (w1181:bool[])
                    n653 = call "_Update Oscillators.vi"("Pole In"=w1181, "ADC Table"=w1179, "Pole Swap (T)"=TRUE, "Update (T)"=FALSE, "Mode(pos)"=w1172, "Oscillator Settings"=w1184) -> ("Pole"=w1177:bool[])  [unwired: 2 in, 3 out]
                    n654 = call "Get Pole Orientations.vi"("Pole"=w1177) -> ("Pole Swap Options Negative"=w1175:T7, "Pole Swap Options Positive"=w1176:T7)  [unwired: 9 in]
                    n655 = local write "Pole Swap Options Positive"(w1176) -> ()
                    n656 = local write "Pole Swap Options Negative"(w1175) -> ()
                  }
                  event "Pole Swap Options Positive.Q1 A": Value Change {
                    n657 = event-data() -> ("NewVal"=w1189:bool)  [unwired: 1 out]
                    n658 = local read "Pole Swap Options Positive"() -> (w1186:T7)
                    n659 = Not(x=w1189) -> (.not. x?=w1188:bool)
                    n660 = Bundle By Name(cluster=w1186, "Q1 A"=w1189, "Q1 B"=w1188) -> (w1187:T7)
                    n661 = local write "Pole Swap Options Positive"(w1187) -> ()
                    n662 = property on="Force Update Poles" class="Bool (strict)"("Val(Sgnl)"=TRUE ("Value (Signaling)")) -> ()  [unwired: 2 in, 2 out]
                  }
                  event "Pole Swap Options Positive.Q1 B": Value Change {
                    n663 = event-data() -> ("NewVal"=w1195:bool)  [unwired: 1 out]
                    n664 = local read "Pole Swap Options Positive"() -> (w1192:T7)
                    n665 = Not(x=w1195) -> (.not. x?=w1194:bool)
                    n666 = Bundle By Name(cluster=w1192, "Q1 B"=w1195, "Q1 A"=w1194) -> (w1193:T7)
                    n667 = local write "Pole Swap Options Positive"(w1193) -> ()
                    n668 = property on="Force Update Poles" class="Bool (strict)"("Val(Sgnl)"=TRUE ("Value (Signaling)")) -> ()  [unwired: 2 in, 2 out]
                  }
                  event "Pole Swap Options Positive.Q2 A": Value Change {
                    n669 = event-data() -> ("NewVal"=w1201:bool)  [unwired: 1 out]
                    n670 = local read "Pole Swap Options Positive"() -> (w1198:T7)
                    n671 = Not(x=w1201) -> (.not. x?=w1200:bool)
                    n672 = Bundle By Name(cluster=w1198, "Q2 A"=w1201, "Q2 B"=w1200) -> (w1199:T7)
                    n673 = local write "Pole Swap Options Positive"(w1199) -> ()
                    n674 = property on="Force Update Poles" class="Bool (strict)"("Val(Sgnl)"=TRUE ("Value (Signaling)")) -> ()  [unwired: 2 in, 2 out]
                  }
                  event "Pole Swap Options Positive.Q2 B": Value Change {
                    n675 = event-data() -> ("NewVal"=w1207:bool)  [unwired: 1 out]
                    n676 = local read "Pole Swap Options Positive"() -> (w1204:T7)
                    n677 = Not(x=w1207) -> (.not. x?=w1206:bool)
                    n678 = Bundle By Name(cluster=w1204, "Q2 B"=w1207, "Q2 A"=w1206) -> (w1205:T7)
                    n679 = local write "Pole Swap Options Positive"(w1205) -> ()
                    n680 = property on="Force Update Poles" class="Bool (strict)"("Val(Sgnl)"=TRUE ("Value (Signaling)")) -> ()  [unwired: 2 in, 2 out]
                  }
                  event "Pole Swap Options Negative.Q1 A": Value Change {
                    n681 = event-data() -> ("NewVal"=w1213:bool)  [unwired: 1 out]
                    n682 = local read "Pole Swap Options Negative"() -> (w1209:T7)
                    n683 = Not(x=w1213) -> (.not. x?=w1212:bool)
                    n684 = Bundle By Name(cluster=w1209, "Q1 A"=w1213, "Q1 B"=w1212) -> (w1210:T7)
                    n685 = local write "Pole Swap Options Negative"(w1210) -> ()
                    n686 = property on="Force Update Poles" class="Bool (strict)"("Val(Sgnl)"=TRUE ("Value (Signaling)")) -> ()  [unwired: 2 in, 2 out]
                  }
                  event "Pole Swap Options Negative.Q1 B": Value Change {
                    n687 = event-data() -> ("NewVal"=w1219:bool)  [unwired: 1 out]
                    n688 = local read "Pole Swap Options Negative"() -> (w1215:T7)
                    n689 = Not(x=w1219) -> (.not. x?=w1218:bool)
                    n690 = Bundle By Name(cluster=w1215, "Q1 B"=w1219, "Q1 A"=w1218) -> (w1216:T7)
                    n691 = local write "Pole Swap Options Negative"(w1216) -> ()
                    n692 = property on="Force Update Poles" class="Bool (strict)"("Val(Sgnl)"=TRUE ("Value (Signaling)")) -> ()  [unwired: 2 in, 2 out]
                  }
                  event "Pole Swap Options Negative.Q2 A": Value Change {
                    n693 = event-data() -> ("NewVal"=w1225:bool)  [unwired: 1 out]
                    n694 = local read "Pole Swap Options Negative"() -> (w1221:T7)
                    n695 = Not(x=w1225) -> (.not. x?=w1224:bool)
                    n696 = Bundle By Name(cluster=w1221, "Q2 A"=w1225, "Q2 B"=w1224) -> (w1222:T7)
                    n697 = local write "Pole Swap Options Negative"(w1222) -> ()
                    n698 = property on="Force Update Poles" class="Bool (strict)"("Val(Sgnl)"=TRUE ("Value (Signaling)")) -> ()  [unwired: 2 in, 2 out]
                  }
                  event "Pole Swap Options Negative.Q2 B": Value Change {
                    n699 = event-data() -> ("NewVal"=w1231:bool)  [unwired: 1 out]
                    n700 = local read "Pole Swap Options Negative"() -> (w1227:T7)
                    n701 = Not(x=w1231) -> (.not. x?=w1230:bool)
                    n702 = Bundle By Name(cluster=w1227, "Q2 B"=w1231, "Q2 A"=w1230) -> (w1228:T7)
                    n703 = local write "Pole Swap Options Negative"(w1228) -> ()
                    n704 = property on="Force Update Poles" class="Bool (strict)"("Val(Sgnl)"=TRUE ("Value (Signaling)")) -> ()  [unwired: 2 in, 2 out]
                  }
                  event "Print": Value Change {
                    n705 = event-data() -> ()  [unwired: 2 out]
                    n706 = control-ref of="This VI"() -> (w1234:refnum<vi>)
                    n707 = Bundle By Name(cluster=T21 {"Picture Name"="", "VI Reference"=refnum} ("Cluster"), "Picture Name"="ServiceTool.jpg" ("name or relative path"), "VI Reference"=w1234) -> (w1233:T21)
                    n708 = Bundle By Name(cluster=cluster{"Command":string, "Data":variant} {"Command"="", "Data"=variant} ("element"), "Command"="Print", "Data"=w1233) -> (w1237:cluster{"Command":string, "Data":variant})
                    n709 = Enqueue Element(queue=w1240, element=w1237, error in (no error)=w1241) -> ()  [unwired: 1 in, 3 out]
                  }
                  event "Oscillator Settings": Value Change {
                    n710 = event-data() -> ()  [unwired: 7 out]
                    n711 = Unbundle By Name(w1244) -> ("ADC Table"=w1245:T19[])
                    n712 = stacked-sequence {
                      tunnel: w1246 -> [_ w1263 _]
                      tunnel: w1245 -> [_ w1260 _]
                      tunnel: w1244 -> [_ _ w1264]
                      tunnel: [_ _ w1265] -> w1243
                      frame #0 {
                        w1252 = 7 ("disabled index (col)")
                        # "copy the Q1RF input to Q2RF"
                        n713 = Index Array(array="Oscillator Settings", index (row)=1, index (col)=w1252) -> (element=w1250:string)
                        n714 = Replace Array Subset(array="Oscillator Settings", new element=w1250, index (row)=2, index (col)=w1252) -> (w1247:string[][])
                        n715 = local write "Oscillator Settings"(w1247) -> ()
                      }
                      frame #1 {
                        w1261 = TRUE ("Update (T)")
                        n716 = local read "Pos/Neg"() -> (w1255:enum32{"Positive", "Negative"})
                        n717 = Equal?(x=w1255, y=enum32{"Positive", "Negative"}."Positive" ("Pos/Neg")) -> (x = y?=w1253:bool)
                        n718 = call "_Update Oscillators.vi"("UpdateInput (F)"=w1261, "ADC Table"=w1260, "Pole Swap (T)"=FALSE, "Update (T)"=w1261, "Mode(pos)"=w1253, "Oscillator Settings"=w1263) -> ("Q1RF Frequency"=w1259:dbl, "Pole"=w1256:bool[])  [unwired: 2 in, 2 out]
                        n719 = local write "New Frequence"(w1259) -> ()
                        n720 = call "Get Pole Orientations.vi"("Pole"=w1256) -> ("Pole Swap Options Negative"=w1257:T7, "Pole Swap Options Positive"=w1258:T7)  [unwired: 9 in]
                        n721 = local write "Pole Swap Options Positive"(w1258) -> ()
                        n722 = local write "Pole Swap Options Negative"(w1257) -> ()
                      }
                      frame #2 {
                        n723 = Unbundle By Name(w1264) -> ("FrequencyTune"=w1266:bool)
                        n724 = case shown="True" w1266 {
                          tunnel: [w1267 w1270] -> w1265
                          tunnel: w1264 -> [w1267 w1271]
                          frame False {
                          }
                          frame True {
                            n725 = global read "_Global Configuration.vi" "Configuration 2"() -> (w1269:T18)
                            n726 = Unbundle By Name(w1269) -> ("Instrument"=w1268:string[])
                            n727 = Bundle By Name(cluster=w1271, "Configuration 2.Instrument"=w1268) -> (w1270:T32)
                          }
                        }
                      }
                    }
                  }
                  event "Force Update Oscillators": Value Change {
                    w1283 = FALSE ("Update (T)")
                    n728 = event-data() -> ()  [unwired: 2 out]
                    n729 = local write "Force Update Oscillators"(FALSE ("Force Update Poles")) -> ()
                    n730 = local read "Pos/Neg"() -> (w1275:enum32{"Positive", "Negative"})
                    n731 = call "_Remote Communicate.vi"("Command"=_RT_Command."Get ADC Table") -> ("error out"=w1282:errorcluster, "Info"=w1281:string)  [unwired: 5 in, 2 out]
                    n732 = Equal?(x=w1275, y=enum32{"Positive", "Negative"}."Positive" ("Pos/Neg")) -> (x = y?=w1273:bool)
                    n733 = Unflatten From String(type=T19[] [], binary string=w1281, error in (no error)=w1282) -> (value=w1279:T19[])  [unwired: 2 in, 2 out]
                    n734 = call "_Update Oscillators.vi"("UpdateInput (F)"=TRUE ("Pole Swap (T)"), "ADC Table"=w1279, "Pole Swap (T)"=w1283, "Update (T)"=w1283, "Mode(pos)"=w1273) -> ("Pole"=w1276:bool[])  [unwired: 5 in, 1 out]
                    n735 = Bundle By Name(cluster=w1285, "ADC Table"=w1279) -> (w1284:T32)
                    n736 = call "Get Pole Orientations.vi"("Pole"=w1276) -> ("Pole Swap Options Negative"=w1277:T7, "Pole Swap Options Positive"=w1278:T7)  [unwired: 9 in]
                    n737 = local write "Pole Swap Options Positive"(w1278) -> ()
                    n738 = local write "Pole Swap Options Negative"(w1277) -> ()
                  }
                  event "Q1 DC Inputs": Value Change {
                    n739 = event-data() -> ()  [unwired: 2 out]
                    n740 = call "_Remote Update DC.vi"("DC Inputs"="Q1 DC Inputs", "Table Reference"=w1290, "Ch#"=u8[] [4, 7, 6]) -> ("DC Outputs"=w1292:string[][], "Total"=→"Q1 Total":dbl, "VDC"=→"Q1 (VDC)":dbl)  [unwired: 2 out]
                    n741 = local write "Q1 DC Inputs"(w1292) -> ()
                  }
                  event "Q2 DC Inputs": Value Change {
                    n742 = event-data() -> ()  [unwired: 2 out]
                    n743 = call "_Remote Update DC.vi"("DC Inputs"="Q2 DC Inputs", "Table Reference"=w1297, "Ch#"=u8[] [5, 9, 8]) -> ("DC Outputs"=w1300:string[][], "Total"=→"Q2 Total":dbl, "VDC"=→"Q2 (VDC)":dbl)  [unwired: 2 out]
                    n744 = local write "Q2 DC Inputs"(w1300) -> ()
                  }
                  event "Turbo Update": Value Change {
                    n745 = event-data() -> ()  [unwired: 2 out]
                    n746 = Unbundle By Name(w1303) -> ("Running"=w1302:bool)
                    n747 = case shown="False" w1302 {
                      frame False {
                        n748 = stacked-sequence {
                          frame #0 {
                            n749 = call <vilib>:"Set Busy.vi"() -> ()  [unwired: 4 in, 8 out]
                          }
                          frame #1 {
                            w1304 = string[][] [] ("Error History")
                            n750 = local write "Pump Info:"(w1304) -> ()
                            n751 = local write "Temperatures:"(w1304) -> ()
                            n752 = local write "Error History"(w1304) -> ()
                            n753 = local write "Pumping:"(w1304) -> ()
                            n754 = local write "Power / Current:"(w1304) -> ()
                          }
                          frame #2 {
                            w1306 = TRUE
                            n755 = call "_Remote Get Turbo Status.vi"("Update Info"=w1306, "Update Temp"=w1306, "Update Error"=w1306, "Update Pumping"=w1306, "Update Power"=w1306) -> ("Power / Current:"=→"Power / Current:":string[][], "Turbo OK"=→"Turbo OK":bool, "Pump Info:"=→"Pump Info:":string[][], "Temperatures:"=→"Temperatures:":string[][], "Error History"=→"Error History":string[][], "Pumping:"=→"Pumping:":string[][])
                          }
                          frame #3 {
                            n756 = call <vilib>:"Unset Busy.vi"() -> ()  [unwired: 2 in, 10 out]
                          }
                        }
                      }
                      frame True {
                      }
                    }
                  }
                  event "LBFreqTemp": Value Change {
                    n757 = event-data() -> ()  [unwired: 2 out]
                    n758 = Unbundle By Name(w1314) -> ("Running"=w1313:bool)
                    n759 = case shown="False" w1313 {
                      frame False {
                        n760 = stacked-sequence {
                          frame #0 {
                            n761 = call <vilib>:"Set Busy.vi"() -> ()  [unwired: 4 in, 8 out]
                          }
                          frame #1 {
                            n762 = call "_Remote Get Leybold Status.vi"("UpdateOthers"=TRUE) -> ("OtherInfo"=w1328:T38, "Turbo OK"=w1315:bool)  [unwired: 5 in, 4 out]
                            n763 = local write "Turbo OK"(w1315) -> ()
                            n764 = Unbundle By Name(w1328) -> ("Frequency"=→"Frequency (Hz):":u16, "Decel"=→"Decel":bool, "Accel"=→"Accel":bool, "Normal \nOperation"=→"Normal \nOperation":bool, "Turning"=→"Turning":bool, "BearingTemp"=→"Bearing Temperature:":u32, "MotorTemp"=→"Moter Temperature:":u32, "ControllerTemp"=→"Controller Temperature:":u16, "PumpStatus"=→"PumpStatus":u16, "NumErrors"=→"Total Number of Errors:":u32, "NumOverload"=→"Number of Pressure Overload Errors:":u32, "NumFailure"=→"Number of Power Failures:":u32)
                          }
                          frame #2 {
                            n765 = call <vilib>:"Unset Busy.vi"() -> ()  [unwired: 2 in, 10 out]
                          }
                        }
                      }
                      frame True {
                      }
                    }
                    n766 = local write "LBFreqTemp"(FALSE ("LBFreqTemp")) -> ()
                  }
                  event "Update Info": Value Change {
                    n767 = event-data() -> ()  [unwired: 2 out]
                    n768 = Unbundle By Name(w1331) -> ("Running"=w1330:bool)
                    n769 = case shown="False" w1330 {
                      frame False {
                        n770 = stacked-sequence {
                          frame #0 {
                            n771 = call <vilib>:"Set Busy.vi"() -> ()  [unwired: 4 in, 8 out]
                          }
                          frame #1 {
                            n772 = local write "Pump Info:"(string[][] [] ("Error History")) -> ()
                          }
                          frame #2 {
                            n773 = call "_Remote Get Turbo Status.vi"("Update Info"=TRUE) -> ("Pump Info:"=w1333:string[][])  [unwired: 4 in, 5 out]
                            n774 = local write "Pump Info:"(w1333) -> ()
                          }
                          frame #3 {
                            n775 = call <vilib>:"Unset Busy.vi"() -> ()  [unwired: 2 in, 10 out]
                          }
                        }
                      }
                      frame True {
                      }
                    }
                  }
                  event "LBConfiguration": Value Change {
                    n776 = event-data() -> ()  [unwired: 2 out]
                    n777 = Unbundle By Name(w1336) -> ("Running"=w1335:bool)
                    n778 = case shown="False" w1335 {
                      frame False {
                        n779 = stacked-sequence {
                          frame #0 {
                            n780 = call <vilib>:"Set Busy.vi"() -> ()  [unwired: 4 in, 8 out]
                          }
                          frame #1 {
                            n781 = local write "Configuration:"(string[][] [] ("Error History")) -> ()
                          }
                          frame #2 {
                            n782 = call "_Remote Get Leybold Status.vi"("UpdateConfig"=TRUE) -> ("Configuration:"=→"Configuration:":string[][])  [unwired: 5 in, 5 out]
                          }
                          frame #3 {
                            n783 = call <vilib>:"Unset Busy.vi"() -> ()  [unwired: 2 in, 10 out]
                          }
                        }
                      }
                      frame True {
                      }
                    }
                  }
                  event "LBPower": Value Change {
                    n784 = event-data() -> ()  [unwired: 2 out]
                    n785 = Unbundle By Name(w1341) -> ("Running"=w1340:bool)
                    n786 = case shown="False" w1340 {
                      frame False {
                        n787 = stacked-sequence {
                          frame #0 {
                            n788 = call <vilib>:"Set Busy.vi"() -> ()  [unwired: 4 in, 8 out]
                          }
                          frame #1 {
                            n789 = local write "Power:"(string[][] [] ("Error History")) -> ()
                          }
                          frame #2 {
                            n790 = call "_Remote Get Leybold Status.vi"("UpdatePower"=TRUE) -> ("Power:"=→"Power:":string[][])  [unwired: 5 in, 5 out]
                          }
                          frame #3 {
                            n791 = call <vilib>:"Unset Busy.vi"() -> ()  [unwired: 2 in, 10 out]
                          }
                        }
                      }
                      frame True {
                      }
                    }
                  }
                  event "LBRunTime": Value Change {
                    n792 = event-data() -> ()  [unwired: 2 out]
                    n793 = Unbundle By Name(w1346) -> ("Running"=w1345:bool)
                    n794 = case shown="False" w1345 {
                      frame False {
                        n795 = stacked-sequence {
                          frame #0 {
                            n796 = call <vilib>:"Set Busy.vi"() -> ()  [unwired: 4 in, 8 out]
                          }
                          frame #1 {
                            n797 = local write "Run Time:"(string[][] [] ("Error History")) -> ()
                          }
                          frame #2 {
                            n798 = call "_Remote Get Leybold Status.vi"("UpdateRunTime"=TRUE) -> ("Run Time:"=→"Run Time:":string[][])  [unwired: 5 in, 5 out]
                          }
                          frame #3 {
                            n799 = call <vilib>:"Unset Busy.vi"() -> ()  [unwired: 2 in, 10 out]
                          }
                        }
                      }
                      frame True {
                      }
                    }
                  }
                  event "LBError": Value Change {
                    n800 = event-data() -> ()  [unwired: 2 out]
                    n801 = Unbundle By Name(w1351) -> ("Running"=w1350:bool)
                    n802 = case shown="False" w1350 {
                      frame False {
                        n803 = stacked-sequence {
                          frame #0 {
                            n804 = call <vilib>:"Set Busy.vi"() -> ()  [unwired: 4 in, 8 out]
                          }
                          frame #1 {
                            n805 = local write "Errors:"(string[][] [] ("Error History")) -> ()
                          }
                          frame #2 {
                            n806 = call "_Remote Get Leybold Status.vi"("UpdateError"=TRUE) -> ("Errors:"=→"Errors:":string[][])  [unwired: 5 in, 5 out]
                          }
                          frame #3 {
                            n807 = call <vilib>:"Unset Busy.vi"() -> ()  [unwired: 2 in, 10 out]
                          }
                        }
                      }
                      frame True {
                      }
                    }
                  }
                  event "LBUpdateAll": Value Change {
                    n808 = event-data() -> ()  [unwired: 2 out]
                    n809 = Unbundle By Name(w1356) -> ("Running"=w1355:bool)
                    n810 = case shown="False" w1355 {
                      frame False {
                        n811 = stacked-sequence {
                          frame #0 {
                            n812 = call <vilib>:"Set Busy.vi"() -> ()  [unwired: 4 in, 8 out]
                          }
                          frame #1 {
                            w1357 = string[][] [] ("Error History")
                            n813 = local write "Configuration:"(w1357) -> ()
                            n814 = local write "Power:"(w1357) -> ()
                            n815 = local write "Run Time:"(w1357) -> ()
                            n816 = local write "Errors:"(w1357) -> ()
                          }
                          frame #2 {
                            w1376 = TRUE
                            n817 = call "_Remote Get Leybold Status.vi"("UpdateError"=w1376, "UpdateRunTime"=w1376, "UpdatePower"=w1376, "UpdateOthers"=w1376, "UpdateConfig"=w1376) -> ("Run Time:"=w1372:string[][], "Power:"=w1373:string[][], "OtherInfo"=w1370:T38, "Configuration:"=w1374:string[][], "Turbo OK"=w1371:bool, "Errors:"=w1375:string[][])  [unwired: 1 in]
                            n818 = local write "Errors:"(w1375) -> ()
                            n819 = local write "Power:"(w1373) -> ()
                            n820 = local write "Run Time:"(w1372) -> ()
                            n821 = local write "Turbo OK"(w1371) -> ()
                            n822 = local write "Configuration:"(w1374) -> ()
                            n823 = Unbundle By Name(w1370) -> ("Frequency"=w1369:u16, "Decel"=w1368:bool, "Accel"=w1367:bool, "Normal \nOperation"=w1366:bool, "Turning"=w1365:bool, "BearingTemp"=w1364:u32, "MotorTemp"=w1363:u32, "ControllerTemp"=w1362:u16, "PumpStatus"=w1361:u16, "NumErrors"=w1360:u32, "NumOverload"=w1359:u32, "NumFailure"=w1358:u32)
                            n824 = local write "Frequency (Hz):"(w1369) -> ()
                            n825 = local write "Decel"(w1368) -> ()
                            n826 = local write "Accel"(w1367) -> ()
                            n827 = local write "Normal \nOperation"(w1366) -> ()
                            n828 = local write "Turning"(w1365) -> ()
                            n829 = local write "Bearing Temperature:"(w1364) -> ()
                            n830 = local write "Moter Temperature:"(w1363) -> ()
                            n831 = local write "Controller Temperature:"(w1362) -> ()
                            n832 = local write "PumpStatus"(w1361) -> ()
                            n833 = local write "Total Number of Errors:"(w1360) -> ()
                            n834 = local write "Number of Pressure Overload Errors:"(w1359) -> ()
                            n835 = local write "Number of Power Failures:"(w1358) -> ()
                          }
                          frame #3 {
                            n836 = call <vilib>:"Unset Busy.vi"() -> ()  [unwired: 2 in, 10 out]
                          }
                        }
                      }
                      frame True {
                      }
                    }
                  }
                  event "LBPump": Value Change {
                    n837 = event-data() -> ()  [unwired: 2 out]
                    n838 = Unbundle By Name(w1378) -> ("Running"=w1377:bool)
                    n839 = case shown="False" w1377 {
                      frame False {
                        n840 = stacked-sequence {
                          frame #0 {
                            n841 = call <vilib>:"Set Busy.vi"() -> ()  [unwired: 4 in, 8 out]
                          }
                          frame #1 {
                            w1382 = 1 ("disabled index (col)")
                            n842 = local read "Configuration:"() -> (w1385:string[][])
                            n843 = call "_Remote Get Leybold Status.vi"("UpdatePump"=TRUE) -> ("Configuration:"=w1388:string[][])  [unwired: 5 in, 5 out]
                            n844 = Index Array(array=w1388, index (col)=1 ("disabled index (col)")) -> (element=w1386:string[])  [unwired: 1 in]
                            n845 = Index Array(array=w1386) -> (element #1=w1381:string, element #2=w1380:string)  [unwired: 2 in]
                            n846 = Replace Array Subset(array=w1385, new element=w1381, index (row)=0, index (col)=w1382) -> (w1383:string[][])
                            n847 = Replace Array Subset(array=w1383, new element=w1380, index (row)=w1382, index (col)=w1382) -> (w1379:string[][])
                            n848 = local write "Configuration:"(w1379) -> ()
                          }
                          frame #2 {
                            n849 = call <vilib>:"Unset Busy.vi"() -> ()  [unwired: 2 in, 10 out]
                          }
                        }
                      }
                      frame True {
                      }
                    }
                  }
                  event "Update Pumping": Value Change {
                    n850 = event-data() -> ()  [unwired: 2 out]
                    n851 = Unbundle By Name(w1391) -> ("Running"=w1390:bool)
                    n852 = case shown="False" w1390 {
                      frame False {
                        n853 = stacked-sequence {
                          frame #0 {
                            n854 = call <vilib>:"Set Busy.vi"() -> ()  [unwired: 4 in, 8 out]
                          }
                          frame #1 {
                            n855 = local write "Pumping:"(string[][] [] ("Error History")) -> ()
                          }
                          frame #2 {
                            n856 = call "_Remote Get Turbo Status.vi"("Update Pumping"=TRUE) -> ("Turbo OK"=w1393:bool, "Pumping:"=w1394:string[][])  [unwired: 4 in, 4 out]
                            n857 = local write "Turbo OK"(w1393) -> ()
                            n858 = local write "Pumping:"(w1394) -> ()
                          }
                          frame #3 {
                            n859 = call <vilib>:"Unset Busy.vi"() -> ()  [unwired: 2 in, 10 out]
                          }
                        }
                      }
                      frame True {
                      }
                    }
                  }
                  event "Update Temp": Value Change {
                    n860 = event-data() -> ()  [unwired: 2 out]
                    n861 = Unbundle By Name(w1397) -> ("Running"=w1396:bool)
                    n862 = case shown="False" w1396 {
                      frame False {
                        n863 = stacked-sequence {
                          frame #0 {
                            n864 = call <vilib>:"Set Busy.vi"() -> ()  [unwired: 4 in, 8 out]
                          }
                          frame #1 {
                            n865 = local write "Temperatures:"(string[][] [] ("Error History")) -> ()
                          }
                          frame #2 {
                            n866 = call "_Remote Get Turbo Status.vi"("Update Temp"=TRUE) -> ("Temperatures:"=w1399:string[][])  [unwired: 4 in, 5 out]
                            n867 = local write "Temperatures:"(w1399) -> ()
                          }
                          frame #3 {
                            n868 = call <vilib>:"Unset Busy.vi"() -> ()  [unwired: 2 in, 10 out]
                          }
                        }
                      }
                      frame True {
                      }
                    }
                  }
                  event "Update Power": Value Change {
                    n869 = event-data() -> ()  [unwired: 2 out]
                    n870 = Unbundle By Name(w1402) -> ("Running"=w1401:bool)
                    n871 = case shown="False" w1401 {
                      frame False {
                        n872 = stacked-sequence {
                          frame #0 {
                            n873 = call <vilib>:"Set Busy.vi"() -> ()  [unwired: 4 in, 8 out]
                          }
                          frame #1 {
                            n874 = local write "Power / Current:"(string[][] [] ("Error History")) -> ()
                          }
                          frame #2 {
                            n875 = call "_Remote Get Turbo Status.vi"("Update Power"=TRUE) -> ("Power / Current:"=w1404:string[][])  [unwired: 4 in, 5 out]
                            n876 = local write "Power / Current:"(w1404) -> ()
                          }
                          frame #3 {
                            n877 = call <vilib>:"Unset Busy.vi"() -> ()  [unwired: 2 in, 10 out]
                          }
                        }
                      }
                      frame True {
                      }
                    }
                  }
                  event "Update Error": Value Change {
                    n878 = event-data() -> ()  [unwired: 2 out]
                    n879 = Unbundle By Name(w1407) -> ("Running"=w1406:bool)
                    n880 = case shown="False" w1406 {
                      frame False {
                        n881 = stacked-sequence {
                          frame #0 {
                            n882 = call <vilib>:"Set Busy.vi"() -> ()  [unwired: 4 in, 8 out]
                          }
                          frame #1 {
                            n883 = call "_Remote Send Turbo Command.vi"("Pump Command"=_Pump_Parameter."Clear Error") -> ()  [unwired: 2 in, 5 out]
                            n884 = local write "Error History"(string[][] [] ("Error History")) -> ()
                          }
                          frame #2 {
                            n885 = call "_Remote Get Turbo Status.vi"("Update Error"=TRUE) -> ("Error History"=w1410:string[][])  [unwired: 4 in, 5 out]
                            n886 = local write "Error History"(w1410) -> ()
                          }
                          frame #3 {
                            n887 = call <vilib>:"Unset Busy.vi"() -> ()  [unwired: 2 in, 10 out]
                          }
                        }
                      }
                      frame True {
                      }
                    }
                  }
                  event "Export ADC": Value Change {
                    n888 = event-data() -> ()  [unwired: 2 out]
                    n889 = call "_Get File.vi"("For Write (T)"=TRUE, "select mode (new or existing)"=T26."new or existing file", "default name"="My ADC Table", "extension (isd)"="*.txt" ("pattern (all files)"), "prompt"="Please enter an export file name.") -> ("Seleted File"=w1412:path, "Succeeded"=w1413:bool)  [unwired: 1 in, 2 out]
                    n890 = case shown="True" w1413 {
                      tunnel: w1412 -> [_ w1420]
                      frame False {
                      }
                      frame True {
                        n891 = property on="ADC List" class="MCListbox (strict)"() -> ("ItemNames"=w1421:string[][])  [unwired: 2 in, 2 out]
                        n892 = call "_Export Table To Text File.vi"("2D data"=w1421, "file path (dialog if empty)"=w1420) -> ()  [unwired: 4 in, 3 out]
                      }
                    }
                  }
                  event "Edit ADC": Value Change {
                    n893 = event-data() -> ()  [unwired: 2 out]
                    n894 = call "_Launch Dynamic VI.vi"("VI Name"=path "Show ADC Readings.vi" ("name or relative path")) -> ()  [unwired: 4 out]
                  }
                  event "Edit Config": Value Change {
                    n895 = event-data() -> ()  [unwired: 7 out]
                    n896 = flat-sequence {
                      frame #0 {
                        n897 = call "Edit Configuration.vi"() -> ()  [unwired: 8 out]
                      }
                      frame #1 {
                        n898 = property on="Force Update Oscillators" class="Bool (strict)"("Val(Sgnl)"=TRUE ("Value (Signaling)")) -> ()  [unwired: 2 in, 2 out]
                      }
                    }
                  }
                  event "View Config": Value Change {
                    n899 = event-data() -> ()  [unwired: 2 out]
                    n900 = call "Configuration Viewer.vi"() -> ()  [unwired: 8 out]
                  }
                  event "Update PM", "M1RF": Value Change {
                    n901 = event-data() -> ()  [unwired: 2 out]
                    n902 = Unbundle By Name(w1428) -> ("Running"=w1427:bool)
                    n903 = case shown="False" w1427 {
                      frame False {
                        n904 = call "_Remote Park Mass.vi"("Q2 Park Mass"="Q2 Park Mass", "Q1 Park Mass"="Q1 Park Mass", "M1RF"="M1RF") -> ("error out"=w1431:errorcluster, "Q2 Park Mass Out"=w1432:dbl, "Q1 Park Mass Out"=w1433:dbl, "M1RF Out"=w1429:dbl)  [unwired: 1 in]
                        n905 = local write "Q2 Park Mass"(w1432) -> ()
                        n906 = local write "Q1 Park Mass"(w1433) -> ()
                        n907 = local write "M1RF"(w1429) -> ()
                        n908 = call "_Handle Error.vi"("error in (no error)"=w1431) -> ()  [unwired: 2 in, 5 out]
                      }
                      frame True {
                      }
                    }
                  }
                  event "FrequencyTuneSetup": Value Change {
                    n909 = event-data() -> ("NewVal"=w1436:bool)  [unwired: 1 out]
                    n910 = case shown="False" w1436 {
                      tunnel: w1438 -> [w1440 w1461]
                      tunnel: [w1441 w1460] -> w1437
                      frame False {
                        # "End Frequency Tuning"
                        n911 = flat-sequence {
                          tunnel: w1440 -> [w1442]
                          tunnel: [w1442] -> w1439
                          tunnel: [w1456] -> w1441
                          tunnel: w1439 -> [w1457]
                          frame #0 {
                            n912 = Current VI's Menubar() -> (w1443:refnum<k9>)
                            n913 = property on="Tab Control" class="TabCtl (strict)"("PageSelVis"=TRUE ("Page Selector Visible")) -> ()  [unwired: 2 in, 2 out]
                            n914 = Set Menu Item Info(7:"Save All Tables" ("item tag"), 9:TRUE ("enabled"), 11:w1443) -> (0:w1447:errorcluster, 3:w1446:refnum<k9>)  [unwired: 4 in]
                            n915 = Set Menu Item Info(7:"Load All Tables" ("item tag"), 8:w1447, 9:TRUE ("enabled"), 11:w1446) -> ()  [unwired: 3 in, 2 out]
                          }
                          frame #1 {
                            n916 = local read "M1RF"() -> (w1455:dbl)
                            n917 = Unbundle By Name(w1457) -> ("Configuration 2"=w1459:T18)
                            n918 = call "_Remote Park Mass.vi"("UseDefault (F)"=TRUE, "M1RF"=w1455) -> ("Q2 Park Mass Out"=w1452:dbl, "Q1 Park Mass Out"=w1451:dbl, "M1RF Out"=w1453:dbl)  [unwired: 2 in, 1 out]
                            n919 = Bundle By Name(cluster=w1457, "FrequencyTune"=FALSE) -> (w1456:T32)
                            n920 = global write "_Global Configuration.vi" "Configuration 2"(w1459) -> ()
                            n921 = local write "Q2 Park Mass"(w1452) -> ()
                            n922 = local write "Q1 Park Mass"(w1451) -> ()
                            n923 = local write "M1RF"(w1453) -> ()
                          }
                        }
                      }
                      frame True {
                        # "Start Frequency Tuning"
                        n924 = flat-sequence {
                          tunnel: w1461 -> [w1475]
                          tunnel: [w1474] -> w1464
                          tunnel: [w1473] -> w1463
                          tunnel: w1464 -> [w1476]
                          tunnel: w1463 -> [w1479]
                          tunnel: [w1476] -> w1462
                          tunnel: [w1492] -> w1460
                          tunnel: w1462 -> [w1502]
                          frame #0 {
                            n925 = global read "_Global Configuration.vi" "Configuration 2"() -> (w1473:T18)
                            n926 = Current VI's Menubar() -> (w1472:refnum<k9>)
                            n927 = Set Menu Item Info(7:"Save All Tables" ("item tag"), 9:FALSE ("enabled"), 11:w1472) -> (0:w1468:errorcluster, 3:w1469:refnum<k9>)  [unwired: 4 in]
                            n928 = Set Menu Item Info(7:"Load All Tables" ("item tag"), 8:w1468, 9:FALSE ("enabled"), 11:w1469) -> ()  [unwired: 3 in, 2 out]
                            n929 = Bundle By Name(cluster=w1475, "Configuration 2"=w1473) -> (w1474:T32)
                            n930 = property on="Tab Control" class="TabCtl (strict)"("PageSelVis"=FALSE ("Page Selector Visible")) -> ()  [unwired: 2 in, 2 out]
                          }
                          frame #1 {
                            n931 = Unbundle By Name(w1479) -> ("Table"=w1477:T19[])
                            n932 = for {
                              shift-right: [w1481] -> w1478
                              shift-left: w1477 -> [w1483]
                              tunnel: w1477 -> [_] mode=indexing
                              i -> [w1482]
                              n933 = in-place {
                                n934 = in-place-array #1(w1483, w1482) -> (w1485:T19)
                                n935 = Unbundle By Name(w1485) -> ("Name"=w1486:string)
                                n936 = case shown="\"M1 RF\", \"Q1 RF\", \"Q2 RF\"" w1486 {
                                tunnel: w1485 -> [w1487 w1490]
                                tunnel: [w1487 w1489] -> w1484
                                frame "False", Default {
                                }
                                frame "M1 RF", "Q1 RF", "Q2 RF" {
                                w1488 = 0.0 ("Def+")
                                n937 = Bundle By Name(cluster=w1490, "Def+"=w1488, "Def-"=w1488) -> (w1489:T19)
                                }
                                }
                                n938 = in-place-array #1(w1484) -> (w1481:T19[])  [unwired: 1 out]
                              }
                            }
                            n939 = Bundle By Name(cluster=w1479, "Table"=w1478) -> (w1480:T18)
                            n940 = global write "_Global Configuration.vi" "Configuration 2"(w1480) -> ()
                          }
                          frame #2 {
                            w1497 = 0.0 ("M1RF")
                            n941 = call "_Remote Park Mass.vi"("Q2 Park Mass"=w1497, "Q1 Park Mass"=w1497, "M1RF"=w1497) -> ("error out"=w1500:errorcluster, "Q2 Park Mass Out"=w1496:dbl, "Q1 Park Mass Out"=w1495:dbl, "M1RF Out"=w1494:dbl)  [unwired: 1 in]
                            n942 = local write "Q2 Park Mass"(w1496) -> ()
                            n943 = local write "Q1 Park Mass"(w1495) -> ()
                            n944 = local write "M1RF"(w1494) -> ()
                            n945 = local read "Oscillator Settings"() -> (w1493:string[][])
                            n946 = Bundle By Name(cluster=w1502, "FrequencyTune"=TRUE) -> (w1492:T32)
                            n947 = call "_Remote Communicate.vi"("error in (no error)"=w1500, "DC Param"=u16 0, "Command"=_RT_Command."Toggle Power") -> ("error out"=w1501:errorcluster)  [unwired: 3 in, 3 out]
                            n948 = property on="Oscillator Settings" class="Tbl (strict)"("Val(Sgnl)"=w1493) -> ()  [unwired: 2 in, 2 out]
                            n949 = call "_Handle Error.vi"("error in (no error)"=w1501) -> ()  [unwired: 2 in, 5 out]
                          }
                        }
                      }
                    }
                  }
                  event "Tab Control": Value Change {
                    n950 = event-data() -> ("OldVal"=w1513:T2)  [unwired: 1 out]
                    n951 = Unbundle By Name(w1504) -> ("Running"=w1511:bool, "Update"=w1510:bool)
                    n952 = Not Equal?(x=w1513, y=T27."QDC & Tuning" ("Tab Control")) -> (x != y?=w1508:bool)
                    n953 = Not(x=w1510) -> (.not. x?=w1509:bool)
                    n954 = And(x=w1509, y=w1508) -> (x .and. y?=w1507:bool)
                    n955 = case shown="Default" "Tab Control" {
                      frame Default {
                      }
                      frame "Leybold 3QS" {
                        n956 = property on="LBFreqTemp" class="Bool (strict)"("Val(Sgnl)"=TRUE ("Value (Signaling)")) -> ()  [unwired: 2 in, 2 out]
                      }
                      frame "Tables" {
                        n957 = property on="Table Choice" class="RadioBtnsControl (strict)"("Val(Sgnl)"="Table Choice") -> ()  [unwired: 2 in, 2 out]
                      }
                    }
                    n958 = Or(x=w1511, y=w1507) -> (x .or. y?=w1512:bool)
                    n959 = case shown="False" w1512 {
                      tunnel: w1504 -> [w1518 w1548]
                      tunnel: [w1517 w1548] -> w1503
                      frame False {
                        w1522 = 0 ("index (row)")
                        w1523 = string[][] [["400"], ["0"], ["0"]] ("Value (Signaling)")
                        n960 = flat-sequence {
                          tunnel: [w1535] -> w1516
                          tunnel: w1518 -> [w1535]
                          tunnel: [w1547] -> w1517
                          tunnel: w1516 -> [w1547]
                          frame #0 {
                            n961 = global read "_Global Configuration.vi" "Configuration 2"() -> (w1534:T18)
                            n962 = Unbundle By Name(w1534) -> ("Table"=w1533:T19[])
                            n963 = for {
                              tunnel: w1533 -> [w1537] mode=indexing
                              n964 = Unbundle By Name(w1537) -> ("Name"=w1538:string, "Def+"=w1536:dbl)
                              n965 = case shown="\"Q2 RF\"" w1538 {
                                tunnel: w1536 -> [_ w1539 w1540 w1541]
                                frame "False", Default {
                                }
                                frame "Q2 RF" {
                                (unwired) 0.0 ("Def+")
                                n966 = local write "Q2 Park Mass"(w1539) -> ()
                                }
                                frame "M1 RF" {
                                n967 = local write "M1RF"(w1540) -> ()
                                }
                                frame "Q1 RF" {
                                n968 = local write "Q1 Park Mass"(w1541) -> ()
                                }
                              }
                            }
                          }
                          frame #1 {
                            # "Reset the park mass to default"
                            n969 = local read "M1RF"() -> (w1546:dbl)
                            n970 = call "_Remote Park Mass.vi"("UseDefault (F)"=TRUE, "M1RF"=w1546) -> ("Q2 Park Mass Out"=w1543:dbl, "Q1 Park Mass Out"=w1542:dbl, "M1RF Out"=w1544:dbl)  [unwired: 2 in, 1 out]
                            n971 = local write "Q2 Park Mass"(w1543) -> ()
                            n972 = local write "Q1 Park Mass"(w1542) -> ()
                            n973 = local write "M1RF"(w1544) -> ()
                          }
                        }
                        n974 = call "_Get Lens Configuration.vi"("Channel #"=u8 4) -> ("Lens Configuration"=w1531:T19)  [unwired: 1 in, 5 out]
                        n975 = call "_Get Lens Configuration.vi"("Channel #"=u8 5) -> ("Lens Configuration"=w1530:T19)  [unwired: 1 in, 5 out]
                        n976 = Unbundle By Name(w1531) -> ("Def+"=w1528:dbl)
                        n977 = Unbundle By Name(w1530) -> ("Def+"=w1525:dbl)
                        n978 = Number To Fractional String(number=w1528, precision (6)=i16 0) -> (F-format string=w1524:string)  [unwired: 2 in]
                        n979 = Number To Fractional String(number=w1525, precision (6)=i16 0) -> (F-format string=w1521:string)  [unwired: 2 in]
                        n980 = Replace Array Subset(array=w1523, new element=w1524, index (row)=w1522, index (col)=w1522) -> (w1519:string[][])
                        n981 = Replace Array Subset(array=w1523, new element=w1521, index (row)=w1522, index (col)=w1522) -> (w1520:string[][])
                        n982 = property on="Q1 DC Inputs" class="Tbl (strict)"("Val(Sgnl)"=w1519) -> ()  [unwired: 2 in, 2 out]
                        n983 = property on="Q2 DC Inputs" class="Tbl (strict)"("Val(Sgnl)"=w1520) -> ()  [unwired: 2 in, 2 out]
                      }
                      frame True {
                      }
                    }
                  }
                  event "Options": Value Change {
                    w1550 = cluster{u32, u32}[] [{16711680, 16711680}, {10421504, 10421504}, {8323072, 8323072}, {5177856, 5177856}]  # RedColor
                    w1551 = cluster{u32, u32}[] [{12369084, 12369084}, {9868950, 9868950}, {12369084, 12369084}, {9868950, 9868950}]  # GrayColor
                    n984 = event-data() -> ()  [unwired: 2 out]
                    n985 = call "Start Up Options.vi"("No PW Needed (F)"=TRUE) -> ("All On"=w1552:bool)  [unwired: 6 out]
                    n986 = Select(t=w1551, s=w1552, f=w1550) -> (s? t:f=w1549:cluster{u32, u32}[])
                    n987 = property on="Options" class="Bool"("Colors [4]"=w1549) -> ()  [unwired: 2 in, 2 out]
                  }
                  event "Adjust Cal Tables": Value Change {
                    # "#EHSM-380: Remove useless boxes from QDC Tuning Tab"
                    n988 = event-data() -> ()  [unwired: 2 out]
                    n989 = disable-structure shown="Disabled" {
                      disable-tunnel: w1556 -> [w1559 w1579]
                      disable-tunnel: [w1558 w1579] -> w1555
                      frame Disabled {
                        n990 = local read "New Frequence"() -> (w1561:dbl)
                        n991 = local read "Old Frequency"() -> (w1562:dbl)
                        n992 = Divide(x=w1561, y=w1562) -> (x/y=w1563:dbl)
                        n993 = Square(x=w1563) -> (x^2=w1560:dbl)
                        n994 = stacked-sequence {
                          tunnel: w1560 -> [w1566 w1569 w1572 w1575 _]
                          frame #0 {
                            n995 = global read "_Global Configuration.vi" "Calibration"() -> (w1565:dbl[][])
                            n996 = call "_Adjust Calibration Table.vi"("Calibration Table In"=w1565, "Adjustment Factor"=w1566) -> ("Calibration Table Out"=w1564:dbl[][])
                            n997 = global write "_Global Configuration.vi" "Calibration"(w1564) -> ()
                          }
                          frame #1 {
                            n998 = global read "_Global Configuration.vi" "Calibration 2"() -> (w1568:dbl[][])
                            n999 = call "_Adjust Calibration Table.vi"("Calibration Table In"=w1568, "Adjustment Factor"=w1569) -> ("Calibration Table Out"=w1567:dbl[][])
                            n1000 = global write "_Global Configuration.vi" "Calibration 2"(w1567) -> ()
                          }
                          frame #2 {
                            n1001 = global read "_Global Configuration.vi" "Calibration 3"() -> (w1571:dbl[][])
                            n1002 = call "_Adjust Calibration Table.vi"("Calibration Table In"=w1571, "Adjustment Factor"=w1572) -> ("Calibration Table Out"=w1570:dbl[][])
                            n1003 = global write "_Global Configuration.vi" "Calibration 3"(w1570) -> ()
                          }
                          frame #3 {
                            n1004 = global read "_Global Configuration.vi" "Calibration 4"() -> (w1574:dbl[][])
                            n1005 = call "_Adjust Calibration Table.vi"("Calibration Table In"=w1574, "Adjustment Factor"=w1575) -> ("Calibration Table Out"=w1573:dbl[][])
                            n1006 = global write "_Global Configuration.vi" "Calibration 4"(w1573) -> ()
                          }
                          frame #4 {
                            n1007 = for {
                              N: 4 -> [_]
                              i -> [w1577]
                              n1008 = call "_Remote Communicate.vi"("DC Param"=w1577, "Command"=_RT_Command."Update Table") -> ()  [unwired: 4 in, 4 out]
                            }
                          }
                        }
                        n1009 = Bundle By Name(cluster=w1559, "CalAjusted"=TRUE) -> (w1558:T32)
                      }
                      frame Enabled {
                      }
                    }
                  }
                  event "Table Choice": Value Change {
                    n1010 = event-data() -> ("NewVal"=w1580:T8)  [unwired: 1 out]
                    n1011 = case shown="\"Low Resolution\"" w1580 {
                      tunnel: [w1590 w1591 w1592 w1593] -> w1581
                      frame "Calibration", Default {
                        w1590 = u16[] [0, 1, 2, 3] items=["Q1 +ve Mass Calibration Table", "Q2 +ve Mass Calibration Table", "Q1 -ve Mass Calibration Table", "Q2 -ve Mass Calibration Table", "Q1 +ve High Resolution Table", "Q2 +ve High Resolution Table", "Q1 +ve Medium Resolution Table", "Q2 +ve Medium Resolution Table", "Q1 +ve Low Resolution Table", "Q2 +ve Low Resolution Table", "Q1 -ve High Resolution Table", "Q2 -ve High Resolution Table", "Q1 -ve Medium Resolution Table", "Q2 -ve Medium Resolution Table", "Q1 -ve Low Resolution Table", "Q2 -ve Low Resolution Table"]
                      }
                      frame "Low Resolution" {
                        w1591 = u16[] [8, 9, 14, 15] items=["Q1 +ve Mass Calibration Table", "Q2 +ve Mass Calibration Table", "Q1 -ve Mass Calibration Table", "Q2 -ve Mass Calibration Table", "Q1 +ve High Resolution Table", "Q2 +ve High Resolution Table", "Q1 +ve Medium Resolution Table", "Q2 +ve Medium Resolution Table", "Q1 +ve Low Resolution Table", "Q2 +ve Low Resolution Table", "Q1 -ve High Resolution Table", "Q2 -ve High Resolution Table", "Q1 -ve Medium Resolution Table", "Q2 -ve Medium Resolution Table", "Q1 -ve Low Resolution Table", "Q2 -ve Low Resolution Table"]
                      }
                      frame "Unit Resolution" {
                        w1592 = u16[] [6, 7, 12, 13] items=["Q1 +ve Mass Calibration Table", "Q2 +ve Mass Calibration Table", "Q1 -ve Mass Calibration Table", "Q2 -ve Mass Calibration Table", "Q1 +ve High Resolution Table", "Q2 +ve High Resolution Table", "Q1 +ve Medium Resolution Table", "Q2 +ve Medium Resolution Table", "Q1 +ve Low Resolution Table", "Q2 +ve Low Resolution Table", "Q1 -ve High Resolution Table", "Q2 -ve High Resolution Table", "Q1 -ve Medium Resolution Table", "Q2 -ve Medium Resolution Table", "Q1 -ve Low Resolution Table", "Q2 -ve Low Resolution Table"]
                      }
                      frame "High Resolution" {
                        w1593 = u16[] [4, 5, 10, 11] items=["Q1 +ve Mass Calibration Table", "Q2 +ve Mass Calibration Table", "Q1 -ve Mass Calibration Table", "Q2 -ve Mass Calibration Table", "Q1 +ve High Resolution Table", "Q2 +ve High Resolution Table", "Q1 +ve Medium Resolution Table", "Q2 +ve Medium Resolution Table", "Q1 +ve Low Resolution Table", "Q2 +ve Low Resolution Table", "Q1 -ve High Resolution Table", "Q2 -ve High Resolution Table", "Q1 -ve Medium Resolution Table", "Q2 -ve Medium Resolution Table", "Q1 -ve Low Resolution Table", "Q2 -ve Low Resolution Table"]
                      }
                    }
                    n1012 = for {
                      tunnel: w1581 -> [w1585] mode=indexing
                      i -> [w1584]
                      n1013 = case shown="3" w1584 {
                        tunnel: [w1586 w1587 w1588 w1589] -> w1583
                        frame 0, Default {
                          n1014 = control-ref of="Table 1"() -> (w1586:refnum<vi>)
                        }
                        frame 1 {
                          n1015 = control-ref of="Table 2"() -> (w1587:refnum<vi>)
                        }
                        frame 2 {
                          n1016 = control-ref of="Table 3"() -> (w1588:refnum<vi>)
                        }
                        frame 3 {
                          n1017 = control-ref of="Table 4"() -> (w1589:refnum<vi>)
                        }
                      }
                      n1018 = call "_Display Calibration Table.vi"("Table Ref"=w1583, "Table Type"=w1585) -> ()  [unwired: 1 out]
                    }
                  }
                }
              }
              n1019 = while {
                shift-right: [w327] -> _
                shift-left: FALSE -> [w331]
                shift-right: [w325] -> _
                shift-left: w246 -> [w323]
                tunnel: w252 -> [w326]
                shift-left: w246 -> [w322]
                stop <- w328 stop-if-true
                n1020 = local read "Running"() -> (w332:bool)
                n1021 = local read "Quit"() -> (w329:bool)
                n1022 = global read "_Global Configuration.vi" "Quit"() -> (w330:bool)
                n1023 = Wait (ms)(milliseconds to wait=u32 280) -> ()  [unwired: 1 out]
                n1024 = Or(x=w330, y=w329) -> (x .or. y?=w328:bool)
                n1025 = case shown="False" w332 {
                  tunnel: w331 -> [w361 w376]
                  tunnel: w328 -> [w359 _]
                  tunnel: [w348 w376] -> w327
                  tunnel: [w356 w375] -> w325
                  tunnel: w323 -> [w357 w375]
                  tunnel: w326 -> [w350 _]
                  frame False {
                    n1026 = global read "_Global Configuration.vi" "Run"() -> (w360:bool)
                    n1027 = Or(x=w360, y=w359) -> (x .or. y?=w358:bool)
                    n1028 = case shown="False" w358 {
                      tunnel: w361 -> [w372 w374]
                      tunnel: [w371 w373] -> w356
                      tunnel: [w370 w374] -> w348
                      tunnel: w357 -> [_ w373]
                      frame False {
                        n1029 = call "_Remote Get RT Status.vi"("RT Ready"=w372) -> ("InstrState"=w371:T1, "RT Ready Out"=w370:bool)  [unwired: 1 in, 1 out]
                      }
                      frame True {
                      }
                    }
                    n1030 = global read "_Global Configuration.vi" "TCP"() -> (w351:bool)
                    n1031 = Select(t="- Connected", s=w351, f="- Simulation") -> (s? t:f=w365:string)
                    n1032 = Not Equal?(x=w356, y=w357) -> (x != y?=w354:bool)
                    n1033 = Equal?(x=w356, y=_RT_Instrument_State."Ready") -> (x = y?=w353:bool)
                    n1034 = Format Into String(format string=" %s, (state = %s)", initial string=w350, w365, w356) -> (resulting string=w349:string)  [unwired: 1 in, 1 out]
                    n1035 = And(x=w354, y=w353) -> (x .and. y?=w352:bool)
                    n1036 = case shown="True" w352 {
                      frame False {
                      }
                      frame True {
                        n1037 = property on="Load Tune File" class="Bool (strict)"("Val(Sgnl)"=FALSE ("Value (Signaling)")) -> ()  [unwired: 2 in, 2 out]
                        n1038 = call <vilib>:"Application Directory.vi"() -> ("Application Directory"=w366:path)
                        n1039 = Build Path(base path=w366, name or relative path="DEFAULT_SETTINGS.d2m") -> (appended path=w367:path)
                        n1040 = local write "Tune File"(w367) -> ()
                      }
                    }
                    n1041 = property class="VI"("Front Panel Window:Title"=w349) -> ()  [unwired: 2 in, 2 out]
                    n1042 = local write "Version"(w349) -> ()
                    n1043 = global write "_Global Configuration.vi" "RT Ready"(w348) -> ()
                  }
                  frame True {
                    # "Start Health Check Squence"
                    n1044 = stacked-sequence {
                      frame #0 {
                        n1045 = local write "Progress Bar"(u8 1 ("ProgressBar")) -> ()
                        n1046 = call <vilib>:"Application Directory.vi"() -> ("Application Directory"=w377:path)
                        n1047 = Build Path(base path=w377, name or relative path="TEST_ALL.d2m") -> (appended path=w380:path)
                        n1048 = local write "Tune File"(w380) -> ()
                      }
                      frame #1 {
                        n1049 = property on="Load Tune File" class="Bool (strict)"("Val(Sgnl)"=FALSE ("Value (Signaling)")) -> ()  [unwired: 2 in, 2 out]
                      }
                      frame #2 {
                        w383 = TRUE
                        # "Firmware Check"
                        n1050 = local read "Running"() -> (w382:bool)
                        n1051 = case shown="True" w382 {
                          tunnel: w383 -> [_ w386]
                          frame False {
                          }
                          frame True {
                            n1052 = property on="Refresh" class="Bool (strict)"("Val(Sgnl)"=w386) -> ()  [unwired: 2 in, 2 out]
                            n1053 = Wait (ms)(milliseconds to wait=u32 800) -> ()  [unwired: 1 out]
                          }
                        }
                        n1054 = property on="Firmware OK" class="Bool (strict)"("Visible"=w383) -> ()  [unwired: 2 in, 2 out]
                        n1055 = local write "Progress Bar"(u8 2 ("ProgressBar")) -> ()
                      }
                      frame #3 {
                        # "this was 2"
                        n1056 = local write "Progress Bar"(u8 14 ("ProgressBar")) -> ()
                        n1057 = local read "Running"() -> (w387:bool)
                        n1058 = case shown="True" w387 {
                          frame False {
                          }
                          frame True {
                            n1059 = global read "_Global Configuration.vi" "UseLeybold"() -> (w389:bool)
                            n1060 = case shown="False" w389 {
                              tunnel: TRUE -> [w391 w394]
                              frame False {
                                n1061 = call "_Remote Get Turbo Status.vi"("Update Info"=w391) -> ("Pump Info:"=w392:string[][])  [unwired: 4 in, 5 out]
                                n1062 = local write "Pump Info:"(w392) -> ()
                              }
                              frame True {
                                n1063 = call "_Remote Get Leybold Status.vi"("UpdateConfig"=w394) -> ("Configuration:"=w393:string[][])  [unwired: 5 in, 5 out]
                                n1064 = local write "Configuration:"(w393) -> ()
                              }
                            }
                          }
                        }
                      }
                      frame #4 {
                        # "this was 3"
                        n1065 = global read "_Global Configuration.vi" "UseLeybold"() -> (w398:bool)
                        n1066 = local write "Progress Bar"(u8 20 ("ProgressBar")) -> ()
                        n1067 = local read "Running"() -> (w396:bool)
                        n1068 = Not(x=w398) -> (.not. x?=w397:bool)
                        n1069 = And(x=w396, y=w397) -> (x .and. y?=w395:bool)
                        n1070 = case shown="True" w395 {
                          frame False {
                          }
                          frame True {
                            n1071 = call "_Remote Get Turbo Status.vi"("Update Pumping"=TRUE) -> ("Turbo OK"=w403:bool, "Pumping:"=w402:string[][])  [unwired: 4 in, 4 out]
                            n1072 = local write "Turbo OK"(w403) -> ()
                            n1073 = local write "Pumping:"(w402) -> ()
                          }
                        }
                        n1074 = property on="Turbo OK" class="Bool (strict)"("Visible"=TRUE) -> ()  [unwired: 2 in, 2 out]
                      }
                      frame #5 {
                        n1075 = global read "_Global Configuration.vi" "UseLeybold"() -> (w407:bool)
                        n1076 = local read "Running"() -> (w405:bool)
                        n1077 = local write "Progress Bar"(u8 35 ("ProgressBar")) -> ()
                        n1078 = Not(x=w407) -> (.not. x?=w406:bool)
                        n1079 = And(x=w405, y=w406) -> (x .and. y?=w404:bool)
                        n1080 = case shown="True" w404 {
                          frame False {
                          }
                          frame True {
                            n1081 = call "_Remote Get Turbo Status.vi"("Update Temp"=TRUE) -> ("Temperatures:"=w410:string[][])  [unwired: 4 in, 5 out]
                            n1082 = local write "Temperatures:"(w410) -> ()
                          }
                        }
                      }
                      frame #6 {
                        n1083 = global read "_Global Configuration.vi" "UseLeybold"() -> (w414:bool)
                        n1084 = local read "Running"() -> (w412:bool)
                        n1085 = local write "Progress Bar"(u8 40 ("ProgressBar")) -> ()
                        n1086 = Not(x=w414) -> (.not. x?=w413:bool)
                        n1087 = And(x=w412, y=w413) -> (x .and. y?=w411:bool)
                        n1088 = case shown="True" w411 {
                          frame False {
                          }
                          frame True {
                            n1089 = call "_Remote Get Turbo Status.vi"("Update Power"=TRUE) -> ("Power / Current:"=w417:string[][])  [unwired: 4 in, 5 out]
                            n1090 = local write "Power / Current:"(w417) -> ()
                          }
                        }
                      }
                      frame #7 {
                        n1091 = local read "Running"() -> (w419:bool)
                        n1092 = global read "_Global Configuration.vi" "UseLeybold"() -> (w418:bool)
                        n1093 = local write "Progress Bar"(u8 65 ("ProgressBar")) -> ()
                        n1094 = case shown="True" w419 {
                          tunnel: w418 -> [_ w421]
                          frame False {
                          }
                          frame True {
                            n1095 = case shown="True" w421 {
                              frame False {
                                n1096 = call "_Remote Get Turbo Status.vi"("Update Error"=TRUE) -> ("Error History"=w423:string[][])  [unwired: 4 in, 5 out]
                                n1097 = local write "Error History"(w423) -> ()
                              }
                              frame True {
                                w424 = TRUE
                                n1098 = call "_Remote Get Leybold Status.vi"("UpdateError"=w424, "UpdateRunTime"=w424, "UpdatePower"=w424, "UpdateOthers"=w424) -> ("Run Time:"=w439:string[][], "Power:"=w440:string[][], "OtherInfo"=w437:T38, "Turbo OK"=w438:bool, "Errors:"=w441:string[][])  [unwired: 2 in, 1 out]
                                n1099 = local write "Errors:"(w441) -> ()
                                n1100 = local write "Power:"(w440) -> ()
                                n1101 = local write "Run Time:"(w439) -> ()
                                n1102 = local write "Turbo OK"(w438) -> ()
                                n1103 = Unbundle By Name(w437) -> ("Frequency"=w436:u16, "Decel"=w435:bool, "Accel"=w434:bool, "Normal \nOperation"=w433:bool, "Turning"=w432:bool, "BearingTemp"=w431:u32, "MotorTemp"=w430:u32, "ControllerTemp"=w429:u16, "PumpStatus"=w428:u16, "NumErrors"=w427:u32, "NumOverload"=w426:u32, "NumFailure"=w425:u32)
                                n1104 = local write "Frequency (Hz):"(w436) -> ()
                                n1105 = local write "Decel"(w435) -> ()
                                n1106 = local write "Accel"(w434) -> ()
                                n1107 = local write "Normal \nOperation"(w433) -> ()
                                n1108 = local write "Turning"(w432) -> ()
                                n1109 = local write "Bearing Temperature:"(w431) -> ()
                                n1110 = local write "Moter Temperature:"(w430) -> ()
                                n1111 = local write "Controller Temperature:"(w429) -> ()
                                n1112 = local write "PumpStatus"(w428) -> ()
                                n1113 = local write "Total Number of Errors:"(w427) -> ()
                                n1114 = local write "Number of Pressure Overload Errors:"(w426) -> ()
                                n1115 = local write "Number of Power Failures:"(w425) -> ()
                              }
                            }
                          }
                        }
                      }
                      frame #8 {
                        w442 = TRUE
                        # "SVG Check"
                        # "Voltage Check"
                        n1116 = local write "Progress Bar"(u8 70 ("ProgressBar")) -> ()
                        n1117 = property on="SVG OK" class="Bool (strict)"("Visible"=w442) -> ()  [unwired: 2 in, 2 out]
                        n1118 = property on="Voltage OK" class="Bool (strict)"("Visible"=w442) -> ()  [unwired: 2 in, 2 out]
                      }
                      frame #9 {
                        # "Interlock Check"
                        n1119 = local write "Progress Bar"(u8 75 ("ProgressBar")) -> ()
                        n1120 = property on="Intlk/Per OK" class="Bool (strict)"("Visible"=TRUE) -> ()  [unwired: 2 in, 2 out]
                      }
                      frame #10 {
                        # "Done Quad Check"
                        n1121 = local write "Progress Bar"(u8 95 ("ProgressBar")) -> ()
                        n1122 = property on="Quad/Tune OK" class="Bool (strict)"("Visible"=TRUE) -> ()  [unwired: 2 in, 2 out]
                      }
                      frame #11 {
                        # "Finish Run"
                        n1123 = local write "Running"(FALSE ("Unit")) -> ()
                        n1124 = property on="Cancel" class="Bool (strict)"("Val(Sgnl)"=TRUE ("Value (Signaling)")) -> ()  [unwired: 2 in, 2 out]
                        n1125 = local write "Progress Bar"(u8 100 ("ProgressBar")) -> ()
                      }
                    }
                  }
                }
                "MS State" <- w325
                n1126 = Not Equal?(x=w323, y=w322) -> (x != y?=w324:bool)
                n1127 = global write "_Global Configuration.vi" "MS State"(w325) -> ()
                n1128 = case shown="True" w324 {
                  tunnel: w323 -> [_ w341]
                  frame False {
                  }
                  frame True {
                    n1129 = Equal?(x=w341, y=_RT_Instrument_State."Ready") -> (x = y?=w337:bool)
                    n1130 = Equal?(x=w341, y=_RT_Instrument_State."Mass Spectrometer is Off") -> (x = y?=w338:bool)
                    n1131 = Current VI's Menubar() -> (w334:refnum<k9>)
                    n1132 = Or(x=w337, y=w338) -> (x .or. y?=w336:bool)
                    n1133 = case shown="False" w336 {
                      tunnel: "Goto Roughing Pump On Standby" ("item name") -> [w344 w347]
                      tunnel: w334 -> [w343 w346]
                      frame True {
                        n1134 = Set Menu Item Info(7:w344, 9:TRUE ("enabled"), 11:w343) -> ()  [unwired: 4 in, 2 out]
                      }
                      frame False {
                        n1135 = Set Menu Item Info(7:w347, 9:FALSE ("enabled"), 11:w346) -> ()  [unwired: 4 in, 2 out]
                      }
                    }
                  }
                }
              }
              n1136 = while {
                tunnel: w251 -> [w273]
                tunnel: w248 -> [w274]
                tunnel: [w270] -> w250
                tunnel: [w269] -> w249
                stop <- w275 stop-if-true
                # "Command Q"
                n1137 = Dequeue Element(queue=w273, timeout in ms (-1)=280, error in (no error)=w274) -> (queue out=w269:refnum<queue>, element=w272:cluster{"Command":string, "Data":variant}, timed out?=w268:bool, error out=w267:errorcluster)
                n1138 = Or(x=w267, y=w268) -> (x .or. y?=w266:bool)
                n1139 = case shown="False" w266 {
                  tunnel: w267 -> [w279 w321]
                  tunnel: w272 -> [w282 _]
                  tunnel: [w278 w321] -> w270
                  frame False {
                    # "New Command"
                    n1140 = Unbundle(w282) -> ("Command"=w280:string, "Data"=w281:variant)
                    n1141 = case shown="\"Print\"" w280 {
                      tunnel: w281 -> [_ w294]
                      tunnel: w279 -> [w283 w311]
                      tunnel: [w283 w298] -> w278
                      frame Default {
                        # "unknown command"
                      }
                      frame "Print" {
                        w303 = 1 items=["portrait", "landscape"] ("orientation (portrait)")
                        # "the report generation Quick print causes the VI to freeze while the screenshot is taken\nwhich causes a FW dropped connection. Getting a scaled image here, and passing it to the report generation\nneed a scaled image as report generator is not scaling the image properly"
                        # "Print Command"
                        n1142 = Variant To Data(error in=w311, type=T21 {"Picture Name"="", "VI Reference"=refnum} ("Cluster"), Variant=w294) -> (data=w293:T21, error out=w296:errorcluster)
                        n1143 = Unbundle By Name(w293) -> ("Picture Name"=w292:string, "VI Reference"=w291:refnum<vi>)
                        n1144 = invoke class="VI" method="FP.Get Image Scaled"(reference=w291, "visible area only"=TRUE ("Visible Area Only"), "max width"=1100 ("Maximum Width"), "max height"=579 ("Maximum Height")) -> ("image data"=w312:T39)  [unwired: 4 in, 7 out]
                        n1145 = call <vilib>:"Application Directory.vi"() -> ("Application Directory"=w310:path)
                        n1146 = Build Path(base path=w310, name or relative path=w292) -> (appended path=w309:path)
                        n1147 = call <vilib>:"Write JPEG File.vi"("error in (no error)"=w296, "image data"=w312, "path to JPEG file"=w309) -> ("error out"=w300:errorcluster, "path"=w297:path)  [unwired: 7 out]
                        n1148 = call <vilib>:"New Report.vi"("report type"=T22."Standard Report", "error in (no error)"=w300) -> ("report out"=w304:refnum<class "NI_report.lvclass">, "error out"=w307:errorcluster)  [unwired: 12 in]
                        n1149 = call-dynamic "Set Report Orientation.vi"("report in"=w304, "orientation (portrait)"=w303, "error in (no error)"=w307) -> ("report out"=w306:refnum<class "NI_report.lvclass">, "error out"=w308:errorcluster)  [unwired: 11 in]
                        n1150 = call-poly <vilib>:"Append Image to Report.vi"("report in"=w306, "path or URL of image"=w297, "error in (no error)"=w308) -> ("report out"=w286:refnum<class "NI_report.lvclass">, "error out"=w288:errorcluster)  [unwired: 9 in, 2 out]
                        n1151 = call-dynamic "Set Report Margins.vi"("report in"=w286, "margins (1.00)"=T20 {"top"=0.1, "left"=0.1, "right"=0.1, "bottom"=0.1}, "error in (no error)"=w288) -> ("report out"=w285:refnum<class "NI_report.lvclass">, "error out"=w287:errorcluster)  [unwired: 10 in, 1 out]
                        n1152 = call "SelectPrinter.vi"() -> ("ChosenPrinter"=w302:string, "Closed?"=w301:bool)  [unwired: 2 in]
                        n1153 = case shown="False" w301 {
                          tunnel: w285 -> [w319 _]
                          tunnel: w302 -> [w317 _]
                          tunnel: w287 -> [w316 w320]
                          tunnel: [w314 w320] -> w299
                          frame False {
                            n1154 = call-dynamic "Print Report.vi"("report in"=w319, "printer name (default)"=w317, "error in (no error)"=w316) -> ("report out"=w318:refnum<class "NI_report.lvclass">, "error out"=w315:errorcluster)  [unwired: 11 in]
                            n1155 = call-dynamic "Dispose Report.vi"("report in"=w318, "error in (no error)"=w315) -> ("error out"=w314:errorcluster)  [unwired: 13 in]
                          }
                          frame True {
                          }
                        }
                        n1156 = Delete(path (use dialog)=w297, error in=w299) -> (error out=w298:errorcluster)  [unwired: 3 in, 2 out]
                      }
                    }
                  }
                  frame True {
                    # "Timeout/Error"
                  }
                }
                n1157 = local read "Quit"() -> (w277:bool)
                n1158 = global read "_Global Configuration.vi" "Quit"() -> (w276:bool)
                n1159 = Or(x=w276, y=w277) -> (x .or. y?=w275:bool)
              }
              n1160 = Release Queue(queue=w249, error in (no error)=w250) -> ()  [unwired: 1 in, 3 out]
            }
            frame #5 {
              n1161 = Release Queue(queue=w1658) -> ()  [unwired: 1 in, 4 out]
              n1162 = Initialize Array("", 16 ("dimension size")) -> (w1648:string[])
              n1163 = global read "_Global Configuration.vi" "Configuration 2"() -> (w1651:T18)
              n1164 = Unbundle By Name(w1651) -> ("Instrument"=w1650:string[])
              n1165 = local read "LoadedTable"() -> (w1656:bool)
              n1166 = Index Array(array=w1652, index #1=10 ("index"), index #5=1 ("index"), index #7=7 ("index")) -> (element #1=w1638:string, element #2=w1636:string, element #3=w1635:string, element #4=w1640:string, element #5=w1618:string, element #6=w1617:string, element #7=w1604:string)  [unwired: 4 in]
              n1167 = Replace Array Subset(array=w1648, new element=w1650, index=0) -> (w1644:string[])
              n1168 = Index Array(array=w1644, index #1=10 ("index"), index #5=1 ("index"), index #7=7 ("index")) -> (element #1=w1637:string, element #2=w1634:string, element #3=w1633:string, element #4=w1639:string, element #5=w1616:string, element #6=w1615:string, element #7=w1603:string)  [unwired: 4 in]
              n1169 = Select(t="A new configuration table has been loaded.\n", s=w1656, f="") -> (s? t:f=w1626:string)
              n1170 = Not Equal?(x=w1640, y=w1639) -> (x != y?=w1641:bool)
              n1171 = Not Equal?(x=w1638, y=w1637) -> (x != y?=w1632:bool)
              n1172 = Not Equal?(x=w1618, y=w1616) -> (x != y?=w1612:bool)
              n1173 = Not Equal?(x=w1636, y=w1634) -> (x != y?=w1631:bool)
              n1174 = Not Equal?(x=w1617, y=w1615) -> (x != y?=w1609:bool)
              n1175 = Not Equal?(x=w1635, y=w1633) -> (x != y?=w1630:bool)
              n1176 = Not Equal?(x=w1604, y=w1603) -> (x != y?=w1600:bool)
              n1177 = Select(t="Pole orientation has been changed.\n", s=w1641, f="") -> (s? t:f=w1625:string)
              n1178 = Compound Arithmetic op=OR(w1632, w1631, w1630) -> (w1627:bool)
              n1179 = Select(t="Oscillator settings have been changed.\n", s=w1627, f="") -> (s? t:f=w1624:string)
              n1180 = Select(t="Serial number has been changed.\n", s=w1612, f="") -> (s? t:f=w1608:string)
              n1181 = Select(t="Model name has been changed.\n", s=w1609, f="") -> (s? t:f=w1607:string)
              n1182 = Select(t="IP address has been changed.\n", s=w1600, f="") -> (s? t:f=w1599:string)
              n1183 = Unbundle By Name(w1596) -> ("CalAjusted"=w1595:bool)
              n1184 = Select(t="Calibration tables have been adjusted.\n", s=w1595, f="") -> (s? t:f=w1594:string)
              n1185 = Concatenate Strings(w1626, w1625, w1624, w1608, w1607, w1599, w1594) -> (w1622:string)
              n1186 = Empty String/Path?(string/path=w1622) -> (empty?=w1623:bool)
              n1187 = case shown="False" w1623 {
                tunnel: w1622 -> [w1660 _]
                tunnel: [w1659 _] -> w1621
                frame False {
                  n1188 = Format Into String(format string="Do you want to keep the following changes:\n\n%s\n(Press No to revert all changes)", w1660) -> (resulting string=w1665:string)  [unwired: 2 in, 1 out]
                  n1189 = call "_Log Events.vi"("Event"=w1660, "Log Command"=_Log_Command."Write" ("File Command")) -> ("error out"=w1659:errorcluster)  [unwired: 6 in, 1 out]
                  n1190 = Two Button Dialog(message=w1665, 1:"No" ("F button name (\"Cancel\")"), 2:"Yes" ("T button name (\"OK\")")) -> (T button?=w1662:bool)
                  n1191 = case shown="False" w1662 {
                    frame False {
                      n1192 = stacked-sequence {
                        frame #0 {
                          n1193 = call <vilib>:"Set Busy.vi"() -> ()  [unwired: 4 in, 8 out]
                        }
                        frame #1 {
                          n1194 = call "_Load All Tables.vi"("Use temporary file (F)"=TRUE) -> ()  [unwired: 7 out]
                        }
                        frame #2 {
                          n1195 = Wait (ms)(milliseconds to wait=u32 1800) -> ()  [unwired: 1 out]
                        }
                        frame #3 {
                          n1196 = call <vilib>:"Unset Busy.vi"() -> ()  [unwired: 2 in, 10 out]
                        }
                      }
                    }
                    frame True {
                    }
                  }
                }
                frame True {
                }
              }
              n1197 = call "_Log Events.vi"("error in (no error)"=w1621, "Log Command"=_Log_Command."Close" ("File Command")) -> ()  [unwired: 6 in, 2 out]
            }
            frame #6 {
              w1680 = "Lens" ("section")
              n1198 = call "_Open Preference File.vi"() -> ("error"=w1689:errorcluster, "refnum"=w1690:T29)  [unwired: 3 in, 3 out]
              n1199 = local read "Oscillator Settings"() -> (w1675:string[][])
              n1200 = local read "IP Address"() -> (w1684:string)
              n1201 = global read "_Global LC Driver.vi" "LC Type"() -> (w1691:T30)
              n1202 = call-poly <vilib>:"Write Key.vi"("section"=w1680, "error in (no error)"=w1689, "value"=w1691, "key"="LCType" ("section"), "refnum"=w1690) -> ("error out"=w1685:errorcluster, "refnum out"=w1686:T29)  [unwired: 5 out]
              n1203 = call "_Save All Tables.vi"("SaveOption (Temporary File)"=T16."My Tables" ("Use temporary file (F)")) -> ()  [unwired: 2 in, 5 out]
              n1204 = call-poly <vilib>:"Write Key.vi"("section"=w1680, "error in (no error)"=w1685, "value"=w1684, "key"="UpsIP" ("section"), "refnum"=w1686) -> ("error out"=w1683:errorcluster, "refnum out"=w1687:T29)  [unwired: 1 in, 4 out]
              n1205 = Index Array(array=w1675, index (col) #1=2 ("index (row)"), index (col) #2=3 ("index (row)"), index (col) #3=4 ("index (row)"), index (col) #4=5 ("index (row)")) -> (element #1=w1673:string[], element #2=w1672:string[], element #3=w1671:string[], element #4=w1670:string[])  [unwired: 4 in]
              n1206 = Build Array(w1673, w1672, w1671, w1670) -> (w1669:string[][])
              n1207 = for {
                shift-right: [w1704] -> w1682
                shift-left: w1683 -> [w1709]
                shift-right: [w1702] -> w1681
                shift-left: w1687 -> [w1708]
                tunnel: string[] ["RefClk", "ClkMult", "FreqOut", "ScaleF"] -> [w1698] mode=indexing
                tunnel: w1669 -> [w1697] mode=indexing
                n1208 = Index Array(array=w1697) -> (element #1=w1696:string, element #2=w1695:string, element #3=w1694:string)  [unwired: 3 in]
                n1209 = call-poly <vilib>:"Write Key.vi"("section"="Oscillator0" ("key"), "error in (no error)"=w1709, "value"=w1696, "key"=w1698, "refnum"=w1708) -> ("error out"=w1707:errorcluster, "refnum out"=w1705:T29)  [unwired: 4 in, 1 out]
                n1210 = call-poly <vilib>:"Write Key.vi"("section"="Oscillator1" ("key"), "error in (no error)"=w1707, "value"=w1695, "key"=w1698, "refnum"=w1705) -> ("error out"=w1706:errorcluster, "refnum out"=w1703:T29)  [unwired: 4 in, 1 out]
                n1211 = call-poly <vilib>:"Write Key.vi"("section"="Oscillator2" ("key"), "error in (no error)"=w1706, "value"=w1694, "key"=w1698, "refnum"=w1703) -> ("error out"=w1704:errorcluster, "refnum out"=w1702:T29)  [unwired: 4 in, 1 out]
              }
              n1212 = call <vilib>:"Close Config Data.vi"("error in (no error)"=w1682, "refnum"=w1681) -> ()  [unwired: 1 in, 9 out]
            }
            frame #7 {
              n1213 = call "_Remote Communicate.vi"("DC Param"=u16 1, "Command"=_RT_Command."Ignore Error") -> ()  [unwired: 4 in, 4 out]
              n1214 = call "_Copy IPF Files.vi"() -> ()  [unwired: 1 out]
            }
          }
        }
      }
    }
    frame #1 {
      # "Hidden Controls Include:\n1. VoltageInput\n2. LoadedTable\n3. Running\n4. Quit\n5. Tune File\n6. SG Input"
      n1215 = case shown="False" w1712 {
        frame False {
          w1713 = TRUE  # release?
          n1216 = Quit LabVIEW(quit? (T)=w1713) -> ()
        }
        frame True {
        }
      }
    }
  }
  n1217 = property class="VI"(reference=w1, "Front Panel.Title"=w2) -> ()  [unwired: 1 in, 2 out]
  "Version" <- w2
